vi "EC_Applied_XYZ_MM_BR_RES_2_NC_GR_pxi_Acc3_preset.vi"() -> ()   [LabVIEW 2009]
uses:
  <vilib>/Utility/file.llb/Read From Spreadsheet File (I64).vi
  <vilib>/Utility/file.llb/Read From Spreadsheet File (string).vi
  <vilib>/Instr/_visa.llb/VISA Configure Serial Port (Instr).vi
  <vilib>/Utility/file.llb/Write To Spreadsheet File (I64).vi
  <vilib>/Utility/file.llb/Write To Spreadsheet File (string).vi
panel:
  out "R Velocity MVdeg/sec":dbl format="%.3f"
  out "R Position MV deg":dbl
  out "Z Velocity MV mm/sec":dbl format="%.3f"
  out "Z Position MV mm":dbl
  out "Y Velocity MV mm/sec":dbl format="%.3f"
  out "Y Position MV mm":dbl
  out "X Velocity MV mm/sec":dbl format="%.3f"
  out "X Position MV mm":dbl
  out "Presets":i32[][](array[numeric])
  in  "stop":bool
  in  "Tab Control 3":enum32{"Status", "Reset"}(tab)
  out "Y in Range":bool
  out "Y Scan":bool
  out "Y in Motion":bool
  out "Y Backlash corr":bool
  out "X  in Range":bool
  out "X Scan":bool
  out "X  in Motion":bool
  out "X Backlash corr":bool
  out "Z in Range":bool
  out "Z Scan":bool
  out "Z in Motion":bool
  out "Z Backlash corr":bool
  out "R in Range":bool
  out "R Scan":bool
  out "R in Motion":bool
  out "R Backlash corr":bool
  out "X Ready":bool
  out "Y Ready":bool
  out "Z Ready":bool
  out "R Ready":bool
  in  "Reset Y Position mm":dbl
  out "Reset Y Motor Steps":i32
  in  "Reset X Position mm":dbl
  out "Reset X Motor Steps":i32
  in  "Reset Z Position mm":dbl
  out "Reset Z Motor Steps":i32
  in  "Reset R Position deg":dbl
  out "Reset R Motor Steps":i32
  in  "Reset":bool
  in  "Tab Control 2":enum32{"mm", "step"}(tab)
  in  "X Scan Length SP mm":dbl
  in  "X Scan Velocity SP mm/sec":dbl
  in  "X Scan set":bool
  in  "Y Scan Length SP mm":dbl
  in  "Y Scan Velocity SP mm/sec":dbl
  in  "Y Scan set":bool
  in  "Z Scan Length SP mm":dbl
  in  "Z Scan Velocity SP mm/sec":dbl
  in  "Z Scan set":bool
  in  "R Scan Length SP deg":dbl
  in  "R Scan Velocity SP deg/sec":dbl
  in  "R Scan set":bool
  in  "X Scan Velocity SP steps/sec":i32=1 min=1 max=102400 step=1
  in  "X Scan Length SP steps":i32 min=-2304000 max=2304000 step=100
  out "X Scan length MV mm":dbl
  out "X Scan velocity MV mm/sec":dbl format="%#_6f"
  in  "Y Scan Velocity SP steps/sec":i32=1 min=1 max=102400 step=1
  in  "Y Scan Length SP steps":i32 min=-2304000 max=2304000 step=100
  out "Y Scan length MV mm":dbl
  out "Y Scan velocity MV mm/sec":dbl format="%#_6f"
  in  "Z Scan Velocity SP steps/sec":i32=1 min=1 max=102400 step=1
  in  "Z Scan Length SP steps":i32 min=-5120000 max=97280000 step=100
  out "Z Scan length MV mm":dbl
  out "Z Scan velocity MV mm/sec":dbl format="%#_6f"
  in  "R Scan Velocity SP steps/sec":i32=1 min=1 max=102400 step=1
  in  "R Scan Length SP steps":i32 min=-6144000 max=0 step=100
  out "R Scan length MV deg":dbl
  out "R Scan velocity MV deg/sec":dbl format="%#_6f"
  out "atan Y/Z":dbl
  in  "Tab Control":enum32{"mm", "preset", "step"}(tab)
  in  "X Position SP mm":dbl
  in  "X Velocity SP mm/sec":dbl
  in  "X Move Set":bool
  in  "Y Move Set":bool
  in  "Y Position SP mm":dbl
  in  "Y Velocity SP mm/sec":dbl
  in  "Z Position SP mm":dbl
  in  "Z Velocity SP mm/sec":dbl
  in  "Z Move Set":bool
  in  "R Position SP deg":dbl
  in  "R Velocity SP deg/sec":dbl
  in  "R Move Set":bool
  in  "Add Button":bool
  in  "String":string
  in  "Delete Button":bool
  in  "Preset positions":i32(ring) items=["ZERO", "Default", "CDOSE", "QMS", "test", "test2", "test3"]
  in  "Set Button":bool
  in  "X Velocity SP step/sec":i32 min=1 max=10000
  in  "Y Velocity SP step/sec":i32 min=1 max=10000
  in  "Z Velocity SP step/sec":i32 min=1 max=10000
  in  "R Velocity SP step/sec":i32 min=1 max=10000
  in  "Y Step SP":i32=-20000 min=-2304000 max=2304000 step=500
  in  "X Step SP":i32=-20000 min=-1000000 max=1000000 step=500
  in  "Z Step SP":i32=-20000 min=0 max=102400000 step=500
  in  "R Step SP":i32=-20000 min=-6144000 max=0 step=500
  out "X Step PV":i32 max=2000
  out "Y Step PV":i32 max=2000
  out "Z Step PV":i32 max=2000
  out "R Step PV":i32 max=2000
  in  "Clear ZY":bool
  out "ZY Graph":cluster{"Y":dbl[], "Y":dbl[]}[](graph)
  out "ZR Graph":cluster{"Y":dbl[], "Y":dbl[]}[](graph)
  out "XY Graph":cluster{"Y":dbl[], "Y":dbl[]}[](graph)
  out "X Scan Duration":dbl
  out "Y Scan Duration":dbl
  out "Z Scan Duration":dbl
  out "R Scan Duration":dbl
  out "R Backlash steps/sec":i32
  out "R Backlash":i32
  out "R Holding Current %":i32
  out "R Run Current %":i32
  out "R offset deg":dbl
  out "R deg/rev":dbl
  out "R steps/rev":u32
  out "R velocity PV step/sec":i32
  out "R MINPOS":i32=-94296
  out "R MAXPOS":i32=-34296
  out "R COM PORT":refnum<visa-resource-name>="COM5"
  in  "R Scan OK":bool
  in  "R Go":bool
  out "R Position deg PV":dbl
  out "Z COM PORT":refnum<visa-resource-name>="COM5"
  out "Z Backlash steps/sec":i32
  out "Z Backlash":i32
  out "Z Holding Current %":i32
  out "Z Run Current %":i32
  out "Z offset mm":dbl
  out "Z mm/rev":dbl
  out "Z steps/rev":u32
  out "Z  velocity PV step/sec":i32
  out "Z MINPOS":i32=-94296
  out "Z MAXPOS":i32=-34296
  in  "Z Scan OK":bool
  in  "Z Go":bool
  out "Z Position mm PV":dbl
  out "X Position mm PV":dbl
  out "X velocity PV step/sec":i32
  in  "X Scan OK":bool
  in  "X Go":bool
  out "X Backlash steps/sec":i32
  out "X Backlash":i32
  out "X Holding Current %":i32
  out "X Run Current %":i32
  out "X offset mm":dbl
  out "X mm/rev":dbl
  out "X steps/rev":u32
  out "X MAXPOS":i32=-34296
  out "X MINPOS":i32=-94296
  out "X COM PORT":refnum<visa-resource-name>="COM5"
  out "Y Backlash steps/sec":i32
  out "Y Backlash":i32
  out "Y Holding Current %":i32
  out "Y Run Current %":i32
  in  "Scan Cancel":bool
  out "Y Position mm PV":dbl
  out "Y offset mm":dbl
  out "Y mm/rev":dbl
  out "Y steps/rev":u32
  out "Y velocity PV step/sec":i32
  in  "Y Scan OK":bool
  in  "Scan Go":bool
  in  "Stop":bool
  in  "Y Go":bool
  out "Y MINPOS":i32=-94296
  out "Y MAXPOS":i32=-34296
  out "Y COM PORT":refnum<visa-resource-name>="COM5"
  # "Current position"
  # "Goto position"
  # "RX"
  # "RY"
  # "RZ"
  # "RR"
  # "L"
  # "M"
  # "B"
  # "S"
  # "R"
  # "Preset position"
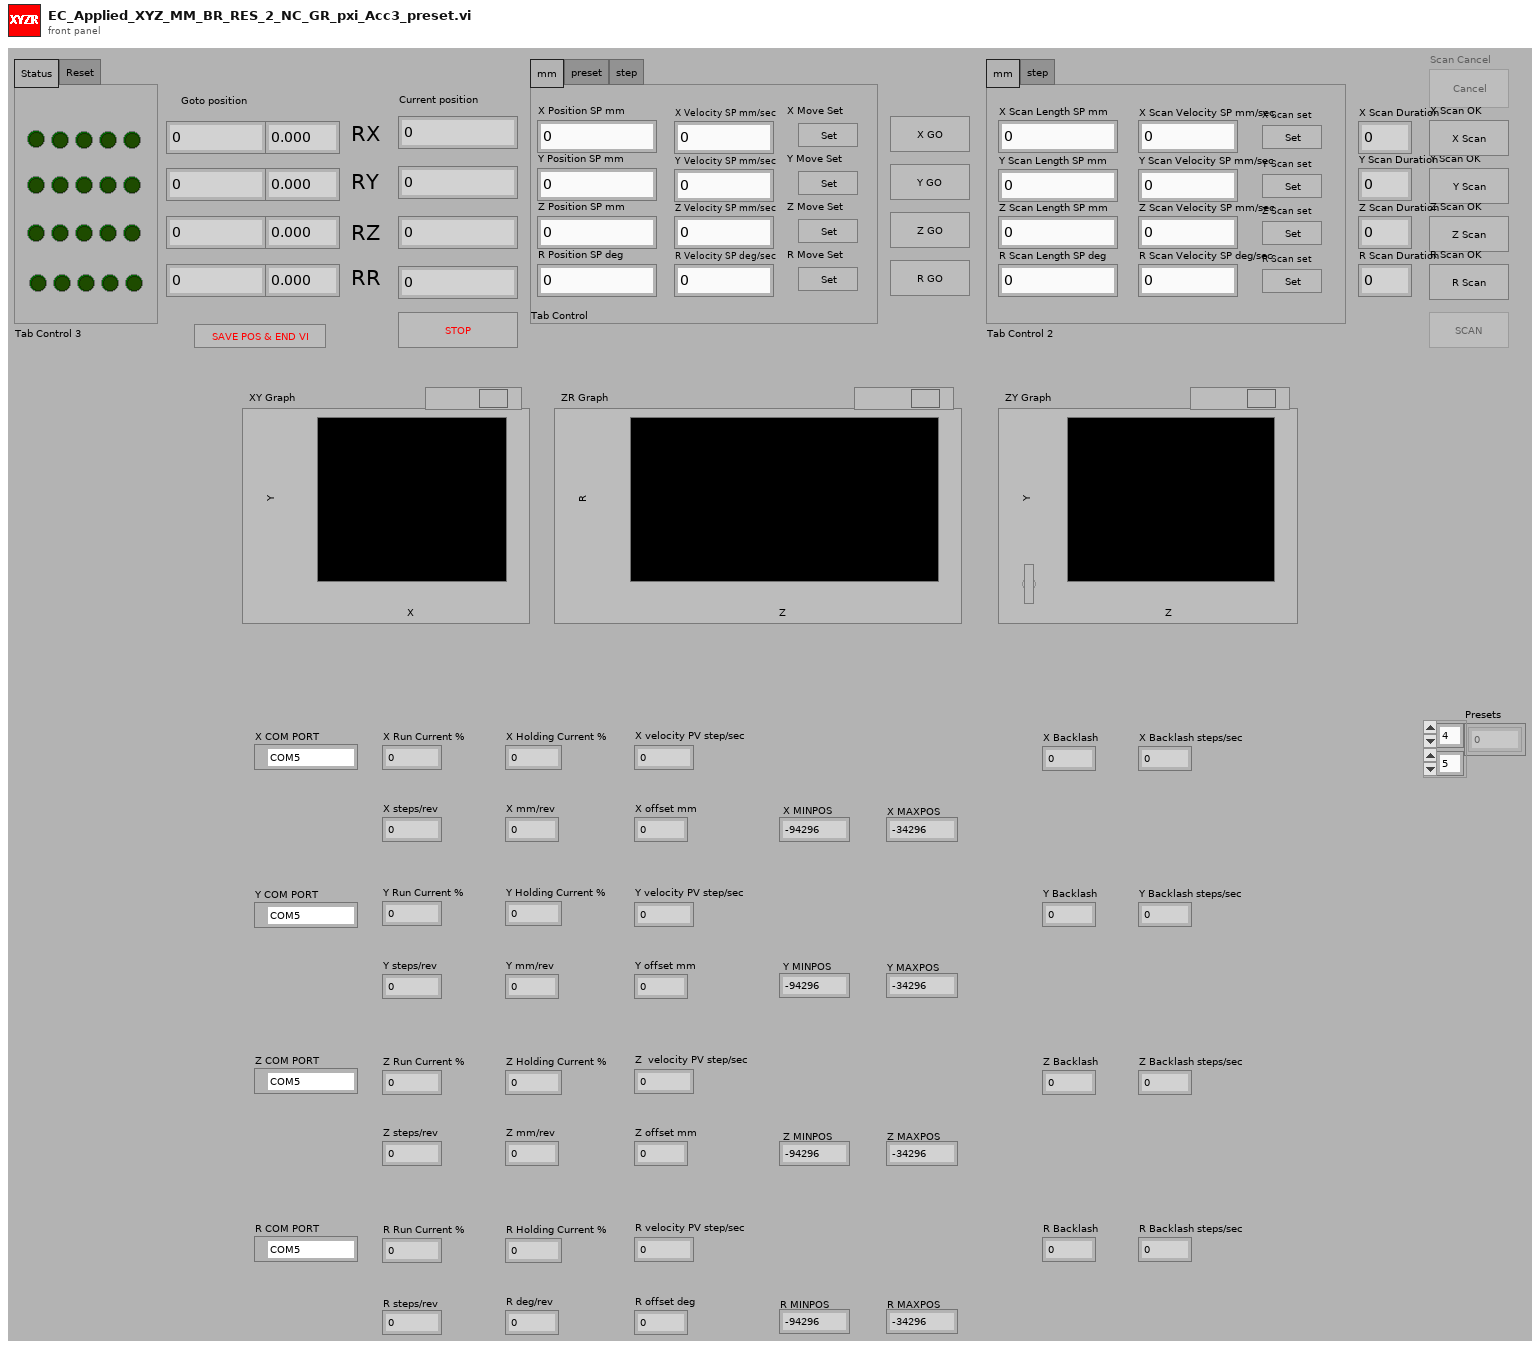
[diagram p1: front panel]
types:
  T1 = enum16{"Stop", "Reset", "Run Current", "Holding Current", "Accel Rate", "Decel Rate", "Move to Relative Position", "Move to Absolute Position", "Echo Mode", "Print Parameter", "Send String", "Microstep Resolution", "Set Current Position", "Max Velocity"}
  T2 = enum8{"Enabled", "Disabled", "Disabled and Grayed Out"}
  T3 = enum16{"Power-up Signature", "Accel Rate", "Accel Max", "Bit Rate", "Buffer Status", "Change Current", "Commence Jogging", "Change Jog Speed", "Continue", "Define Address", "Distance for FC,FM,FO,FY", "Decel Rate", "Distance or Position", "Define Limits", "Encoder Deadband", "Encoder Function", "Encoder Position", "Encoder Ratio", "Feed to Length with Speed Change", "Feed to Length", "Feed to Sensor with Mask Dist", "Feed to Length & Set Output", "Feed to Position", "Feed to Sensor", "Feed to Sensor w/safety", "Follow Handwheel", "Immediate Distance?", "Immediate Encoder?", "Immediate Low Output", "Immediate High Output", "Immediate Position?", "Input Status?", "Jog Accel/Decel", "Jog Disable", "Jog Enable", "Jog Speed", "Motor Disable", "Motor Enable", "Microstep Resolution", "Power up Current", "Power up Mode", "Pause", "Request Status", "Revision Level?", "Seek Home", "Stop Jogging", "Stop & Kill Buffer", "Set Output", "Set ABS Position", "Send String", "Stop", "Velocity for Speed Change", "Velocity Setting", "Wait for Input", "Wait Time"}
  T4 = cluster{"first row[0]":i64, "first row[1]":i64, "first row[2]":i64, "first row[3]":i64, "first row[4]":i64, "first row[5]":i64, "first row[6]":i64, "first row[7]":i64, "first row[8]":i64}
  T5 = cluster{"Value[0]":i32, "Value[1]":i32, "Value[2]":i32, "Value[3]":i32, "Value[4]":i32, "Value[5]":i32, "Value[6]":i32, "Value[7]":i32, "Value[8]":i32}
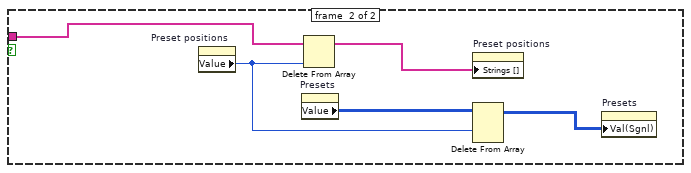
[diagram p2: hidden frame]
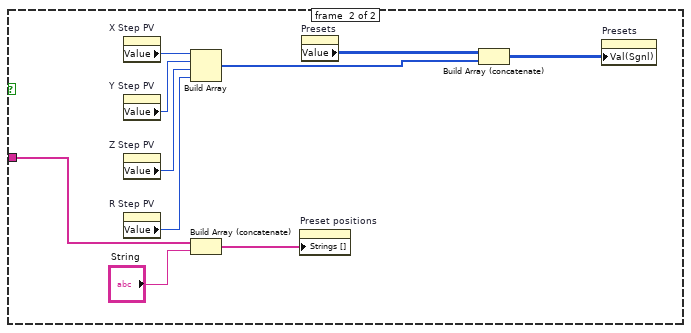
[diagram p3: hidden frame]
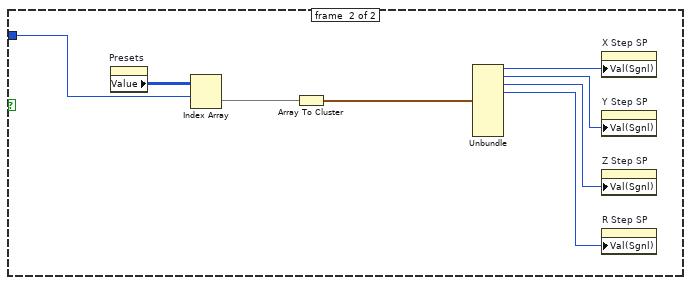
[diagram p4: hidden frame]
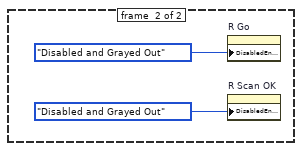
[diagram p5: hidden frame]
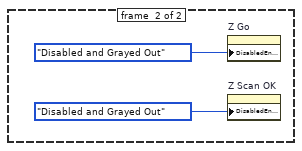
[diagram p8: hidden frame]
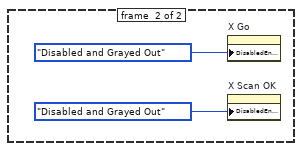
[diagram p11: hidden frame]
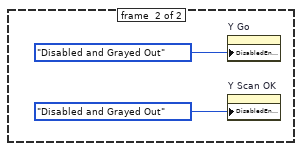
[diagram p14: hidden frame]
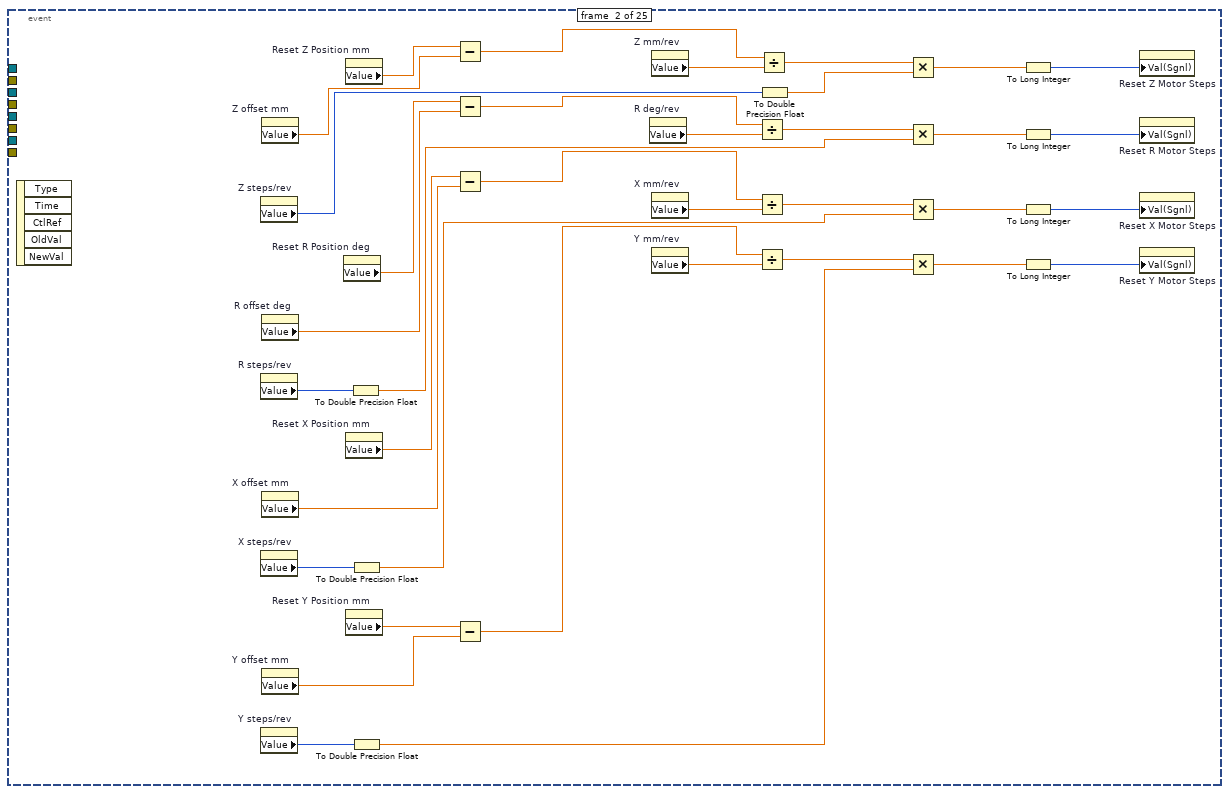
[diagram p17: hidden frame]
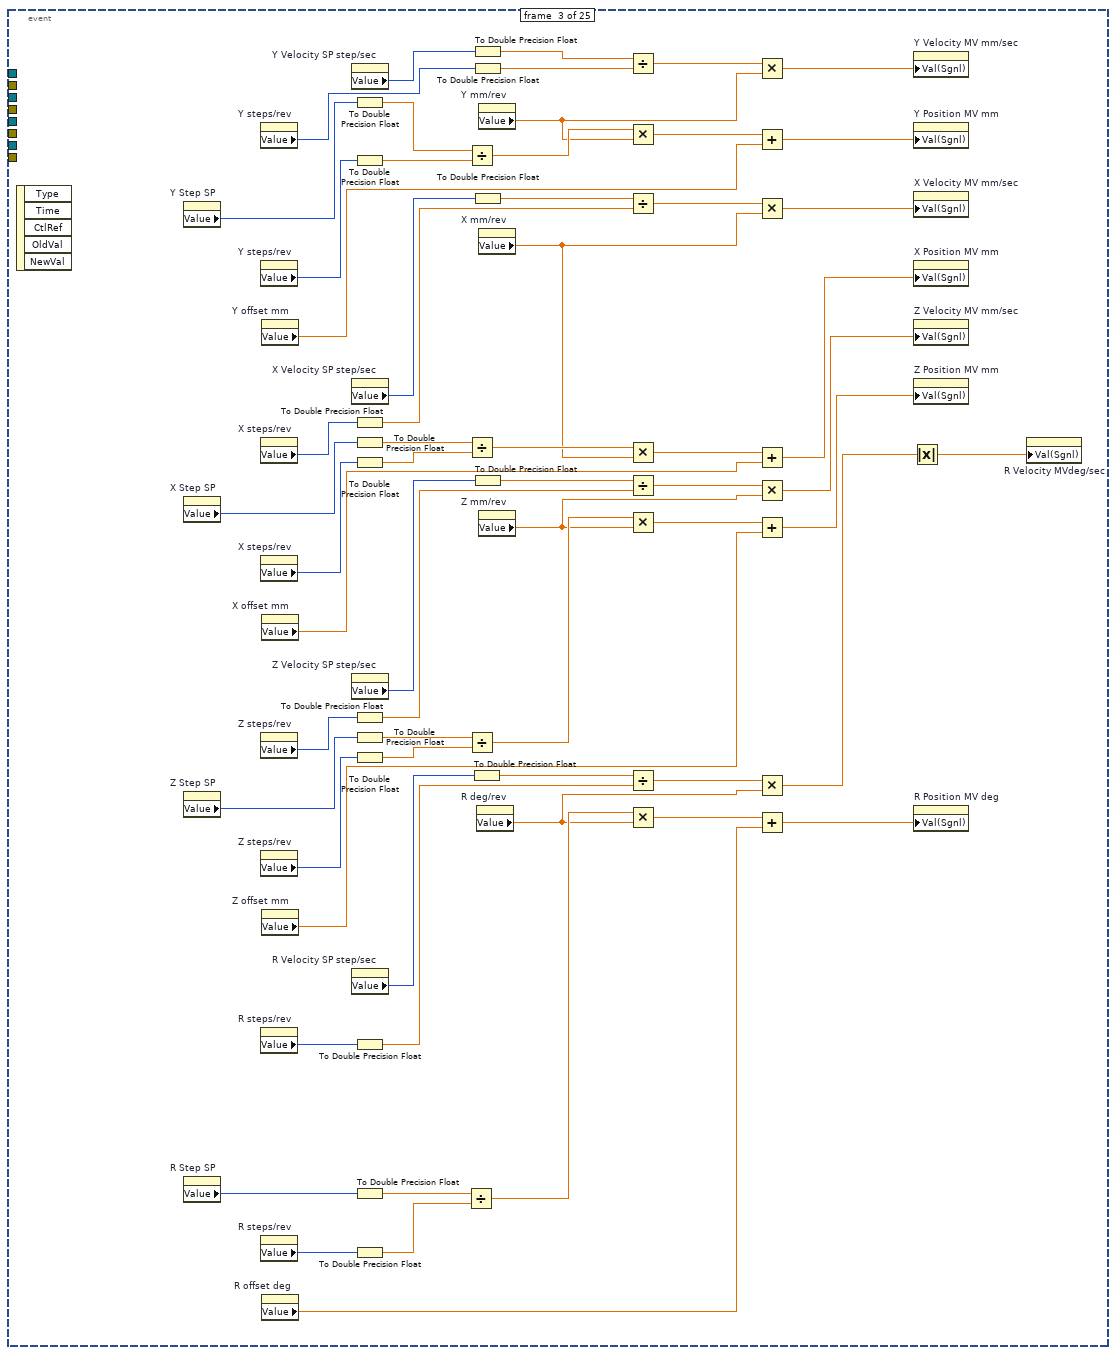
[diagram p18: hidden frame]
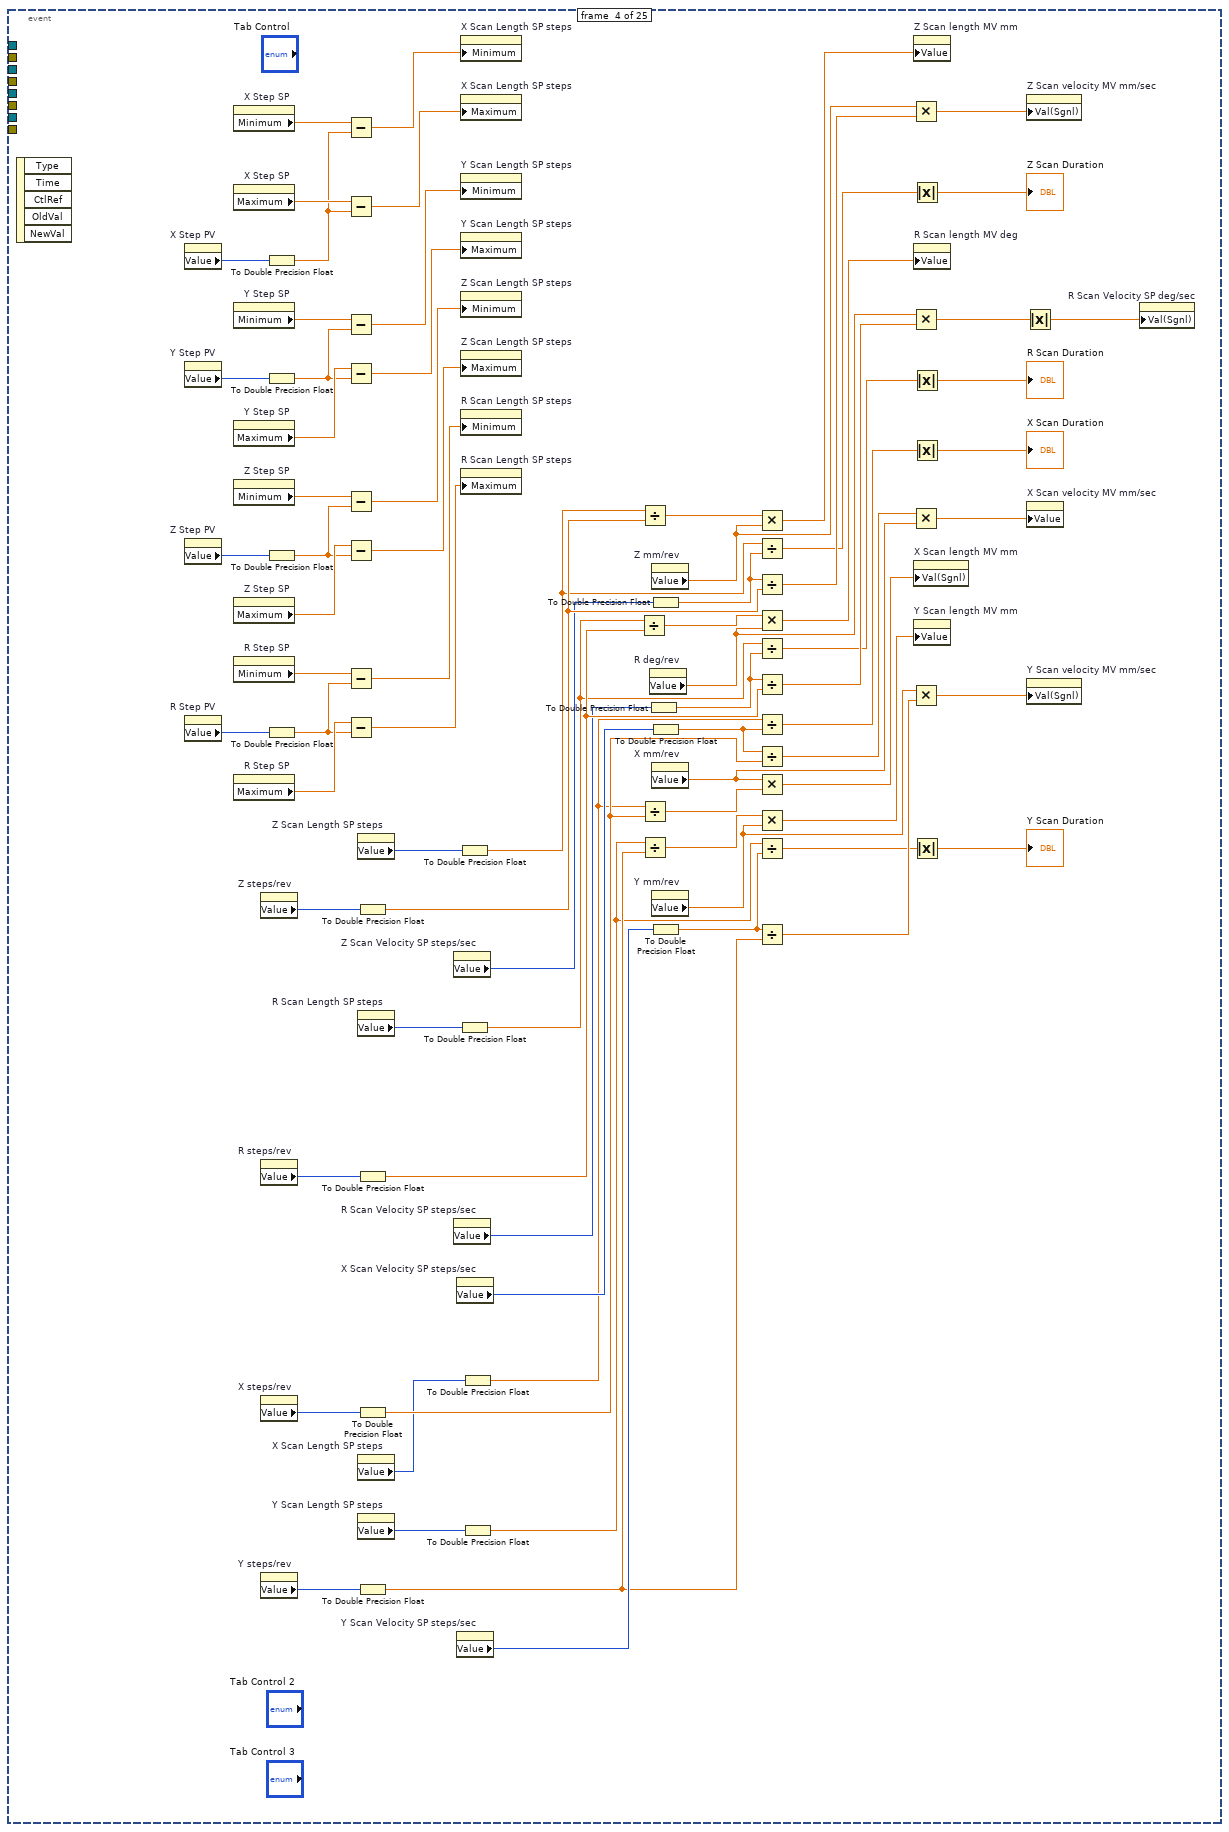
[diagram p19: hidden frame]
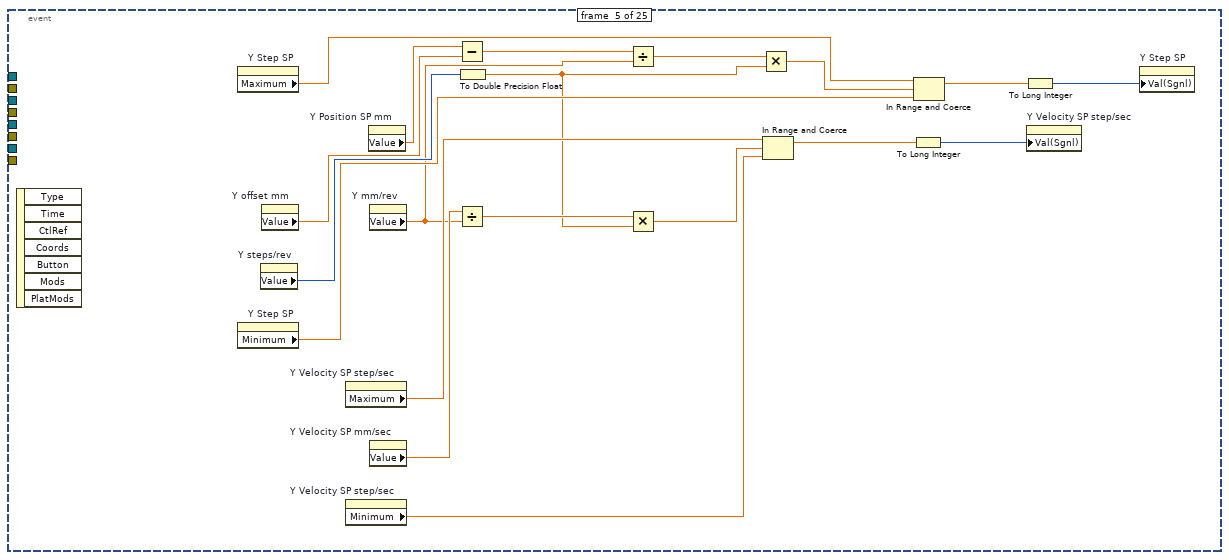
[diagram p20: hidden frame]
diagram:
  w6 = 0 ("dimension size")
  n1 = flat-sequence {
    tunnel: [w99] -> w40
    tunnel: [w98] -> w39
    tunnel: [w107] -> w56
    tunnel: [w109] -> w54
    tunnel: w40 -> [w108]
    tunnel: w39 -> [w110]
    tunnel: w56 -> [w114]
    tunnel: [w115] -> w55
    tunnel: w54 -> [w113]
    tunnel: [w116] -> w53
    tunnel: [w127] -> w69
    tunnel: [w129] -> w68
    tunnel: w55 -> [w128]
    tunnel: w53 -> [w123]
    tunnel: w69 -> [w136]
    tunnel: [w135] -> w67
    tunnel: w68 -> [w133]
    tunnel: [w134] -> w66
    tunnel: [w146] -> w65
    tunnel: [w147] -> w64
    tunnel: w67 -> [w145]
    tunnel: w66 -> [w144]
    tunnel: w65 -> [w157]
    tunnel: w64 -> [w156]
    tunnel: [w159] -> w63
    tunnel: [w158] -> w62
    tunnel: [w153] -> w61
    tunnel: [w166] -> w57
    tunnel: [w167] -> w58
    tunnel: w63 -> [w167]
    tunnel: w62 -> [w166]
    tunnel: w61 -> [w164]
    frame #0 {
      w106 = refnum<visa-resource-name> "COM11" ("COM PORT")
      w104 = u16 0 items=["None", "XON/XOFF", "RTS/CTS", "XON/XOFF & RTS/CTS", "DTR/DSR", "XON/XOFF & DTR/DSR"] ("flow control (0:none)")
      w103 = u16 10 items=["1.0"=10, "1.5"=15, "2.0"=20] ("stop bits (10: 1 bit)")
      # "Stop bits"
      n2 = call-poly "VISA Configure Serial Port"("VISA resource name"=w106, "timeout (10sec)"=u32 10000, "baud rate (9600)"=u32 9600, "data bits (8)"=u16 8, "parity (0:none)"=enum16{"None", "Odd", "Even", "Mark", "Space"}."None", "stop bits (10: 1 bit)"=w103, "flow control (0:none)"=w104) -> ("VISA resource name out"=w99:refnum<visa-resource-name>, "error out"=w98:errorcluster)  [unwired: 7 in]
      "R COM PORT" <- w106
    }
    frame #1 {
      n3 = call "mDrive Send Command.vi"("error in (no error)"=w110, "Extra"="EM=2", "Command"=T1."Send String", "VISA resource name"=w108) -> ("error out"=w109:errorcluster, "VISA resource name out"=w107:refnum<visa-resource-name>)  [unwired: 3 in, 1 out]
    }
    frame #2 {
      # "pr=1000000"
      n4 = Number To Decimal String(number=100000) -> (decimal integer string=w118:string)  [unwired: 1 in]
      n5 = call "mDrive Send Command.vi"("error in (no error)"=w113, "Extra"=w118, "Command"=T1."Accel Rate", "VISA resource name"=w114) -> ("error out"=w117:errorcluster, "VISA resource name out"=w122:refnum<visa-resource-name>)  [unwired: 3 in, 1 out]
      n6 = call "mDrive Send Command.vi"("error in (no error)"=w117, "Extra"=w118, "Command"=T1."Decel Rate", "VISA resource name"=w122) -> ("error out"=w116:errorcluster, "VISA resource name out"=w115:refnum<visa-resource-name>)  [unwired: 3 in, 1 out]
    }
    frame #3 {
      # "Run Current %"
      n7 = property on="R Run Current %" class="DigNum (strict)"() -> ("Value"=w125:i32)  [unwired: 2 in, 2 out]
      n8 = Number To Decimal String(number=w125) -> (decimal integer string=w126:string)  [unwired: 1 in]
      n9 = call "mDrive Send Command.vi"("error in (no error)"=w123, "Extra"=w126, "Command"=T1."Run Current", "VISA resource name"=w128) -> ("error out"=w129:errorcluster, "VISA resource name out"=w127:refnum<visa-resource-name>)  [unwired: 3 in, 1 out]
    }
    frame #4 {
      # "Holding Current %"
      n10 = property on="R Holding Current %" class="DigNum (strict)"() -> ("Value"=w131:i32)  [unwired: 2 in, 2 out]
      n11 = Number To Decimal String(number=w131) -> (decimal integer string=w132:string)  [unwired: 1 in]
      n12 = call "mDrive Send Command.vi"("error in (no error)"=w133, "Extra"=w132, "Command"=T1."Holding Current", "VISA resource name"=w136) -> ("error out"=w134:errorcluster, "VISA resource name out"=w135:refnum<visa-resource-name>)  [unwired: 3 in, 1 out]
    }
    frame #5 {
      # "Print Velocity Max"
      # "Velocity Max"
      n13 = property on="R Velocity SP step/sec" class="DigNum (strict)"() -> ("Value"=w143:i32)  [unwired: 2 in, 2 out]
      n14 = Number To Decimal String(number=w143) -> (decimal integer string=w142:string)  [unwired: 1 in]
      n15 = call "mDrive Send Command.vi"("error in (no error)"=w144, "Extra"=w142, "Command"=T1."Max Velocity", "VISA resource name"=w145) -> ("error out"=w140:errorcluster, "VISA resource name out"=w150:refnum<visa-resource-name>)  [unwired: 3 in, 1 out]
      n16 = call "mDrive Send Command.vi"("error in (no error)"=w140, "Extra"="VM", "Command"=T1."Print Parameter", "VISA resource name"=w150) -> ("error out"=w147:errorcluster, "read buffer"=w148:string, "VISA resource name out"=w146:refnum<visa-resource-name>)  [unwired: 3 in]
      n17 = Decimal String To Number(string=w148, offset=0) -> (number=w141:i32)  [unwired: 1 in, 1 out]
      n18 = property on="R velocity PV step/sec" class="DigNum (strict)"("Val(Sgnl)"=w141) -> ()  [unwired: 2 in, 2 out]
    }
    frame #6 {
      # "PRINT POSITION"
      n19 = call "mDrive Send Command.vi"("error in (no error)"=w156, "Extra"="P", "Command"=T1."Print Parameter", "VISA resource name"=w157) -> ("error out"=w158:errorcluster, "read buffer"=w155:string, "VISA resource name out"=w159:refnum<visa-resource-name>)  [unwired: 3 in]
      n20 = Decimal String To Number(string=w155, offset=0) -> (number=w153:i32)  [unwired: 1 in, 1 out]
    }
    frame #7 {
      n21 = property on="R Step SP" class="DigNum (strict)"("Val(Sgnl)"=w164) -> ()  [unwired: 2 in, 2 out]
      n22 = property on="R Step SP" class="DigNum (strict)"() -> ("Maximum"=w163:dbl)  [unwired: 2 in, 2 out]
      n23 = property on="R Step SP" class="DigNum (strict)"() -> ("Minimum"=w162:dbl)  [unwired: 2 in, 2 out]
      n24 = To Long Integer(number=w163) -> (32bit integer=w160:i32)
      "R MAXPOS" <- w160
      n25 = To Long Integer(number=w162) -> (32bit integer=w161:i32)
      "R MINPOS" <- w161
      n26 = In Range and Coerce(upper limit=w160, x=w164, lower limit=w161) -> (In Range?=w165:bool)  [unwired: 1 out]
      n27 = property on="R in Range" class="Bool (strict)"("Val(Sgnl)"=w165) -> ()  [unwired: 2 in, 2 out]
    }
  }
  n28 = flat-sequence {
    frame #0 {
      w173 = -3.0 ("R deg/rev")
      w171 = u32 20000 ("step/rev")
      w175 = 10000 ("Value (Signaling)")
      n29 = To Double Precision Float(number=w175) -> (double precision float=w177:dbl)
      n30 = To Double Precision Float(number=w171) -> (double precision float=w172:dbl)
      n31 = property on="R Velocity SP step/sec" class="DigNum (strict)"("Val(Sgnl)"=w175) -> ()  [unwired: 2 in, 2 out]
      n32 = property on="R Velocity SP step/sec" class="DigNum (strict)"("Minimum"=1.0 ("Data Entry Limits:Minimum")) -> ()  [unwired: 2 in, 2 out]
      n33 = Divide(x=w177, y=w172) -> (x/y=w176:dbl)
      n34 = property on="R Velocity SP step/sec" class="DigNum (strict)"("Maximum"=w177) -> ()  [unwired: 2 in, 2 out]
      n35 = Multiply(x=w176, y=w173) -> (x*y=w174:dbl)
      n36 = Absolute Value(x=w174) -> (abs(x)=w168:dbl)
      n37 = property on="R Velocity SP deg/sec" class="DigNum (strict)"("Val(Sgnl)"=w168) -> ()  [unwired: 2 in, 2 out]
      "R offset deg" <- 0.0 ("R offset deg")
      "R deg/rev" <- w173
      "R steps/rev" <- w171
    }
  }
  n38 = flat-sequence {
    frame #0 {
      w179 = 5.08 ("Z mm/rev")
      w178 = u32 20000 ("step/rev")
      w180 = 10000 ("Value (Signaling)")
      n39 = To Double Precision Float(number=w180) -> (double precision float=w184:dbl)
      n40 = To Double Precision Float(number=w178) -> (double precision float=w183:dbl)
      n41 = property on="Z Velocity SP step/sec" class="DigNum (strict)"("Val(Sgnl)"=w180) -> ()  [unwired: 2 in, 2 out]
      n42 = property on="Z Velocity SP step/sec" class="DigNum (strict)"("Minimum"=1.0 ("Data Entry Limits:Minimum")) -> ()  [unwired: 2 in, 2 out]
      n43 = Divide(x=w184, y=w183) -> (x/y=w181:dbl)
      n44 = property on="Z Velocity SP step/sec" class="DigNum (strict)"("Maximum"=w184) -> ()  [unwired: 2 in, 2 out]
      n45 = Multiply(x=w181, y=w179) -> (x*y=w182:dbl)
      n46 = property on="Z Velocity SP mm/sec" class="DigNum (strict)"("Val(Sgnl)"=w182) -> ()  [unwired: 2 in, 2 out]
      "Z offset mm" <- 0.0 ("Z offset mm")
      "Z mm/rev" <- w179
      "Z steps/rev" <- w178
    }
  }
  n47 = flat-sequence {
    frame #0 {
      n48 = property on="X Backlash corr" class="Bool (strict)"("Val(Sgnl)"=FALSE ("Value (Signaling)")) -> ()  [unwired: 2 in, 2 out]
      n49 = property on="Y Backlash corr" class="Bool (strict)"("Val(Sgnl)"=FALSE ("Value (Signaling)")) -> ()  [unwired: 2 in, 2 out]
      n50 = property on="R Backlash corr" class="Bool (strict)"("Val(Sgnl)"=FALSE ("Value (Signaling)")) -> ()  [unwired: 2 in, 2 out]
      n51 = property on="Z Backlash corr" class="Bool (strict)"("Val(Sgnl)"=FALSE ("Value (Signaling)")) -> ()  [unwired: 2 in, 2 out]
      "Z Backlash steps/sec" <- 1000 ("Z Backlash steps/sec")
      "Z Backlash" <- -12800 ("Z Backlash")
      "X Backlash steps/sec" <- 10000 ("Value (Signaling)")
      "X Backlash" <- 5000 ("Backlash2")
      "Y Backlash" <- 5120 ("Backlash2")
      "Y Backlash steps/sec" <- 1000 ("Value (Signaling)")
      "R Backlash steps/sec" <- 6400 ("R Backlash steps/sec")
      "R Backlash" <- -12800 ("R Backlash")
    }
  }
  n52 = flat-sequence {
    frame #0 {
      "Z Holding Current %" <- 50 ("Z Holding Current %")
      "Z Run Current %" <- 100 ("Z Run Current %")
      "X Run Current %" <- 100 ("Run Current %")
      "X Holding Current %" <- 50 ("Holding Current %")
      "Y Run Current %" <- 100 ("Run Current %")
      "Y Holding Current %" <- 50 ("Holding Current %")
      "R Holding Current %" <- 50 ("R Holding Current %")
      "R Run Current %" <- 100 ("R Run Current %")
    }
  }
  n53 = flat-sequence {
    frame #0 {
      n54 = property on="Y Scan" class="Bool (strict)"("Val(Sgnl)"=FALSE ("Value (Signaling)")) -> ()  [unwired: 2 in, 2 out]
      n55 = property on="X Scan Velocity SP mm/sec" class="DigNum (strict)"("Val(Sgnl)"=0.1 ("Value (Signaling)")) -> ()  [unwired: 2 in, 2 out]
      n56 = property on="Z Scan" class="Bool (strict)"("Val(Sgnl)"=FALSE ("Value (Signaling)")) -> ()  [unwired: 2 in, 2 out]
      n57 = property on="X Scan" class="Bool (strict)"("Val(Sgnl)"=FALSE ("Value (Signaling)")) -> ()  [unwired: 2 in, 2 out]
      n58 = property on="Z Scan Velocity SP mm/sec" class="DigNum (strict)"("Val(Sgnl)"=0.1 ("Value (Signaling)")) -> ()  [unwired: 2 in, 2 out]
      n59 = property on="R Velocity SP deg/sec" class="DigNum (strict)"("Val(Sgnl)"=0.1 ("Value (Signaling)")) -> ()  [unwired: 2 in, 2 out]
      n60 = property on="R Scan" class="Bool (strict)"("Val(Sgnl)"=FALSE ("Value (Signaling)")) -> ()  [unwired: 2 in, 2 out]
      n61 = property on="Y Scan Velocity SP mm/sec" class="DigNum (strict)"("Val(Sgnl)"=0.1 ("Value (Signaling)")) -> ()  [unwired: 2 in, 2 out]
      n62 = property on="Scan Go" class="Bool"("DisabledEnum"=T2."Disabled and Grayed Out" ("Disabled")) -> ()  [unwired: 2 in, 2 out]
      n63 = property on="Scan Cancel" class="Bool"("DisabledEnum"=T2."Disabled and Grayed Out" ("Disabled")) -> ()  [unwired: 2 in, 2 out]
    }
  }
  n64 = flat-sequence {
    frame #0 {
      w219 = 0.21167 ("MM/rev")
      w222 = u32 20000 ("step/rev")
      w217 = 10000 ("Value (Signaling)")
      # "a=1000000"
      n65 = property on="X Velocity SP step/sec" class="DigNum (strict)"("Minimum"=1.0 ("Data Entry Limits:Minimum")) -> ()  [unwired: 2 in, 2 out]
      n66 = To Double Precision Float(number=w217) -> (double precision float=w223:dbl)
      n67 = To Double Precision Float(number=w222) -> (double precision float=w221:dbl)
      n68 = property on="X Velocity SP step/sec" class="DigNum (strict)"("Val(Sgnl)"=w217) -> ()  [unwired: 2 in, 2 out]
      n69 = Divide(x=w223, y=w221) -> (x/y=w218:dbl)
      n70 = property on="X Velocity SP step/sec" class="DigNum (strict)"("Maximum"=w223) -> ()  [unwired: 2 in, 2 out]
      n71 = Multiply(x=w218, y=w219) -> (x*y=w220:dbl)
      n72 = property on="X Velocity SP mm/sec" class="DigNum (strict)"("Val(Sgnl)"=w220) -> ()  [unwired: 2 in, 2 out]
      "X offset mm" <- 0.0 ("offset")
      "X steps/rev" <- w222
      "X mm/rev" <- w219
    }
  }
  n73 = flat-sequence {
    frame #0 {
      w228 = 0.21167 ("MM/rev")
      w231 = u32 20000 ("step/rev")
      w226 = 10000 ("Value (Signaling)")
      n74 = To Double Precision Float(number=w226) -> (double precision float=w232:dbl)
      n75 = To Double Precision Float(number=w231) -> (double precision float=w230:dbl)
      n76 = property on="Y Velocity SP step/sec" class="DigNum (strict)"("Minimum"=1.0 ("Data Entry Limits:Minimum")) -> ()  [unwired: 2 in, 2 out]
      n77 = property on="Y Velocity SP step/sec" class="DigNum (strict)"("Val(Sgnl)"=w226) -> ()  [unwired: 2 in, 2 out]
      n78 = Divide(x=w232, y=w230) -> (x/y=w227:dbl)
      n79 = property on="Y Velocity SP step/sec" class="DigNum (strict)"("Maximum"=w232) -> ()  [unwired: 2 in, 2 out]
      n80 = Multiply(x=w227, y=w228) -> (x*y=w229:dbl)
      n81 = property on="Y Velocity SP mm/sec" class="DigNum (strict)"("Val(Sgnl)"=w229) -> ()  [unwired: 2 in, 2 out]
      "Y offset mm" <- 0.0 ("offset")
      "Y steps/rev" <- w231
      "Y mm/rev" <- w228
    }
  }
  n82 = flat-sequence {
    tunnel: [w235] -> w42
    tunnel: [w236] -> w41
    tunnel: [w246] -> w48
    tunnel: [w245] -> w46
    tunnel: w42 -> [w247]
    tunnel: w41 -> [w244]
    tunnel: w48 -> [w257]
    tunnel: [w252] -> w47
    tunnel: w46 -> [w256]
    tunnel: [w256] -> w45
    tunnel: [w261] -> w78
    tunnel: [w263] -> w77
    tunnel: w47 -> [w262]
    tunnel: w45 -> [w264]
    tunnel: w78 -> [w271]
    tunnel: [w270] -> w76
    tunnel: w77 -> [w268]
    tunnel: [w269] -> w75
    tunnel: [w281] -> w74
    tunnel: [w282] -> w73
    tunnel: w76 -> [w280]
    tunnel: w75 -> [w279]
    tunnel: w74 -> [w292]
    tunnel: w73 -> [w291]
    tunnel: [w294] -> w72
    tunnel: [w293] -> w71
    tunnel: [w288] -> w70
    tunnel: [w301] -> w59
    tunnel: [w302] -> w60
    tunnel: w72 -> [w302]
    tunnel: w71 -> [w301]
    tunnel: w70 -> [w299]
    frame #0 {
      w243 = refnum<visa-resource-name> "COM10" ("COM PORT")
      w241 = u16 0 items=["None", "XON/XOFF", "RTS/CTS", "XON/XOFF & RTS/CTS", "DTR/DSR", "XON/XOFF & DTR/DSR"] ("flow control (0:none)")
      w240 = u16 10 items=["1.0"=10, "1.5"=15, "2.0"=20] ("stop bits (10: 1 bit)")
      # "Stop bits"
      n83 = call-poly "VISA Configure Serial Port"("VISA resource name"=w243, "timeout (10sec)"=u32 10000, "baud rate (9600)"=u32 9600, "data bits (8)"=u16 8, "parity (0:none)"=enum16{"None", "Odd", "Even", "Mark", "Space"}."None", "stop bits (10: 1 bit)"=w240, "flow control (0:none)"=w241) -> ("VISA resource name out"=w235:refnum<visa-resource-name>, "error out"=w236:errorcluster)  [unwired: 7 in]
      "Z COM PORT" <- w243
    }
    frame #1 {
      n84 = call "mDrive Send Command.vi"("error in (no error)"=w244, "Extra"="EM=2", "Command"=T1."Send String", "VISA resource name"=w247) -> ("error out"=w245:errorcluster, "VISA resource name out"=w246:refnum<visa-resource-name>)  [unwired: 3 in, 1 out]
    }
    frame #2 {
      n85 = Number To Decimal String(number=1000000) -> (decimal integer string=w250:string)  [unwired: 1 in]
      n86 = call "mDrive Send Command.vi"("Extra"=w250, "Command"=T1."Accel Rate", "VISA resource name"=w257) -> ("VISA resource name out"=w255:refnum<visa-resource-name>)  [unwired: 4 in, 2 out]
      n87 = call "mDrive Send Command.vi"("Extra"=w250, "Command"=T1."Decel Rate", "VISA resource name"=w255) -> ("VISA resource name out"=w252:refnum<visa-resource-name>)  [unwired: 4 in, 2 out]
    }
    frame #3 {
      # "Run Current %"
      n88 = property on="Z Run Current %" class="DigNum (strict)"() -> ("Value"=w259:i32)  [unwired: 2 in, 2 out]
      n89 = Number To Decimal String(number=w259) -> (decimal integer string=w260:string)  [unwired: 1 in]
      n90 = call "mDrive Send Command.vi"("error in (no error)"=w264, "Extra"=w260, "Command"=T1."Run Current", "VISA resource name"=w262) -> ("error out"=w263:errorcluster, "VISA resource name out"=w261:refnum<visa-resource-name>)  [unwired: 3 in, 1 out]
    }
    frame #4 {
      # "Holding Current %"
      n91 = property on="Z Run Current %" class="DigNum (strict)"() -> ("Value"=w266:i32)  [unwired: 2 in, 2 out]
      n92 = Number To Decimal String(number=w266) -> (decimal integer string=w267:string)  [unwired: 1 in]
      n93 = call "mDrive Send Command.vi"("error in (no error)"=w268, "Extra"=w267, "Command"=T1."Holding Current", "VISA resource name"=w271) -> ("error out"=w269:errorcluster, "VISA resource name out"=w270:refnum<visa-resource-name>)  [unwired: 3 in, 1 out]
    }
    frame #5 {
      # "Velocity Max"
      n94 = property on="Z Velocity SP step/sec" class="DigNum (strict)"() -> ("Value"=w278:i32)  [unwired: 2 in, 2 out]
      n95 = Number To Decimal String(number=w278) -> (decimal integer string=w277:string)  [unwired: 1 in]
      n96 = call "mDrive Send Command.vi"("error in (no error)"=w279, "Extra"=w277, "Command"=T1."Max Velocity", "VISA resource name"=w280) -> ("error out"=w275:errorcluster, "VISA resource name out"=w285:refnum<visa-resource-name>)  [unwired: 3 in, 1 out]
      n97 = call "mDrive Send Command.vi"("error in (no error)"=w275, "Extra"="VM", "Command"=T1."Print Parameter", "VISA resource name"=w285) -> ("error out"=w282:errorcluster, "read buffer"=w283:string, "VISA resource name out"=w281:refnum<visa-resource-name>)  [unwired: 3 in]
      n98 = Decimal String To Number(string=w283, offset=0) -> (number=w276:i32)  [unwired: 1 in, 1 out]
      n99 = property on="Z  velocity PV step/sec" class="DigNum (strict)"("Val(Sgnl)"=w276) -> ()  [unwired: 2 in, 2 out]
    }
    frame #6 {
      # "PRINT POSITION"
      n100 = call "mDrive Send Command.vi"("error in (no error)"=w291, "Extra"="P", "Command"=T1."Print Parameter", "VISA resource name"=w292) -> ("error out"=w293:errorcluster, "read buffer"=w290:string, "VISA resource name out"=w294:refnum<visa-resource-name>)  [unwired: 3 in]
      n101 = Decimal String To Number(string=w290, offset=0) -> (number=w288:i32)  [unwired: 1 in, 1 out]
    }
    frame #7 {
      n102 = property on="Z Step SP" class="DigNum (strict)"("Val(Sgnl)"=w299) -> ()  [unwired: 2 in, 2 out]
      n103 = property on="Z Step SP" class="DigNum (strict)"() -> ("Maximum"=w296:dbl)  [unwired: 2 in, 2 out]
      n104 = property on="Z Step SP" class="DigNum (strict)"() -> ("Minimum"=w298:dbl)  [unwired: 2 in, 2 out]
      n105 = To Long Integer(number=w296) -> (32bit integer=w297:i32)
      "Z MAXPOS" <- w297
      n106 = To Long Integer(number=w298) -> (32bit integer=w295:i32)
      "Z MINPOS" <- w295
      n107 = In Range and Coerce(upper limit=w297, x=w299, lower limit=w295) -> (In Range?=w300:bool)  [unwired: 1 out]
      n108 = property on="Z in Range" class="Bool (strict)"("Val(Sgnl)"=w300) -> ()  [unwired: 2 in, 2 out]
    }
  }
  n109 = flat-sequence {
    tunnel: [w304] -> w38
    tunnel: [w303] -> w37
    tunnel: [w314] -> w52
    tunnel: [w312] -> w50
    tunnel: w38 -> [w315]
    tunnel: w37 -> [w313]
    tunnel: w52 -> [w321]
    tunnel: [w322] -> w51
    tunnel: w50 -> [w318]
    tunnel: [w320] -> w49
    tunnel: [w331] -> w93
    tunnel: [w333] -> w91
    tunnel: w51 -> [w332]
    tunnel: w49 -> [w334]
    tunnel: w93 -> [w341]
    tunnel: [w340] -> w92
    tunnel: w91 -> [w338]
    tunnel: [w339] -> w90
    tunnel: [w351] -> w95
    tunnel: [w352] -> w94
    tunnel: w92 -> [w350]
    tunnel: w90 -> [w349]
    tunnel: w95 -> [w362]
    tunnel: w94 -> [w361]
    tunnel: [w364] -> w84
    tunnel: [w363] -> w83
    tunnel: [w358] -> w82
    tunnel: [w369] -> w96
    tunnel: [w370] -> w97
    tunnel: w84 -> [w370]
    tunnel: w83 -> [w369]
    tunnel: w82 -> [w365]
    frame #0 {
      w311 = refnum<visa-resource-name> "COM9" ("COM PORT")
      w309 = u16 0 items=["None", "XON/XOFF", "RTS/CTS", "XON/XOFF & RTS/CTS", "DTR/DSR", "XON/XOFF & DTR/DSR"] ("flow control (0:none)")
      w308 = u16 10 items=["1.0"=10, "1.5"=15, "2.0"=20] ("stop bits (10: 1 bit)")
      # "Stop bits"
      n110 = call-poly "VISA Configure Serial Port"("VISA resource name"=w311, "timeout (10sec)"=u32 10000, "baud rate (9600)"=u32 9600, "data bits (8)"=u16 8, "parity (0:none)"=enum16{"None", "Odd", "Even", "Mark", "Space"}."None", "stop bits (10: 1 bit)"=w308, "flow control (0:none)"=w309) -> ("VISA resource name out"=w304:refnum<visa-resource-name>, "error out"=w303:errorcluster)  [unwired: 7 in]
      "Y COM PORT" <- w311
    }
    frame #1 {
      n111 = call "mDrive Send Command.vi"("error in (no error)"=w313, "Extra"="EM=2", "Command"=T1."Send String", "VISA resource name"=w315) -> ("error out"=w312:errorcluster, "VISA resource name out"=w314:refnum<visa-resource-name>)  [unwired: 3 in, 1 out]
    }
    frame #2 {
      n112 = Number To Decimal String(number=1000000) -> (decimal integer string=w323:string)  [unwired: 1 in]
      n113 = call "mDrive Send Command.vi"("error in (no error)"=w318, "Extra"=w323, "Command"=T1."Accel Rate", "VISA resource name"=w321) -> ("error out"=w319:errorcluster, "VISA resource name out"=w327:refnum<visa-resource-name>)  [unwired: 3 in, 1 out]
      n114 = call "mDrive Send Command.vi"("error in (no error)"=w319, "Extra"=w323, "Command"=T1."Decel Rate", "VISA resource name"=w327) -> ("error out"=w320:errorcluster, "VISA resource name out"=w322:refnum<visa-resource-name>)  [unwired: 3 in, 1 out]
    }
    frame #3 {
      # "Run Current %"
      n115 = property on="Y Run Current %" class="DigNum (strict)"() -> ("Value"=w329:i32)  [unwired: 2 in, 2 out]
      n116 = Number To Decimal String(number=w329) -> (decimal integer string=w330:string)  [unwired: 1 in]
      n117 = call "mDrive Send Command.vi"("error in (no error)"=w334, "Extra"=w330, "Command"=T1."Run Current", "VISA resource name"=w332) -> ("error out"=w333:errorcluster, "VISA resource name out"=w331:refnum<visa-resource-name>)  [unwired: 3 in, 1 out]
    }
    frame #4 {
      # "Holding Current %"
      n118 = property on="Y Holding Current %" class="DigNum (strict)"() -> ("Value"=w336:i32)  [unwired: 2 in, 2 out]
      n119 = Number To Decimal String(number=w336) -> (decimal integer string=w337:string)  [unwired: 1 in]
      n120 = call "mDrive Send Command.vi"("error in (no error)"=w338, "Extra"=w337, "Command"=T1."Holding Current", "VISA resource name"=w341) -> ("error out"=w339:errorcluster, "VISA resource name out"=w340:refnum<visa-resource-name>)  [unwired: 3 in, 1 out]
    }
    frame #5 {
      # "Velocity Max"
      n121 = property on="Y Velocity SP step/sec" class="DigNum (strict)"() -> ("Value"=w348:i32)  [unwired: 2 in, 2 out]
      n122 = Number To Decimal String(number=w348) -> (decimal integer string=w347:string)  [unwired: 1 in]
      n123 = call "mDrive Send Command.vi"("error in (no error)"=w349, "Extra"=w347, "Command"=T1."Max Velocity", "VISA resource name"=w350) -> ("error out"=w345:errorcluster, "VISA resource name out"=w355:refnum<visa-resource-name>)  [unwired: 3 in, 1 out]
      n124 = call "mDrive Send Command.vi"("error in (no error)"=w345, "Extra"="VM", "Command"=T1."Print Parameter", "VISA resource name"=w355) -> ("error out"=w352:errorcluster, "read buffer"=w353:string, "VISA resource name out"=w351:refnum<visa-resource-name>)  [unwired: 3 in]
      n125 = Decimal String To Number(string=w353, offset=0) -> (number=w346:i32)  [unwired: 1 in, 1 out]
      n126 = property on="Y scan velocity MV step/sec" class="DigNum (strict)"("Val(Sgnl)"=w346) -> ()  [unwired: 2 in, 2 out]
    }
    frame #6 {
      # "PRINT POSITION"
      n127 = call "mDrive Send Command.vi"("error in (no error)"=w361, "Extra"="P", "Command"=T1."Print Parameter", "VISA resource name"=w362) -> ("error out"=w363:errorcluster, "read buffer"=w360:string, "VISA resource name out"=w364:refnum<visa-resource-name>)  [unwired: 3 in]
      n128 = Decimal String To Number(string=w360, offset=0) -> (number=w358:i32)  [unwired: 1 in, 1 out]
    }
    frame #7 {
      w367 = -2304000 ("lower limit")
      w368 = 2304000 ("upper limit")
      n129 = property on="Y Step SP" class="DigNum (strict)"("Val(Sgnl)"=w365) -> ()  [unwired: 2 in, 2 out]
      n130 = property on="Y Step SP" class="DigNum (strict)"("Maximum"=w368) -> ()  [unwired: 2 in, 2 out]
      n131 = property on="Y Step SP" class="DigNum (strict)"("Minimum"=w367) -> ()  [unwired: 2 in, 2 out]
      n132 = In Range and Coerce(upper limit=w368, x=w365, lower limit=w367) -> (In Range?=w366:bool)  [unwired: 1 out]
      n133 = property on="Y in Range" class="Bool (strict)"("Val(Sgnl)"=w366) -> ()  [unwired: 2 in, 2 out]
      "Y MINPOS" <- w367
      "Y MAXPOS" <- w368
    }
  }
  n134 = property on="Z Step SP" class="DigNum (strict)"("Minimum"=0 ("lower limit")) -> ()  [unwired: 2 in, 2 out]
  n135 = property on="R Step SP" class="DigNum (strict)"("Maximum"=0 ("upper limit")) -> ()  [unwired: 2 in, 2 out]
  n136 = flat-sequence {
    tunnel: [w372] -> w5
    tunnel: [w371] -> w4
    tunnel: w5 -> [w387]
    tunnel: w4 -> [w386]
    tunnel: [w385] -> w3
    tunnel: [w384] -> w2
    tunnel: [w390] -> w89
    tunnel: w3 -> [w398]
    tunnel: w2 -> [w397]
    tunnel: [w391] -> w1
    tunnel: w89 -> [w412]
    tunnel: [w411] -> w81
    tunnel: [w409] -> w80
    tunnel: [w414] -> w79
    tunnel: w1 -> [w413]
    tunnel: [w423] -> w87
    tunnel: [w424] -> w88
    tunnel: w81 -> [w424]
    tunnel: w80 -> [w423]
    tunnel: w79 -> [w419]
    frame #0 {
      w379 = refnum<visa-resource-name> "COM8" ("COM PORT")
      w377 = u16 0 items=["None", "XON/XOFF", "RTS/CTS", "XON/XOFF & RTS/CTS", "DTR/DSR", "XON/XOFF & DTR/DSR"] ("flow control (0:none)")
      w376 = u16 10 items=["1.0"=10, "1.5"=15, "2.0"=20] ("stop bits (10: 1 bit)")
      # "Stop bits"
      n137 = call-poly "VISA Configure Serial Port"("VISA resource name"=w379, "timeout (10sec)"=u32 10000, "baud rate (9600)"=u32 9600, "data bits (8)"=u16 8, "parity (0:none)"=enum16{"None", "Odd", "Even", "Mark", "Space"}."None", "stop bits (10: 1 bit)"=w376, "flow control (0:none)"=w377) -> ("VISA resource name out"=w372:refnum<visa-resource-name>, "error out"=w371:errorcluster)  [unwired: 7 in]
      "X COM PORT" <- w379
    }
    frame #1 {
      n138 = property on="X Run Current" class="DigNum (strict)"() -> ("Value"=w380:i32)  [unwired: 2 in, 2 out]
      n139 = Divide(x=w380, y=3.5) -> (x/y=w382:dbl)
      n140 = Number To Fractional String(number=w382) -> (F-format string=w383:string)  [unwired: 3 in]
      n141 = call "Applied Send Command.vi"("error in (no error)"=w386, "Extra"=w383, "Command"=T3."Change Current", "VISA resource name"=w387) -> ("error out"=w385:errorcluster, "VISA resource name out"=w384:refnum<visa-resource-name>)  [unwired: 3 in, 1 out]
    }
    frame #2 {
      # "VELOCITY"
      n142 = property on="X Velocity SP step/sec" class="DigNum (strict)"() -> ("Value"=w394:i32)  [unwired: 2 in, 2 out]
      n143 = property on="X steps/rev" class="DigNum (strict)"() -> ("Value"=w393:u32)  [unwired: 2 in, 2 out]
      n144 = Divide(x=w394, y=w393) -> (x/y=w392:dbl)
      n145 = Number To Fractional String(number=w392) -> (F-format string=w399:string)  [unwired: 3 in]
      n146 = call "Applied Send Command.vi"("error in (no error)"=w398, "Extra"=w399, "Command"=T3."Velocity Setting", "VISA resource name"=w397) -> ("error out"=w400:errorcluster, "VISA resource name out"=w407:refnum<visa-resource-name>)  [unwired: 3 in, 1 out]
      n147 = call "Time Delay30"("error in (no error)"=w400, "Delay Time (s)"=0.5) -> ("error out"=w405:errorcluster)  [unwired: 9 in]
      n148 = call "Applied Send Command.vi"("error in (no error)"=w405, "Extra"="", "Command"=T3."Velocity Setting", "VISA resource name"=w407) -> ("error out"=w390:errorcluster, "read buffer"=w403:string, "VISA resource name out"=w391:refnum<visa-resource-name>)  [unwired: 3 in]
      n149 = Fract/Exp String To Number(string=w403, offset=3) -> (number=w396:dbl)  [unwired: 2 in, 1 out]
      n150 = Multiply(x=w396, y=w393) -> (x*y=w395:dbl)
      n151 = property on="X velocity PV step/sec" class="DigNum (strict)"("Val(Sgnl)"=w395) -> ()  [unwired: 2 in, 2 out]
    }
    frame #3 {
      # "GET CURRENT POSITION"
      n152 = call "Applied Send Command.vi"("error in (no error)"=w412, "Extra"="", "Command"=T3."Immediate Position?", "VISA resource name"=w413) -> ("error out"=w410:errorcluster, "read buffer"=w416:string, "VISA resource name out"=w411:refnum<visa-resource-name>)  [unwired: 3 in]
      n153 = call "Time Delay13"("error in (no error)"=w410, "Delay Time (s)"=0.2) -> ("error out"=w409:errorcluster)  [unwired: 9 in]
      n154 = Hexadecimal String To Number(string=w416, offset=3) -> (number=w414:u32)  [unwired: 1 in, 1 out]
    }
    frame #4 {
      w421 = -500000 ("lower limit")
      w422 = 500000 ("upper limit")
      n155 = property on="X Step SP" class="DigNum (strict)"("Val(Sgnl)"=w419) -> ()  [unwired: 2 in, 2 out]
      n156 = property on="X Step SP" class="DigNum (strict)"("Maximum"=w422) -> ()  [unwired: 2 in, 2 out]
      n157 = In Range and Coerce(upper limit=w422, x=w419, lower limit=w421) -> (In Range?=w420:bool)  [unwired: 1 out]
      n158 = property on="X Step SP" class="DigNum (strict)"("Minimum"=w421) -> ()  [unwired: 2 in, 2 out]
      n159 = property on="X  in Range" class="Bool (strict)"("Val(Sgnl)"=w420) -> ()  [unwired: 2 in, 2 out]
      "X MINPOS" <- w421
      "X MAXPOS" <- w422
    }
  }
  n160 = property on="R Step SP" class="DigNum (strict)"("Minimum"=-6144000 ("lower limit")) -> ()  [unwired: 2 in, 2 out]
  n161 = property on="Z Step SP" class="DigNum (strict)"("Maximum"=102400000 ("upper limit")) -> ()  [unwired: 2 in, 2 out]
  n162 = call-poly <vilib>:"Read From Spreadsheet File.vi"("file path (dialog if empty)"=path "S:/LV codes/SCL2/POS.TXT") -> ("first row"=w24:i64[])  [unwired: 6 in, 4 out]
  n163 = call-poly <vilib>:"Read From Spreadsheet File.vi"("file path (dialog if empty)"=path "S:/LV codes/SCL2/PRESET.TXT") -> ("all rows"=w12:string[][])  [unwired: 6 in, 4 out]
  n164 = Array To Cluster(array=w24) -> (cluster=w23:T4)
  n165 = Transpose 2D Array(2D array=w12) -> (transposed array=w13:string[][])
  n166 = Unbundle(w23) -> ("first row[0]"=w21:i64, "first row[1]"=w20:i64, "first row[2]"=w19:i64, "first row[3]"=w18:i64)  [unwired: 5 out]
  n167 = Delete From Array(array=w13, index (row)=0) -> (deleted portion=w14:string[], array with subset deleted=w16:string[][])  [unwired: 2 in]
  n168 = property on="Reset X Motor Steps" class="DigNum (strict)"("Val(Sgnl)"=w21) -> ()  [unwired: 2 in, 2 out]
  n169 = property on="Reset Y Motor Steps" class="DigNum (strict)"("Val(Sgnl)"=w20) -> ()  [unwired: 2 in, 2 out]
  n170 = property on="Reset Z Motor Steps" class="DigNum (strict)"("Val(Sgnl)"=w19) -> ()  [unwired: 2 in, 2 out]
  n171 = property on="Reset R Motor Steps" class="DigNum (strict)"("Val(Sgnl)"=w18) -> ()  [unwired: 2 in, 2 out]
  n172 = Transpose 2D Array(2D array=w16) -> (transposed array=w17:string[][])
  n173 = property on="Preset positions" class="Ring (strict)"("Strings []"=w14) -> ()  [unwired: 2 in, 2 out]
  n174 = Decimal String To Number(string=w17) -> (number=w15:i32[][])  [unwired: 2 in, 1 out]
  n175 = Initialize Array(w6, w6, 4 ("dimension size")) -> (w9:i32[][])
  n176 = Build Array (concatenate)(w9, w15) -> (→"Presets":i32[][])
  n177 = while {
    tunnel: w97 -> [w443]
    tunnel: w96 -> [w446]
    tunnel: [w447] -> w31
    tunnel: [w445] -> w32
    tunnel: w88 -> [w442]
    tunnel: w87 -> [w441]
    tunnel: [w440] -> w86
    tunnel: [w439] -> w85
    tunnel: w60 -> [w438]
    tunnel: w59 -> [w437]
    tunnel: [w436] -> w34
    tunnel: [w435] -> w33
    tunnel: w58 -> [w434]
    tunnel: w57 -> [w433]
    tunnel: [w432] -> w30
    tunnel: [w431] -> w29
    stop <- "stop" stop-if-true
    n178 = property on="Preset positions" class="Ring (strict)"() -> ("Strings []"=w427:string[])  [unwired: 2 in, 2 out]
    n179 = event shown="[0] Timeout" {
      selector: _ -> [_ _ _ _ _ _ _ _ _ _ _ _ _ _ _ _ _ _ _ _ _ _ _ _ _]
      dyn-events: _ -> [_ _ _ _ _ _ _ _ _ _ _ _ _ _ _ _ _ _ _ _ _ _ _ _ _]
      timeout: 200 -> [_ _ _ _ _ _ _ _ _ _ _ _ _ _ _ _ _ _ _ _ _ _ _ _ _]
      tunnel: w446 -> [w548 _ _ _ _ _ _ _ _ _ _ _ w1360 _ _ _ _ w1622 _ _ w1717 w1733 w1777 w1854 w2096]
      tunnel: [w547 _ _ _ _ _ _ _ _ _ _ _ w1366 _ _ _ _ w1620 _ _ w1717 w1731 w1779 w1843 w2094] -> w447
      tunnel: w443 -> [w486 _ _ _ _ _ _ _ _ _ _ _ w1361 _ _ _ _ w1621 _ _ w1718 w1734 w1778 w1856 w2097]
      tunnel: [w546 _ _ _ _ _ _ _ _ _ _ _ w1367 _ _ _ _ w1617 _ _ w1718 w1732 w1780 w1844 w2095] -> w445
      tunnel: w442 -> [w485 _ _ _ _ _ _ _ _ _ _ _ _ _ _ w1524 w1584 _ _ _ _ w1728 w1770 w1860 w2093]
      tunnel: w441 -> [w523 _ _ _ _ _ _ _ _ _ _ _ _ _ _ w1523 w1583 _ _ _ _ w1727 w1769 w1858 w2092]
      tunnel: [w522 _ _ _ _ _ _ _ _ _ _ _ _ _ _ w1522 w1582 _ _ _ _ w1730 w1768 w1836 w2091] -> w440
      tunnel: [w521 _ _ _ _ _ _ _ _ _ _ _ _ _ _ w1521 w1581 _ _ _ _ w1729 w1767 w1834 w2090] -> w439
      tunnel: w438 -> [w495 _ _ _ _ _ _ _ _ _ _ _ _ w1412 _ _ _ _ w1652 _ _ w1726 w1764 w1852 w2089]
      tunnel: w437 -> [w498 _ _ _ _ _ _ _ _ _ _ _ _ w1411 _ _ _ _ w1651 _ _ w1725 w1763 w1850 w2088]
      tunnel: [w497 _ _ _ _ _ _ _ _ _ _ _ _ w1409 _ _ _ _ w1649 _ _ w1724 w1762 w1842 w2085] -> w436
      tunnel: [w496 _ _ _ _ _ _ _ _ _ _ _ _ w1410 _ _ _ _ w1650 _ _ w1723 w1761 w1841 w2084] -> w435
      tunnel: w434 -> [w494 _ _ _ _ _ _ _ _ _ _ _ _ _ w1465 _ _ _ _ w1686 _ w1722 w1758 w1847 w2087]
      tunnel: w433 -> [w493 _ _ _ _ _ _ _ _ _ _ _ _ _ w1464 _ _ _ _ w1685 _ w1721 w1757 w1845 w2086]
      tunnel: [w492 _ _ _ _ _ _ _ _ _ _ _ _ _ w1462 _ _ _ _ w1684 _ w1720 w1756 w1839 w2083] -> w432
      tunnel: [w491 _ _ _ _ _ _ _ _ _ _ _ _ _ w1463 _ _ _ _ w1683 _ w1719 w1755 w1838 w2082] -> w431
      event #0 {
        n180 = event-data() -> ()  [unwired: 1 in, 2 out]
        n181 = flat-sequence {
          tunnel: [w815] -> w534
          tunnel: [w826] -> w533
          tunnel: [w837] -> w532
          tunnel: [w811] -> w531
          tunnel: w485 -> [w822]
          tunnel: w523 -> [w810]
          tunnel: w534 -> [w848]
          tunnel: [w848] -> w530
          tunnel: w533 -> [w847]
          tunnel: [w847] -> w529
          tunnel: w532 -> [w846]
          tunnel: [w846] -> w528
          tunnel: w531 -> [w843]
          tunnel: [w843] -> w527
          tunnel: w530 -> [w857]
          tunnel: [w854] -> w526
          tunnel: w529 -> [w856]
          tunnel: [w855] -> w525
          tunnel: w528 -> [w853]
          tunnel: [w858] -> w524
          tunnel: w527 -> [w858]
          tunnel: w526 -> [w869]
          tunnel: w525 -> [w870]
          tunnel: w524 -> [w871]
          tunnel: [w868] -> w521
          tunnel: [w867] -> w522
          frame #0 {
            w825 = 0.2 ("Delay Time (s)")
            n182 = property on="X Step SP" class="DigNum (strict)"() -> ("Maximum"=w839:dbl)  [unwired: 2 in, 2 out]
            n183 = property on="X Step SP" class="DigNum (strict)"() -> ("Minimum"=w841:dbl)  [unwired: 2 in, 2 out]
            n184 = property on="X steps/rev" class="DigNum (strict)"() -> ("Value"=w835:u32)  [unwired: 2 in, 2 out]
            n185 = property on="X offset mm" class="DigNum (strict)"() -> ("Value"=w831:dbl)  [unwired: 2 in, 2 out]
            n186 = To Long Integer(number=w839) -> (32bit integer=w838:i32)
            n187 = To Long Integer(number=w841) -> (32bit integer=w840:i32)
            n188 = To Double Precision Float(number=w835) -> (double precision float=w836:dbl)
            n189 = call "Applied Send Command.vi"("error in (no error)"=w810, "Command"=T3."Immediate Position?", "VISA resource name"=w822) -> ("error out"=w820:errorcluster, "read buffer"=w821:string, "VISA resource name out"=w816:refnum<visa-resource-name>)  [unwired: 4 in]
            n190 = call "Time Delay12"("error in (no error)"=w820, "Delay Time (s)"=w825) -> ("error out"=w813:errorcluster)  [unwired: 9 in]
            n191 = Hexadecimal String To Number(string=w821, offset=3) -> (number=w827:u32)  [unwired: 1 in, 1 out]
            n192 = To Long Integer(number=w827) -> (32bit integer=w829:i32)
            n193 = call "Applied Send Command.vi"("error in (no error)"=w813, "Command"=T3."Request Status", "VISA resource name"=w816) -> ("error out"=w814:errorcluster, "read buffer"=w818:string, "VISA resource name out"=w815:refnum<visa-resource-name>)  [unwired: 4 in]
            n194 = property on="X Step PV" class="DigNum (strict)"("Val(Sgnl)"=w829) -> ()  [unwired: 2 in, 2 out]
            n195 = String Subset(string=w818, offset (0)=0, length (rest)=1 ("length (rest)")) -> (substring=w807:string)
            n196 = call "Time Delay11"("error in (no error)"=w814, "Delay Time (s)"=w825) -> ("error out"=w826:errorcluster)  [unwired: 9 in]
            n197 = In Range and Coerce(upper limit=w838, x=w829, lower limit=w840) -> (In Range?=w837:bool)  [unwired: 1 out]
            n198 = To Double Precision Float(number=w829) -> (double precision float=w830:dbl)
            n199 = Not Equal?(x=w807, y="R") -> (x != y?=w811:bool)
            n200 = Equal?(x=w807, y="R") -> (x = y?=w824:bool)
            n201 = property on="X  in Range" class="Bool (strict)"("Val(Sgnl)"=w837) -> ()  [unwired: 2 in, 2 out]
            n202 = property on="X Ready" class="Bool (strict)"("Val(Sgnl)"=w824) -> ()  [unwired: 2 in, 2 out]
            n203 = Divide(x=w830, y=w836) -> (x/y=w834:dbl)
            n204 = property on="X mm/rev" class="DigNum (strict)"() -> ("Value"=w833:dbl)  [unwired: 2 in, 2 out]
            n205 = Multiply(x=w834, y=w833) -> (x*y=w832:dbl)
            n206 = property on="X  in Motion" class="Bool (strict)"("Val(Sgnl)"=w811) -> ()  [unwired: 2 in, 2 out]
            n207 = Add(x=w832, y=w831) -> (x+y=w828:dbl)
            n208 = property on="X Position mm PV" class="DigNum (strict)"("Val(Sgnl)"=w828) -> ()  [unwired: 2 in, 2 out]
          }
          frame #1 {
            n209 = property on="X Scan" class="Bool (strict)"() -> ("Value"=w844:bool)  [unwired: 2 in, 2 out]
            n210 = Or(x=w843, y=w844) -> (x .or. y?=w845:bool)
            n211 = case shown="True" w845 {
              frame #0 {
                n212 = property on="X Go" class="Bool"("DisabledEnum"=T2."Enabled" ("Disabled")) -> ()  [unwired: 2 in, 2 out]
                n213 = property on="X Scan OK" class="Bool"("DisabledEnum"=T2."Enabled" ("Disabled")) -> ()  [unwired: 2 in, 2 out]
              }
              frame #1 {
                n214 = property on="X Go" class="Bool"("DisabledEnum"=T2."Disabled and Grayed Out" ("Disabled")) -> ()  [unwired: 2 in, 2 out]
                n215 = property on="X Scan OK" class="Bool"("DisabledEnum"=T2."Disabled and Grayed Out" ("Disabled")) -> ()  [unwired: 2 in, 2 out]
              }
            }
          }
          frame #2 {
            n216 = case shown="False" w853 {
              tunnel: w857 -> [w860 w865]
              tunnel: [w862 w865] -> w854
              tunnel: [w863 w864] -> w855
              tunnel: w856 -> [w859 w864]
              frame #0 {
                n217 = call "Applied Send Command.vi"("error in (no error)"=w859, "Command"=T3."Stop & Kill Buffer", "VISA resource name"=w860) -> ("error out"=w863:errorcluster, "VISA resource name out"=w862:refnum<visa-resource-name>)  [unwired: 4 in, 1 out]
              }
              frame #1 {
              }
            }
          }
          frame #3 {
            n218 = property on="X Backlash corr" class="Bool (strict)"() -> ("Value"=w872:bool)  [unwired: 2 in, 2 out]
            n219 = Implies(1:w871, 2:w872) -> (0:w866:bool)
            n220 = case shown="False" w866 {
              tunnel: w870 -> [w886 w905]
              tunnel: w869 -> [w887 w906]
              tunnel: [w889 w905] -> w868
              tunnel: [w888 w906] -> w867
              frame #0 {
                w877 = 0.1 ("Delay Time (s)")
                # "Backlash"
                n221 = property on="X steps/rev" class="DigNum (strict)"() -> ("Value"=w875:u32)  [unwired: 2 in, 2 out]
                n222 = property on="X Backlash steps/sec" class="DigNum (strict)"() -> ("Value"=w876:i32)  [unwired: 2 in, 2 out]
                n223 = Divide(x=w876, y=w875) -> (x/y=w874:dbl)
                n224 = Number To Fractional String(number=w874) -> (F-format string=w873:string)  [unwired: 3 in]
                n225 = property on="X Backlash" class="DigNum (strict)"() -> ("Value"=w892:i32)  [unwired: 2 in, 2 out]
                n226 = call "Applied Send Command.vi"("error in (no error)"=w886, "Extra"=w873, "Command"=T3."Velocity Setting", "VISA resource name"=w887) -> ("error out"=w879:errorcluster, "VISA resource name out"=w890:refnum<visa-resource-name>)  [unwired: 3 in, 1 out]
                n227 = call "Time Delay35"("error in (no error)"=w879, "Delay Time (s)"=w877) -> ("error out"=w878:errorcluster)  [unwired: 9 in]
                n228 = Number To Decimal String(number=w892) -> (decimal integer string=w896:string)  [unwired: 1 in]
                n229 = To Long Integer(number=w892) -> (32bit integer=w901:i32)
                n230 = Negate(x=w901) -> (-x=w902:i32)
                n231 = call "Applied Send Command.vi"("error in (no error)"=w878, "Extra"=w896, "Command"=T3."Distance or Position", "VISA resource name"=w890) -> ("error out"=w885:errorcluster, "VISA resource name out"=w897:refnum<visa-resource-name>)  [unwired: 3 in, 1 out]
                n232 = Number To Decimal String(number=w902) -> (decimal integer string=w895:string)  [unwired: 1 in]
                n233 = call "Time Delay32"("error in (no error)"=w885, "Delay Time (s)"=w877) -> ("error out"=w884:errorcluster)  [unwired: 9 in]
                n234 = call "Applied Send Command.vi"("error in (no error)"=w884, "Command"=T3."Feed to Length", "VISA resource name"=w897) -> ("error out"=w883:errorcluster, "VISA resource name out"=w894:refnum<visa-resource-name>)  [unwired: 4 in, 1 out]
                n235 = call "Time Delay33"("error in (no error)"=w883, "Delay Time (s)"=w877) -> ("error out"=w882:errorcluster)  [unwired: 9 in]
                n236 = call "Applied Send Command.vi"("error in (no error)"=w882, "Extra"=w895, "Command"=T3."Distance or Position", "VISA resource name"=w894) -> ("error out"=w881:errorcluster, "VISA resource name out"=w893:refnum<visa-resource-name>)  [unwired: 3 in, 1 out]
                n237 = call "Time Delay34"("error in (no error)"=w881, "Delay Time (s)"=w877) -> ("error out"=w880:errorcluster)  [unwired: 9 in]
                n238 = call "Applied Send Command.vi"("error in (no error)"=w880, "Command"=T3."Feed to Length", "VISA resource name"=w893) -> ("error out"=w889:errorcluster, "VISA resource name out"=w888:refnum<visa-resource-name>)  [unwired: 4 in, 1 out]
                n239 = property on="X Backlash corr" class="Bool (strict)"("Val(Sgnl)"=FALSE ("Value (Signaling)")) -> ()  [unwired: 2 in, 2 out]
              }
              frame #1 {
              }
            }
          }
        }
        n240 = flat-sequence {
          tunnel: w548 -> [w939]
          tunnel: w486 -> [w938]
          tunnel: [w944] -> w545
          tunnel: [w919] -> w543
          tunnel: [w931] -> w541
          tunnel: [w910] -> w539
          tunnel: w545 -> [w950]
          tunnel: [w950] -> w544
          tunnel: w543 -> [w949]
          tunnel: [w949] -> w542
          tunnel: w541 -> [w948]
          tunnel: [w948] -> w540
          tunnel: w539 -> [w945]
          tunnel: [w945] -> w535
          tunnel: w544 -> [w957]
          tunnel: [w958] -> w538
          tunnel: w542 -> [w960]
          tunnel: [w959] -> w537
          tunnel: w540 -> [w956]
          tunnel: [w955] -> w536
          tunnel: w535 -> [w955]
          tunnel: w538 -> [w970]
          tunnel: w537 -> [w971]
          tunnel: w536 -> [w973]
          tunnel: [w969] -> w547
          tunnel: [w968] -> w546
          frame #0 {
            w914 = 0.05 ("Delay Time (s)")
            n241 = property on="Y Step SP" class="DigNum (strict)"() -> ("Maximum"=w933:dbl)  [unwired: 2 in, 2 out]
            n242 = property on="Y Step SP" class="DigNum (strict)"() -> ("Minimum"=w935:dbl)  [unwired: 2 in, 2 out]
            n243 = property on="Y steps/rev" class="DigNum (strict)"() -> ("Value"=w929:u32)  [unwired: 2 in, 2 out]
            n244 = property on="Y offset mm" class="DigNum (strict)"() -> ("Value"=w925:dbl)  [unwired: 2 in, 2 out]
            n245 = To Long Integer(number=w933) -> (32bit integer=w932:i32)
            n246 = To Long Integer(number=w935) -> (32bit integer=w934:i32)
            n247 = To Double Precision Float(number=w929) -> (double precision float=w930:dbl)
            n248 = call "mDrive Send Command.vi"("error in (no error)"=w939, "Extra"="P", "Command"=T1."Print Parameter", "VISA resource name"=w938) -> ("error out"=w937:errorcluster, "read buffer"=w943:string, "VISA resource name out"=w941:refnum<visa-resource-name>)  [unwired: 3 in]
            n249 = call "Time Delay4"("error in (no error)"=w937, "Delay Time (s)"=w914) -> ("error out"=w936:errorcluster)  [unwired: 9 in]
            n250 = Decimal String To Number(string=w943, offset=0) -> (number=w921:i32)  [unwired: 1 in, 1 out]
            n251 = To Long Integer(number=w921) -> (32bit integer=w923:i32)
            n252 = property on="Y Step PV" class="DigNum (strict)"("Val(Sgnl)"=w923) -> ()  [unwired: 2 in, 2 out]
            n253 = call "mDrive Send Command.vi"("error in (no error)"=w936, "Extra"="MV", "Command"=T1."Print Parameter", "VISA resource name"=w941) -> ("error out"=w940:errorcluster, "read buffer"=w907:string, "VISA resource name out"=w944:refnum<visa-resource-name>)  [unwired: 3 in]
            n254 = call "Time Delay3"("error in (no error)"=w940, "Delay Time (s)"=w914) -> ("error out"=w919:errorcluster)  [unwired: 9 in]
            n255 = In Range and Coerce(upper limit=w932, x=w923, lower limit=w934) -> (In Range?=w931:bool)  [unwired: 1 out]
            n256 = To Double Precision Float(number=w923) -> (double precision float=w924:dbl)
            n257 = Decimal String To Number(string=w907, offset=0 ("offset (0)")) -> (number=w913:i32)  [unwired: 1 in, 1 out]
            n258 = Not Equal?(x=w907, y="") -> (x != y?=w908:bool)
            n259 = property on="Y in Range" class="Bool (strict)"("Val(Sgnl)"=w931) -> ()  [unwired: 2 in, 2 out]
            n260 = property on="Y Ready" class="Bool (strict)"("Val(Sgnl)"=w908) -> ()  [unwired: 2 in, 2 out]
            n261 = Divide(x=w924, y=w930) -> (x/y=w928:dbl)
            n262 = Number To Boolean Array(number=w913) -> (Boolean array=w912:bool[])
            n263 = property on="Y mm/rev" class="DigNum (strict)"() -> ("Value"=w927:dbl)  [unwired: 2 in, 2 out]
            n264 = Index Array(array=w912, index=0) -> (element=w910:bool)
            n265 = Multiply(x=w928, y=w927) -> (x*y=w926:dbl)
            n266 = property on="Y in Motion" class="Bool (strict)"("Val(Sgnl)"=w910) -> ()  [unwired: 2 in, 2 out]
            n267 = Add(x=w926, y=w925) -> (x+y=w922:dbl)
            n268 = property on="Y Position mm PV" class="DigNum (strict)"("Val(Sgnl)"=w922) -> ()  [unwired: 2 in, 2 out]
          }
          frame #1 {
            n269 = property on="Y Scan" class="Bool (strict)"() -> ("Value"=w946:bool)  [unwired: 2 in, 2 out]
            n270 = Or(x=w945, y=w946) -> (x .or. y?=w947:bool)
            n271 = case shown="True" w947 {
              frame #0 {
                n272 = property on="Y Go" class="Bool"("DisabledEnum"=T2."Enabled" ("Disabled")) -> ()  [unwired: 2 in, 2 out]
                n273 = property on="Y Scan OK" class="Bool"("DisabledEnum"=T2."Enabled" ("Disabled")) -> ()  [unwired: 2 in, 2 out]
              }
              frame #1 {
                n274 = property on="Y Go" class="Bool"("DisabledEnum"=T2."Disabled and Grayed Out" ("Disabled")) -> ()  [unwired: 2 in, 2 out]
                n275 = property on="Y Scan OK" class="Bool"("DisabledEnum"=T2."Disabled and Grayed Out" ("Disabled")) -> ()  [unwired: 2 in, 2 out]
              }
            }
          }
          frame #2 {
            n276 = case shown="False" w956 {
              tunnel: w957 -> [w963 w967]
              tunnel: [w964 w967] -> w958
              tunnel: [w965 w966] -> w959
              tunnel: w960 -> [w962 w966]
              frame #0 {
                n277 = call "mDrive Send Command.vi"("error in (no error)"=w962, "Command"=T1."Stop", "VISA resource name"=w963) -> ("error out"=w965:errorcluster, "VISA resource name out"=w964:refnum<visa-resource-name>)  [unwired: 4 in, 1 out]
              }
              frame #1 {
              }
            }
          }
          frame #3 {
            n278 = property on="Y Backlash corr" class="Bool (strict)"() -> ("Value"=w974:bool)  [unwired: 2 in, 2 out]
            n279 = Implies(1:w973, 2:w974) -> (0:w972:bool)
            n280 = case shown="False" w972 {
              tunnel: w971 -> [w981 w1034]
              tunnel: w970 -> [w980 w1035]
              tunnel: [w979 w1034] -> w969
              tunnel: [w978 w1035] -> w968
              frame #0 {
                # "Backlash"
                n281 = flat-sequence {
                  tunnel: [w996] -> w993
                  tunnel: [w998] -> w992
                  tunnel: [w997] -> w991
                  tunnel: w981 -> [w995]
                  tunnel: w980 -> [w994]
                  tunnel: w993 -> [w1006]
                  tunnel: [w1006] -> w990
                  tunnel: w992 -> [w1005]
                  tunnel: w991 -> [w1004]
                  tunnel: [w1003] -> w989
                  tunnel: [w1002] -> w988
                  tunnel: [w1001] -> w977
                  tunnel: w990 -> [w1016]
                  tunnel: w989 -> [w1015]
                  tunnel: w988 -> [w1013]
                  tunnel: [w1014] -> w987
                  tunnel: [w1013] -> w986
                  tunnel: [w1012] -> w983
                  tunnel: [w1011] -> w982
                  tunnel: w977 -> [w1011]
                  tunnel: w987 -> [w1027]
                  tunnel: w986 -> [w1020]
                  tunnel: [w1027] -> w985
                  tunnel: [w1026] -> w984
                  tunnel: w983 -> [w1026]
                  tunnel: w982 -> [w1022]
                  tunnel: [w1021] -> w975
                  tunnel: w985 -> [w1031]
                  tunnel: w984 -> [w1030]
                  tunnel: [w1029] -> w979
                  tunnel: [w1028] -> w976
                  tunnel: w975 -> [w1028]
                  tunnel: [w1033] -> w978
                  tunnel: w976 -> [w1033]
                  frame #0 {
                    n282 = property on="Y Backlash steps/sec" class="DigNum (strict)"() -> ("Value"=w996:i32)  [unwired: 2 in, 2 out]
                    n283 = Number To Decimal String(number=w996) -> (decimal integer string=w999:string)  [unwired: 1 in]
                    n284 = call "mDrive Send Command.vi"("error in (no error)"=w995, "Extra"=w999, "Command"=T1."Max Velocity", "VISA resource name"=w994) -> ("error out"=w997:errorcluster, "VISA resource name out"=w998:refnum<visa-resource-name>)  [unwired: 3 in, 1 out]
                  }
                  frame #1 {
                    n285 = property on="Y Backlash" class="DigNum (strict)"() -> ("Value"=w1001:i32)  [unwired: 2 in, 2 out]
                    n286 = Number To Decimal String(number=w1001) -> (decimal integer string=w1007:string)  [unwired: 1 in]
                    n287 = call "mDrive Send Command.vi"("error in (no error)"=w1004, "Extra"=w1007, "Command"=T1."Move to Relative Position", "VISA resource name"=w1005) -> ("error out"=w1003:errorcluster, "VISA resource name out"=w1002:refnum<visa-resource-name>)  [unwired: 3 in, 1 out]
                  }
                  frame #2 {
                    n288 = To Double Precision Float(number=w1011) -> (double precision float=w1009:dbl)
                    n289 = To Double Precision Float(number=w1016) -> (double precision float=w1018:dbl)
                    n290 = Absolute Value(x=w1009) -> (abs(x)=w1010:dbl)
                    n291 = Divide(x=w1010, y=w1018) -> (x/y=w1019:dbl)
                    n292 = Add(x=w1019, y=0.3) -> (x+y=w1012:dbl)
                    n293 = call "Time Delay8"("error in (no error)"=w1015, "Delay Time (s)"=w1012) -> ("error out"=w1014:errorcluster)  [unwired: 9 in]
                  }
                  frame #3 {
                    n294 = Negate(x=w1022) -> (-x=w1023:i32)
                    n295 = Number To Decimal String(number=w1023) -> (decimal integer string=w1024:string)  [unwired: 1 in]
                    n296 = call "mDrive Send Command.vi"("Extra"=w1024, "Command"=T1."Move to Relative Position", "VISA resource name"=w1020) -> ("VISA resource name out"=w1021:refnum<visa-resource-name>)  [unwired: 4 in, 2 out]
                  }
                  frame #4 {
                    n297 = call "Time Delay2"("error in (no error)"=w1031, "Delay Time (s)"=w1030) -> ("error out"=w1029:errorcluster)  [unwired: 9 in]
                  }
                  frame #5 {
                    n298 = property on="Y Backlash corr" class="Bool (strict)"("Val(Sgnl)"=FALSE ("Value (Signaling)")) -> ()  [unwired: 2 in, 2 out]
                  }
                }
              }
              frame #1 {
              }
            }
          }
        }
        n299 = flat-sequence {
          tunnel: [w715] -> w520
          tunnel: [w692] -> w519
          tunnel: [w704] -> w518
          tunnel: [w683] -> w517
          tunnel: w495 -> [w682]
          tunnel: w498 -> [w681]
          tunnel: w520 -> [w721]
          tunnel: [w721] -> w516
          tunnel: w519 -> [w720]
          tunnel: [w720] -> w515
          tunnel: w518 -> [w719]
          tunnel: [w719] -> w514
          tunnel: w517 -> [w716]
          tunnel: [w716] -> w513
          tunnel: w516 -> [w728]
          tunnel: [w729] -> w512
          tunnel: w515 -> [w731]
          tunnel: [w730] -> w511
          tunnel: w514 -> [w727]
          tunnel: [w726] -> w510
          tunnel: w513 -> [w726]
          tunnel: w512 -> [w741]
          tunnel: w511 -> [w742]
          tunnel: w510 -> [w744]
          tunnel: [w740] -> w496
          tunnel: [w739] -> w497
          frame #0 {
            w687 = 0.05 ("Delay Time (s)")
            n300 = property on="Z Step SP" class="DigNum (strict)"() -> ("Maximum"=w706:dbl)  [unwired: 2 in, 2 out]
            n301 = property on="Z Step SP" class="DigNum (strict)"() -> ("Minimum"=w708:dbl)  [unwired: 2 in, 2 out]
            n302 = property on="Z steps/rev" class="DigNum (strict)"() -> ("Value"=w702:u32)  [unwired: 2 in, 2 out]
            n303 = property on="Z offset mm" class="DigNum (strict)"() -> ("Value"=w698:dbl)  [unwired: 2 in, 2 out]
            n304 = To Long Integer(number=w706) -> (32bit integer=w705:i32)
            n305 = To Long Integer(number=w708) -> (32bit integer=w707:i32)
            n306 = To Double Precision Float(number=w702) -> (double precision float=w703:dbl)
            n307 = call "mDrive Send Command.vi"("error in (no error)"=w681, "Extra"="P", "Command"=T1."Print Parameter", "VISA resource name"=w682) -> ("error out"=w710:errorcluster, "read buffer"=w714:string, "VISA resource name out"=w712:refnum<visa-resource-name>)  [unwired: 3 in]
            n308 = call "Time Delay17"("error in (no error)"=w710, "Delay Time (s)"=w687) -> ("error out"=w709:errorcluster)  [unwired: 9 in]
            n309 = Decimal String To Number(string=w714, offset=0) -> (number=w694:i32)  [unwired: 1 in, 1 out]
            n310 = To Long Integer(number=w694) -> (32bit integer=w696:i32)
            n311 = property on="Z Step PV" class="DigNum (strict)"("Val(Sgnl)"=w696) -> ()  [unwired: 2 in, 2 out]
            n312 = call "mDrive Send Command.vi"("error in (no error)"=w709, "Extra"="MV", "Command"=T1."Print Parameter", "VISA resource name"=w712) -> ("error out"=w711:errorcluster, "read buffer"=w678:string, "VISA resource name out"=w715:refnum<visa-resource-name>)  [unwired: 3 in]
            n313 = call "Time Delay16"("error in (no error)"=w711, "Delay Time (s)"=w687) -> ("error out"=w692:errorcluster)  [unwired: 9 in]
            n314 = In Range and Coerce(upper limit=w705, x=w696, lower limit=w707) -> (In Range?=w704:bool)  [unwired: 1 out]
            n315 = To Double Precision Float(number=w696) -> (double precision float=w697:dbl)
            n316 = Decimal String To Number(string=w678, offset=0 ("offset (0)")) -> (number=w686:i32)  [unwired: 1 in, 1 out]
            n317 = Not Equal?(x=w678, y="") -> (x != y?=w679:bool)
            n318 = property on="Z in Range" class="Bool (strict)"("Val(Sgnl)"=w704) -> ()  [unwired: 2 in, 2 out]
            n319 = property on="Z Ready" class="Bool (strict)"("Val(Sgnl)"=w679) -> ()  [unwired: 2 in, 2 out]
            n320 = Divide(x=w697, y=w703) -> (x/y=w701:dbl)
            n321 = Number To Boolean Array(number=w686) -> (Boolean array=w685:bool[])
            n322 = property on="Z mm/rev" class="DigNum (strict)"() -> ("Value"=w700:dbl)  [unwired: 2 in, 2 out]
            n323 = Index Array(array=w685, index=0) -> (element=w683:bool)
            n324 = Multiply(x=w701, y=w700) -> (x*y=w699:dbl)
            n325 = property on="Z in Motion" class="Bool (strict)"("Val(Sgnl)"=w683) -> ()  [unwired: 2 in, 2 out]
            n326 = Add(x=w699, y=w698) -> (x+y=w695:dbl)
            n327 = property on="Z Position mm PV" class="DigNum (strict)"("Val(Sgnl)"=w695) -> ()  [unwired: 2 in, 2 out]
          }
          frame #1 {
            n328 = property on="Z Scan" class="Bool (strict)"() -> ("Value"=w717:bool)  [unwired: 2 in, 2 out]
            n329 = Or(x=w716, y=w717) -> (x .or. y?=w718:bool)
            n330 = case shown="True" w718 {
              frame #0 {
                n331 = property on="Z Go" class="Bool"("DisabledEnum"=T2."Enabled" ("Disabled")) -> ()  [unwired: 2 in, 2 out]
                n332 = property on="Z Scan OK" class="Bool"("DisabledEnum"=T2."Enabled" ("Disabled")) -> ()  [unwired: 2 in, 2 out]
              }
              frame #1 {
                n333 = property on="Z Go" class="Bool"("DisabledEnum"=T2."Disabled and Grayed Out" ("Disabled")) -> ()  [unwired: 2 in, 2 out]
                n334 = property on="Z Scan OK" class="Bool"("DisabledEnum"=T2."Disabled and Grayed Out" ("Disabled")) -> ()  [unwired: 2 in, 2 out]
              }
            }
          }
          frame #2 {
            n335 = case shown="False" w727 {
              tunnel: w728 -> [w734 w738]
              tunnel: [w735 w738] -> w729
              tunnel: [w736 w737] -> w730
              tunnel: w731 -> [w733 w737]
              frame #0 {
                n336 = call "mDrive Send Command.vi"("error in (no error)"=w733, "Command"=T1."Stop", "VISA resource name"=w734) -> ("error out"=w736:errorcluster, "VISA resource name out"=w735:refnum<visa-resource-name>)  [unwired: 4 in, 1 out]
              }
              frame #1 {
              }
            }
          }
          frame #3 {
            n337 = property on="Z Backlash corr" class="Bool (strict)"() -> ("Value"=w745:bool)  [unwired: 2 in, 2 out]
            n338 = Implies(1:w744, 2:w745) -> (0:w743:bool)
            n339 = case shown="False" w743 {
              tunnel: w742 -> [w752 w805]
              tunnel: w741 -> [w751 w806]
              tunnel: [w750 w805] -> w740
              tunnel: [w749 w806] -> w739
              frame #0 {
                # "Backlash"
                n340 = flat-sequence {
                  tunnel: [w767] -> w764
                  tunnel: [w769] -> w763
                  tunnel: [w768] -> w762
                  tunnel: w752 -> [w766]
                  tunnel: w751 -> [w765]
                  tunnel: w764 -> [w777]
                  tunnel: [w777] -> w761
                  tunnel: w763 -> [w776]
                  tunnel: w762 -> [w775]
                  tunnel: [w774] -> w760
                  tunnel: [w773] -> w759
                  tunnel: [w772] -> w748
                  tunnel: w761 -> [w787]
                  tunnel: w760 -> [w786]
                  tunnel: w759 -> [w784]
                  tunnel: [w785] -> w758
                  tunnel: [w784] -> w757
                  tunnel: [w783] -> w754
                  tunnel: [w782] -> w753
                  tunnel: w748 -> [w782]
                  tunnel: w758 -> [w798]
                  tunnel: w757 -> [w791]
                  tunnel: [w798] -> w756
                  tunnel: [w797] -> w755
                  tunnel: w754 -> [w797]
                  tunnel: w753 -> [w793]
                  tunnel: [w792] -> w746
                  tunnel: w756 -> [w802]
                  tunnel: w755 -> [w801]
                  tunnel: [w800] -> w750
                  tunnel: [w799] -> w747
                  tunnel: w746 -> [w799]
                  tunnel: [w804] -> w749
                  tunnel: w747 -> [w804]
                  frame #0 {
                    n341 = property on="Z Backlash steps/sec" class="DigNum (strict)"() -> ("Value"=w767:i32)  [unwired: 2 in, 2 out]
                    n342 = Number To Decimal String(number=w767) -> (decimal integer string=w770:string)  [unwired: 1 in]
                    n343 = call "mDrive Send Command.vi"("error in (no error)"=w766, "Extra"=w770, "Command"=T1."Max Velocity", "VISA resource name"=w765) -> ("error out"=w768:errorcluster, "VISA resource name out"=w769:refnum<visa-resource-name>)  [unwired: 3 in, 1 out]
                  }
                  frame #1 {
                    n344 = property on="Z Backlash" class="DigNum (strict)"() -> ("Value"=w772:i32)  [unwired: 2 in, 2 out]
                    n345 = Number To Decimal String(number=w772) -> (decimal integer string=w778:string)  [unwired: 1 in]
                    n346 = call "mDrive Send Command.vi"("error in (no error)"=w775, "Extra"=w778, "Command"=T1."Move to Relative Position", "VISA resource name"=w776) -> ("error out"=w774:errorcluster, "VISA resource name out"=w773:refnum<visa-resource-name>)  [unwired: 3 in, 1 out]
                  }
                  frame #2 {
                    n347 = To Double Precision Float(number=w782) -> (double precision float=w780:dbl)
                    n348 = To Double Precision Float(number=w787) -> (double precision float=w789:dbl)
                    n349 = Absolute Value(x=w780) -> (abs(x)=w781:dbl)
                    n350 = Divide(x=w781, y=w789) -> (x/y=w790:dbl)
                    n351 = Add(x=w790, y=0.5) -> (x+y=w783:dbl)
                    n352 = call "Time Delay18"("error in (no error)"=w786, "Delay Time (s)"=w783) -> ("error out"=w785:errorcluster)  [unwired: 9 in]
                  }
                  frame #3 {
                    n353 = Negate(x=w793) -> (-x=w794:i32)
                    n354 = Number To Decimal String(number=w794) -> (decimal integer string=w795:string)  [unwired: 1 in]
                    n355 = call "mDrive Send Command.vi"("Extra"=w795, "Command"=T1."Move to Relative Position", "VISA resource name"=w791) -> ("VISA resource name out"=w792:refnum<visa-resource-name>)  [unwired: 4 in, 2 out]
                  }
                  frame #4 {
                    n356 = call "Time Delay19"("error in (no error)"=w802, "Delay Time (s)"=w801) -> ("error out"=w800:errorcluster)  [unwired: 9 in]
                  }
                  frame #5 {
                    n357 = property on="Z Backlash corr" class="Bool (strict)"("Val(Sgnl)"=FALSE ("Value (Signaling)")) -> ()  [unwired: 2 in, 2 out]
                  }
                }
              }
              frame #1 {
              }
            }
          }
        }
        n358 = flat-sequence {
          tunnel: [w586] -> w509
          tunnel: [w563] -> w508
          tunnel: [w575] -> w507
          tunnel: [w554] -> w506
          tunnel: w494 -> [w553]
          tunnel: w493 -> [w552]
          tunnel: w509 -> [w592]
          tunnel: [w592] -> w505
          tunnel: w508 -> [w591]
          tunnel: [w591] -> w504
          tunnel: w507 -> [w590]
          tunnel: [w590] -> w503
          tunnel: w506 -> [w587]
          tunnel: [w587] -> w502
          tunnel: w505 -> [w599]
          tunnel: [w600] -> w501
          tunnel: w504 -> [w602]
          tunnel: [w601] -> w500
          tunnel: w503 -> [w598]
          tunnel: [w597] -> w499
          tunnel: w502 -> [w597]
          tunnel: w501 -> [w612]
          tunnel: w500 -> [w613]
          tunnel: w499 -> [w615]
          tunnel: [w611] -> w491
          tunnel: [w610] -> w492
          frame #0 {
            w558 = 0.05 ("Delay Time (s)")
            n359 = property on="R Step SP" class="DigNum (strict)"() -> ("Maximum"=w577:dbl)  [unwired: 2 in, 2 out]
            n360 = property on="R Step SP" class="DigNum (strict)"() -> ("Minimum"=w579:dbl)  [unwired: 2 in, 2 out]
            n361 = property on="R steps/rev" class="DigNum (strict)"() -> ("Value"=w573:u32)  [unwired: 2 in, 2 out]
            n362 = property on="R offset deg" class="DigNum (strict)"() -> ("Value"=w569:dbl)  [unwired: 2 in, 2 out]
            n363 = To Long Integer(number=w577) -> (32bit integer=w576:i32)
            n364 = To Long Integer(number=w579) -> (32bit integer=w578:i32)
            n365 = To Double Precision Float(number=w573) -> (double precision float=w574:dbl)
            n366 = call "mDrive Send Command.vi"("error in (no error)"=w552, "Extra"="P", "Command"=T1."Print Parameter", "VISA resource name"=w553) -> ("error out"=w581:errorcluster, "read buffer"=w585:string, "VISA resource name out"=w583:refnum<visa-resource-name>)  [unwired: 3 in]
            n367 = call "Time Delay21"("error in (no error)"=w581, "Delay Time (s)"=w558) -> ("error out"=w580:errorcluster)  [unwired: 9 in]
            n368 = Decimal String To Number(string=w585, offset=0) -> (number=w565:i32)  [unwired: 1 in, 1 out]
            n369 = To Long Integer(number=w565) -> (32bit integer=w567:i32)
            n370 = property on="R Step PV" class="DigNum (strict)"("Val(Sgnl)"=w567) -> ()  [unwired: 2 in, 2 out]
            n371 = call "mDrive Send Command.vi"("error in (no error)"=w580, "Extra"="MV", "Command"=T1."Print Parameter", "VISA resource name"=w583) -> ("error out"=w582:errorcluster, "read buffer"=w549:string, "VISA resource name out"=w586:refnum<visa-resource-name>)  [unwired: 3 in]
            n372 = call "Time Delay20"("error in (no error)"=w582, "Delay Time (s)"=w558) -> ("error out"=w563:errorcluster)  [unwired: 9 in]
            n373 = In Range and Coerce(upper limit=w576, x=w567, lower limit=w578) -> (In Range?=w575:bool)  [unwired: 1 out]
            n374 = To Double Precision Float(number=w567) -> (double precision float=w568:dbl)
            n375 = Decimal String To Number(string=w549, offset=0 ("offset (0)")) -> (number=w557:i32)  [unwired: 1 in, 1 out]
            n376 = Not Equal?(x=w549, y="") -> (x != y?=w550:bool)
            n377 = property on="R in Range" class="Bool (strict)"("Val(Sgnl)"=w575) -> ()  [unwired: 2 in, 2 out]
            n378 = property on="R Ready" class="Bool (strict)"("Val(Sgnl)"=w550) -> ()  [unwired: 2 in, 2 out]
            n379 = Divide(x=w568, y=w574) -> (x/y=w572:dbl)
            n380 = Number To Boolean Array(number=w557) -> (Boolean array=w556:bool[])
            n381 = property on="R deg/rev" class="DigNum (strict)"() -> ("Value"=w571:dbl)  [unwired: 2 in, 2 out]
            n382 = Index Array(array=w556, index=0) -> (element=w554:bool)
            n383 = Multiply(x=w572, y=w571) -> (x*y=w570:dbl)
            n384 = property on="R in Motion" class="Bool (strict)"("Val(Sgnl)"=w554) -> ()  [unwired: 2 in, 2 out]
            n385 = Add(x=w570, y=w569) -> (x+y=w566:dbl)
            n386 = property on="R Position deg PV" class="DigNum (strict)"("Val(Sgnl)"=w566) -> ()  [unwired: 2 in, 2 out]
          }
          frame #1 {
            n387 = property on="R Scan" class="Bool (strict)"() -> ("Value"=w588:bool)  [unwired: 2 in, 2 out]
            n388 = Or(x=w587, y=w588) -> (x .or. y?=w589:bool)
            n389 = case shown="True" w589 {
              frame #0 {
                n390 = property on="R Go" class="Bool"("DisabledEnum"=T2."Enabled" ("Disabled")) -> ()  [unwired: 2 in, 2 out]
                n391 = property on="R Scan OK" class="Bool"("DisabledEnum"=T2."Enabled" ("Disabled")) -> ()  [unwired: 2 in, 2 out]
              }
              frame #1 {
                n392 = property on="R Go" class="Bool"("DisabledEnum"=T2."Disabled and Grayed Out" ("Disabled")) -> ()  [unwired: 2 in, 2 out]
                n393 = property on="R Scan OK" class="Bool"("DisabledEnum"=T2."Disabled and Grayed Out" ("Disabled")) -> ()  [unwired: 2 in, 2 out]
              }
            }
          }
          frame #2 {
            n394 = case shown="False" w598 {
              tunnel: w599 -> [w605 w609]
              tunnel: [w606 w609] -> w600
              tunnel: [w607 w608] -> w601
              tunnel: w602 -> [w604 w608]
              frame #0 {
                n395 = call "mDrive Send Command.vi"("error in (no error)"=w604, "Command"=T1."Stop", "VISA resource name"=w605) -> ("error out"=w607:errorcluster, "VISA resource name out"=w606:refnum<visa-resource-name>)  [unwired: 4 in, 1 out]
              }
              frame #1 {
              }
            }
          }
          frame #3 {
            n396 = property on="R Backlash corr" class="Bool (strict)"() -> ("Value"=w616:bool)  [unwired: 2 in, 2 out]
            n397 = Implies(1:w615, 2:w616) -> (0:w614:bool)
            n398 = case shown="False" w614 {
              tunnel: w613 -> [w623 w676]
              tunnel: w612 -> [w622 w677]
              tunnel: [w621 w676] -> w611
              tunnel: [w620 w677] -> w610
              frame #0 {
                # "Backlash"
                n399 = flat-sequence {
                  tunnel: [w638] -> w635
                  tunnel: [w640] -> w634
                  tunnel: [w639] -> w633
                  tunnel: w623 -> [w637]
                  tunnel: w622 -> [w636]
                  tunnel: w635 -> [w648]
                  tunnel: [w648] -> w632
                  tunnel: w634 -> [w647]
                  tunnel: w633 -> [w646]
                  tunnel: [w645] -> w631
                  tunnel: [w644] -> w630
                  tunnel: [w643] -> w619
                  tunnel: w632 -> [w658]
                  tunnel: w631 -> [w657]
                  tunnel: w630 -> [w655]
                  tunnel: [w656] -> w629
                  tunnel: [w655] -> w628
                  tunnel: [w654] -> w625
                  tunnel: [w653] -> w624
                  tunnel: w619 -> [w653]
                  tunnel: w629 -> [w669]
                  tunnel: w628 -> [w662]
                  tunnel: [w669] -> w627
                  tunnel: [w668] -> w626
                  tunnel: w625 -> [w668]
                  tunnel: w624 -> [w664]
                  tunnel: [w663] -> w617
                  tunnel: w627 -> [w673]
                  tunnel: w626 -> [w672]
                  tunnel: [w671] -> w621
                  tunnel: [w670] -> w618
                  tunnel: w617 -> [w670]
                  tunnel: [w675] -> w620
                  tunnel: w618 -> [w675]
                  frame #0 {
                    n400 = property on="R Backlash steps/sec" class="DigNum (strict)"() -> ("Value"=w638:i32)  [unwired: 2 in, 2 out]
                    n401 = Number To Decimal String(number=w638) -> (decimal integer string=w641:string)  [unwired: 1 in]
                    n402 = call "mDrive Send Command.vi"("error in (no error)"=w637, "Extra"=w641, "Command"=T1."Max Velocity", "VISA resource name"=w636) -> ("error out"=w639:errorcluster, "VISA resource name out"=w640:refnum<visa-resource-name>)  [unwired: 3 in, 1 out]
                  }
                  frame #1 {
                    n403 = property on="R Backlash" class="DigNum (strict)"() -> ("Value"=w643:i32)  [unwired: 2 in, 2 out]
                    n404 = Number To Decimal String(number=w643) -> (decimal integer string=w649:string)  [unwired: 1 in]
                    n405 = call "mDrive Send Command.vi"("error in (no error)"=w646, "Extra"=w649, "Command"=T1."Move to Relative Position", "VISA resource name"=w647) -> ("error out"=w645:errorcluster, "VISA resource name out"=w644:refnum<visa-resource-name>)  [unwired: 3 in, 1 out]
                  }
                  frame #2 {
                    n406 = To Double Precision Float(number=w653) -> (double precision float=w651:dbl)
                    n407 = To Double Precision Float(number=w658) -> (double precision float=w660:dbl)
                    n408 = Absolute Value(x=w651) -> (abs(x)=w652:dbl)
                    n409 = Divide(x=w652, y=w660) -> (x/y=w661:dbl)
                    n410 = Add(x=w661, y=0.3) -> (x+y=w654:dbl)
                    n411 = call "Time Delay22"("error in (no error)"=w657, "Delay Time (s)"=w654) -> ("error out"=w656:errorcluster)  [unwired: 9 in]
                  }
                  frame #3 {
                    n412 = Negate(x=w664) -> (-x=w665:i32)
                    n413 = Number To Decimal String(number=w665) -> (decimal integer string=w666:string)  [unwired: 1 in]
                    n414 = call "mDrive Send Command.vi"("Extra"=w666, "Command"=T1."Move to Relative Position", "VISA resource name"=w662) -> ("VISA resource name out"=w663:refnum<visa-resource-name>)  [unwired: 4 in, 2 out]
                  }
                  frame #4 {
                    n415 = call "Time Delay23"("error in (no error)"=w673, "Delay Time (s)"=w672) -> ("error out"=w671:errorcluster)  [unwired: 9 in]
                  }
                  frame #5 {
                    n416 = property on="R Backlash corr" class="Bool (strict)"("Val(Sgnl)"=FALSE ("Value (Signaling)")) -> ()  [unwired: 2 in, 2 out]
                  }
                }
              }
              frame #1 {
              }
            }
          }
        }
        n417 = property on="X Position mm PV" class="DigNum (strict)"() -> ("Value"=w487:dbl)  [unwired: 2 in, 2 out]
        n418 = property on="Y Position mm PV" class="DigNum (strict)"() -> ("Value"=w480:dbl)  [unwired: 2 in, 2 out]
        n419 = property on="Z Position mm PV" class="DigNum (strict)"() -> ("Value"=w481:dbl)  [unwired: 2 in, 2 out]
        n420 = property on="R Position deg PV" class="DigNum (strict)"() -> ("Value"=w488:dbl)  [unwired: 2 in, 2 out]
        n421 = property on="Y Scan Length SP steps" class="DigNum (strict)"() -> ("Value"=w472:i32)  [unwired: 2 in, 2 out]
        n422 = property on="Z Scan Length SP steps" class="DigNum (strict)"() -> ("Value"=w473:i32)  [unwired: 2 in, 2 out]
        n423 = Divide(x=w472, y=w473) -> (x/y=w474:dbl)
        n424 = call "Build XY Graph"("Reset"=TRUE, "Y Input"=w480, "X Input"=w487) -> ("XY Graph"=→"XY Graph":cluster{"Y":dbl[], "Y":dbl[]}[])  [unwired: 7 in, 1 out]
        n425 = call "Build XY Graph2"("Reset"=TRUE, "Y Input"=w488, "X Input"=w481) -> ("XY Graph"=→"ZR Graph":cluster{"Y":dbl[], "Y":dbl[]}[])  [unwired: 7 in, 1 out]
        n426 = property on="Clear ZY" class="Bool (strict)"() -> ("Value"=w471:bool)  [unwired: 2 in, 2 out]
        n427 = call "Build XY Graph3"("Reset"=w471, "Y Input"=w480, "X Input"=w481) -> ("XY Graph"=→"ZY Graph":cluster{"Y":dbl[], "Y":dbl[]}[])  [unwired: 7 in, 1 out]
        n428 = Inverse Tangent(1:w474) -> (0:w475:dbl)
        n429 = Divide(x=w475, y=6.283185307179586) -> (x/y=w476:dbl)
        n430 = Multiply(x=360.0, y=w476) -> (x*y=w479:dbl)
        n431 = property on="atan Y/Z" class="DigNum (strict)"("Val(Sgnl)"=w479) -> ()  [unwired: 2 in, 2 out]
      }
      event #1 {
        n432 = event-data() -> ()  [unwired: 1 in, 5 out]
        n433 = property on="Z steps/rev" class="DigNum (strict)"() -> ("Value"=w1047:u32)  [unwired: 2 in, 2 out]
        n434 = property on="R steps/rev" class="DigNum (strict)"() -> ("Value"=w1038:u32)  [unwired: 2 in, 2 out]
        n435 = property on="X steps/rev" class="DigNum (strict)"() -> ("Value"=w1056:u32)  [unwired: 2 in, 2 out]
        n436 = property on="Y steps/rev" class="DigNum (strict)"() -> ("Value"=w1065:u32)  [unwired: 2 in, 2 out]
        n437 = property on="Z offset mm" class="DigNum (strict)"() -> ("Value"=w1045:dbl)  [unwired: 2 in, 2 out]
        n438 = property on="R offset deg" class="DigNum (strict)"() -> ("Value"=w1036:dbl)  [unwired: 2 in, 2 out]
        n439 = property on="X offset mm" class="DigNum (strict)"() -> ("Value"=w1054:dbl)  [unwired: 2 in, 2 out]
        n440 = property on="Y offset mm" class="DigNum (strict)"() -> ("Value"=w1063:dbl)  [unwired: 2 in, 2 out]
        n441 = property on="Reset R Position deg" class="DigNum (strict)"() -> ("Value"=w1044:dbl)  [unwired: 2 in, 2 out]
        n442 = property on="Reset Z Position mm" class="DigNum (strict)"() -> ("Value"=w1053:dbl)  [unwired: 2 in, 2 out]
        n443 = property on="Reset X Position mm" class="DigNum (strict)"() -> ("Value"=w1062:dbl)  [unwired: 2 in, 2 out]
        n444 = property on="Reset Y Position mm" class="DigNum (strict)"() -> ("Value"=w1071:dbl)  [unwired: 2 in, 2 out]
        n445 = To Double Precision Float(number=w1038) -> (double precision float=w1041:dbl)
        n446 = To Double Precision Float(number=w1056) -> (double precision float=w1059:dbl)
        n447 = To Double Precision Float(number=w1065) -> (double precision float=w1068:dbl)
        n448 = Subtract(x=w1053, y=w1045) -> (x-y=w1052:dbl)
        n449 = Subtract(x=w1044, y=w1036) -> (x-y=w1043:dbl)
        n450 = Subtract(x=w1062, y=w1054) -> (x-y=w1061:dbl)
        n451 = Subtract(x=w1071, y=w1063) -> (x-y=w1070:dbl)
        n452 = property on="R deg/rev" class="DigNum (strict)"() -> ("Value"=w1037:dbl)  [unwired: 2 in, 2 out]
        n453 = property on="Z mm/rev" class="DigNum (strict)"() -> ("Value"=w1046:dbl)  [unwired: 2 in, 2 out]
        n454 = property on="X mm/rev" class="DigNum (strict)"() -> ("Value"=w1055:dbl)  [unwired: 2 in, 2 out]
        n455 = property on="Y mm/rev" class="DigNum (strict)"() -> ("Value"=w1064:dbl)  [unwired: 2 in, 2 out]
        n456 = Divide(x=w1043, y=w1037) -> (x/y=w1042:dbl)
        n457 = Divide(x=w1061, y=w1055) -> (x/y=w1060:dbl)
        n458 = Divide(x=w1070, y=w1064) -> (x/y=w1069:dbl)
        n459 = Divide(x=w1052, y=w1046) -> (x/y=w1051:dbl)
        n460 = To Double Precision Float(number=w1047) -> (double precision float=w1050:dbl)
        n461 = Multiply(x=w1051, y=w1050) -> (x*y=w1049:dbl)
        n462 = Multiply(x=w1042, y=w1041) -> (x*y=w1040:dbl)
        n463 = Multiply(x=w1060, y=w1059) -> (x*y=w1058:dbl)
        n464 = Multiply(x=w1069, y=w1068) -> (x*y=w1067:dbl)
        n465 = To Long Integer(number=w1049) -> (32bit integer=w1048:i32)
        n466 = To Long Integer(number=w1040) -> (32bit integer=w1039:i32)
        n467 = To Long Integer(number=w1058) -> (32bit integer=w1057:i32)
        n468 = To Long Integer(number=w1067) -> (32bit integer=w1066:i32)
        n469 = property on="Reset Z Motor Steps" class="DigNum (strict)"("Val(Sgnl)"=w1048) -> ()  [unwired: 2 in, 2 out]
        n470 = property on="Reset R Motor Steps" class="DigNum (strict)"("Val(Sgnl)"=w1039) -> ()  [unwired: 2 in, 2 out]
        n471 = property on="Reset X Motor Steps" class="DigNum (strict)"("Val(Sgnl)"=w1057) -> ()  [unwired: 2 in, 2 out]
        n472 = property on="Reset Y Motor Steps" class="DigNum (strict)"("Val(Sgnl)"=w1066) -> ()  [unwired: 2 in, 2 out]
      }
      event #2 {
        n473 = event-data() -> ()  [unwired: 1 in, 5 out]
        n474 = property on="Y Step SP" class="DigNum (strict)"() -> ("Value"=w1104:i32)  [unwired: 2 in, 2 out]
        n475 = property on="X Step SP" class="DigNum (strict)"() -> ("Value"=w1096:i32)  [unwired: 2 in, 2 out]
        n476 = property on="Z Step SP" class="DigNum (strict)"() -> ("Value"=w1088:i32)  [unwired: 2 in, 2 out]
        n477 = property on="R Step SP" class="DigNum (strict)"() -> ("Value"=w1080:i32)  [unwired: 2 in, 2 out]
        n478 = property on="Y steps/rev" class="DigNum (strict)"() -> ("Value"=w1127:u32)  [unwired: 2 in, 2 out]
        n479 = property on="Y steps/rev" class="DigNum (strict)"() -> ("Value"=w1102:u32)  [unwired: 2 in, 2 out]
        n480 = property on="X steps/rev" class="DigNum (strict)"() -> ("Value"=w1121:u32)  [unwired: 2 in, 2 out]
        n481 = property on="X steps/rev" class="DigNum (strict)"() -> ("Value"=w1094:u32)  [unwired: 2 in, 2 out]
        n482 = property on="Z steps/rev" class="DigNum (strict)"() -> ("Value"=w1115:u32)  [unwired: 2 in, 2 out]
        n483 = property on="Z steps/rev" class="DigNum (strict)"() -> ("Value"=w1086:u32)  [unwired: 2 in, 2 out]
        n484 = property on="R steps/rev" class="DigNum (strict)"() -> ("Value"=w1109:u32)  [unwired: 2 in, 2 out]
        n485 = property on="R steps/rev" class="DigNum (strict)"() -> ("Value"=w1078:u32)  [unwired: 2 in, 2 out]
        n486 = property on="Y offset mm" class="DigNum (strict)"() -> ("Value"=w1101:dbl)  [unwired: 2 in, 2 out]
        n487 = property on="X offset mm" class="DigNum (strict)"() -> ("Value"=w1093:dbl)  [unwired: 2 in, 2 out]
        n488 = property on="Z offset mm" class="DigNum (strict)"() -> ("Value"=w1085:dbl)  [unwired: 2 in, 2 out]
        n489 = property on="R offset deg" class="DigNum (strict)"() -> ("Value"=w1077:dbl)  [unwired: 2 in, 2 out]
        n490 = property on="Y Velocity SP step/sec" class="DigNum (strict)"() -> ("Value"=w1129:i32)  [unwired: 2 in, 2 out]
        n491 = property on="X Velocity SP step/sec" class="DigNum (strict)"() -> ("Value"=w1123:i32)  [unwired: 2 in, 2 out]
        n492 = property on="Z Velocity SP step/sec" class="DigNum (strict)"() -> ("Value"=w1117:i32)  [unwired: 2 in, 2 out]
        n493 = property on="R Velocity SP step/sec" class="DigNum (strict)"() -> ("Value"=w1111:i32)  [unwired: 2 in, 2 out]
        n494 = To Double Precision Float(number=w1104) -> (double precision float=w1105:dbl)
        n495 = To Double Precision Float(number=w1102) -> (double precision float=w1108:dbl)
        n496 = To Double Precision Float(number=w1121) -> (double precision float=w1126:dbl)
        n497 = To Double Precision Float(number=w1096) -> (double precision float=w1097:dbl)
        n498 = To Double Precision Float(number=w1094) -> (double precision float=w1100:dbl)
        n499 = To Double Precision Float(number=w1115) -> (double precision float=w1120:dbl)
        n500 = To Double Precision Float(number=w1088) -> (double precision float=w1089:dbl)
        n501 = To Double Precision Float(number=w1086) -> (double precision float=w1092:dbl)
        n502 = To Double Precision Float(number=w1109) -> (double precision float=w1114:dbl)
        n503 = To Double Precision Float(number=w1080) -> (double precision float=w1081:dbl)
        n504 = To Double Precision Float(number=w1078) -> (double precision float=w1084:dbl)
        n505 = Divide(x=w1081, y=w1084) -> (x/y=w1083:dbl)
        n506 = Divide(x=w1105, y=w1108) -> (x/y=w1107:dbl)
        n507 = Divide(x=w1097, y=w1100) -> (x/y=w1099:dbl)
        n508 = Divide(x=w1089, y=w1092) -> (x/y=w1091:dbl)
        n509 = To Double Precision Float(number=w1111) -> (double precision float=w1112:dbl)
        n510 = To Double Precision Float(number=w1129) -> (double precision float=w1130:dbl)
        n511 = To Double Precision Float(number=w1127) -> (double precision float=w1132:dbl)
        n512 = To Double Precision Float(number=w1123) -> (double precision float=w1124:dbl)
        n513 = To Double Precision Float(number=w1117) -> (double precision float=w1118:dbl)
        n514 = property on="R deg/rev" class="DigNum (strict)"() -> ("Value"=w1076:dbl)  [unwired: 2 in, 2 out]
        n515 = property on="Y mm/rev" class="DigNum (strict)"() -> ("Value"=w1073:dbl)  [unwired: 2 in, 2 out]
        n516 = property on="X mm/rev" class="DigNum (strict)"() -> ("Value"=w1074:dbl)  [unwired: 2 in, 2 out]
        n517 = property on="Z mm/rev" class="DigNum (strict)"() -> ("Value"=w1075:dbl)  [unwired: 2 in, 2 out]
        n518 = Divide(x=w1130, y=w1132) -> (x/y=w1131:dbl)
        n519 = Multiply(x=w1107, y=w1073) -> (x*y=w1106:dbl)
        n520 = Divide(x=w1124, y=w1126) -> (x/y=w1125:dbl)
        n521 = Multiply(x=w1099, y=w1074) -> (x*y=w1098:dbl)
        n522 = Divide(x=w1118, y=w1120) -> (x/y=w1119:dbl)
        n523 = Multiply(x=w1091, y=w1075) -> (x*y=w1090:dbl)
        n524 = Divide(x=w1112, y=w1114) -> (x/y=w1113:dbl)
        n525 = Multiply(x=w1083, y=w1076) -> (x*y=w1082:dbl)
        n526 = Multiply(x=w1131, y=w1073) -> (x*y=w1128:dbl)
        n527 = Add(x=w1106, y=w1101) -> (x+y=w1103:dbl)
        n528 = Multiply(x=w1125, y=w1074) -> (x*y=w1122:dbl)
        n529 = Add(x=w1098, y=w1093) -> (x+y=w1095:dbl)
        n530 = Multiply(x=w1119, y=w1075) -> (x*y=w1116:dbl)
        n531 = Add(x=w1090, y=w1085) -> (x+y=w1087:dbl)
        n532 = Multiply(x=w1113, y=w1076) -> (x*y=w1110:dbl)
        n533 = Add(x=w1082, y=w1077) -> (x+y=w1079:dbl)
        n534 = Absolute Value(x=w1110) -> (abs(x)=w1072:dbl)
        n535 = property on="Y Velocity MV mm/sec" class="DigNum (strict)"("Val(Sgnl)"=w1128) -> ()  [unwired: 2 in, 2 out]
        n536 = property on="Y Position MV mm" class="DigNum (strict)"("Val(Sgnl)"=w1103) -> ()  [unwired: 2 in, 2 out]
        n537 = property on="X Velocity MV mm/sec" class="DigNum (strict)"("Val(Sgnl)"=w1122) -> ()  [unwired: 2 in, 2 out]
        n538 = property on="X Position MV mm" class="DigNum (strict)"("Val(Sgnl)"=w1095) -> ()  [unwired: 2 in, 2 out]
        n539 = property on="Z Velocity MV mm/sec" class="DigNum (strict)"("Val(Sgnl)"=w1116) -> ()  [unwired: 2 in, 2 out]
        n540 = property on="Z Position MV mm" class="DigNum (strict)"("Val(Sgnl)"=w1087) -> ()  [unwired: 2 in, 2 out]
        n541 = property on="R Position MV deg" class="DigNum (strict)"("Val(Sgnl)"=w1079) -> ()  [unwired: 2 in, 2 out]
        n542 = property on="R Velocity MVdeg/sec" class="DigNum (strict)"("Val(Sgnl)"=w1072) -> ()  [unwired: 2 in, 2 out]
      }
      event #3 {
        n543 = event-data() -> ()  [unwired: 1 in, 5 out]
        n544 = property on="X Step PV" class="DigNum (strict)"() -> ("Value"=w1201:i32)  [unwired: 2 in, 2 out]
        n545 = property on="Y Step PV" class="DigNum (strict)"() -> ("Value"=w1187:i32)  [unwired: 2 in, 2 out]
        n546 = property on="Z Step PV" class="DigNum (strict)"() -> ("Value"=w1174:i32)  [unwired: 2 in, 2 out]
        n547 = property on="R Step PV" class="DigNum (strict)"() -> ("Value"=w1160:i32)  [unwired: 2 in, 2 out]
        n548 = property on="X Step SP" class="DigNum (strict)"() -> ("Minimum"=w1208:dbl)  [unwired: 2 in, 2 out]
        n549 = property on="X Step SP" class="DigNum (strict)"() -> ("Maximum"=w1207:dbl)  [unwired: 2 in, 2 out]
        n550 = property on="Y Step SP" class="DigNum (strict)"() -> ("Minimum"=w1194:dbl)  [unwired: 2 in, 2 out]
        n551 = property on="Y Step SP" class="DigNum (strict)"() -> ("Maximum"=w1193:dbl)  [unwired: 2 in, 2 out]
        n552 = property on="Z Step SP" class="DigNum (strict)"() -> ("Minimum"=w1181:dbl)  [unwired: 2 in, 2 out]
        n553 = property on="Z Step SP" class="DigNum (strict)"() -> ("Maximum"=w1180:dbl)  [unwired: 2 in, 2 out]
        n554 = property on="R Step SP" class="DigNum (strict)"() -> ("Minimum"=w1165:dbl)  [unwired: 2 in, 2 out]
        n555 = property on="R Step SP" class="DigNum (strict)"() -> ("Maximum"=w1168:dbl)  [unwired: 2 in, 2 out]
        n556 = property on="Z steps/rev" class="DigNum (strict)"() -> ("Value"=w1176:u32)  [unwired: 2 in, 2 out]
        n557 = property on="R steps/rev" class="DigNum (strict)"() -> ("Value"=w1162:u32)  [unwired: 2 in, 2 out]
        n558 = property on="X steps/rev" class="DigNum (strict)"() -> ("Value"=w1203:u32)  [unwired: 2 in, 2 out]
        n559 = property on="Y steps/rev" class="DigNum (strict)"() -> ("Value"=w1189:u32)  [unwired: 2 in, 2 out]
        n560 = To Double Precision Float(number=w1201) -> (double precision float=w1154:dbl)
        n561 = To Double Precision Float(number=w1187) -> (double precision float=w1153:dbl)
        n562 = To Double Precision Float(number=w1174) -> (double precision float=w1152:dbl)
        n563 = To Double Precision Float(number=w1160) -> (double precision float=w1151:dbl)
        n564 = Subtract(x=w1208, y=w1154) -> (x-y=w1209:dbl)
        n565 = Subtract(x=w1207, y=w1154) -> (x-y=w1206:dbl)
        n566 = Subtract(x=w1194, y=w1153) -> (x-y=w1195:dbl)
        n567 = Subtract(x=w1193, y=w1153) -> (x-y=w1192:dbl)
        n568 = Subtract(x=w1181, y=w1152) -> (x-y=w1182:dbl)
        n569 = Subtract(x=w1180, y=w1152) -> (x-y=w1179:dbl)
        n570 = Subtract(x=w1165, y=w1151) -> (x-y=w1166:dbl)
        n571 = Subtract(x=w1168, y=w1151) -> (x-y=w1167:dbl)
        n572 = property on="Z Scan Length SP steps" class="DigNum (strict)"() -> ("Value"=w1177:i32)  [unwired: 2 in, 2 out]
        n573 = To Double Precision Float(number=w1176) -> (double precision float=w1173:dbl)
        n574 = property on="R Scan Length SP steps" class="DigNum (strict)"() -> ("Value"=w1163:i32)  [unwired: 2 in, 2 out]
        n575 = To Double Precision Float(number=w1162) -> (double precision float=w1159:dbl)
        n576 = To Double Precision Float(number=w1203) -> (double precision float=w1200:dbl)
        n577 = property on="X Scan Length SP steps" class="DigNum (strict)"() -> ("Value"=w1199:i32)  [unwired: 2 in, 2 out]
        n578 = property on="Y Scan Length SP steps" class="DigNum (strict)"() -> ("Value"=w1190:i32)  [unwired: 2 in, 2 out]
        n579 = To Double Precision Float(number=w1189) -> (double precision float=w1144:dbl)
        n580 = property on="Z Scan Velocity SP steps/sec" class="DigNum (strict)"() -> ("Value"=w1172:i32)  [unwired: 2 in, 2 out]
        n581 = property on="R Scan Velocity SP steps/sec" class="DigNum (strict)"() -> ("Value"=w1158:i32)  [unwired: 2 in, 2 out]
        n582 = property on="X Scan Velocity SP steps/sec" class="DigNum (strict)"() -> ("Value"=w1204:i32)  [unwired: 2 in, 2 out]
        n583 = property on="Y Scan Velocity SP steps/sec" class="DigNum (strict)"() -> ("Value"=w1186:i32)  [unwired: 2 in, 2 out]
        n584 = To Double Precision Float(number=w1177) -> (double precision float=w1150:dbl)
        n585 = To Double Precision Float(number=w1163) -> (double precision float=w1148:dbl)
        n586 = property on="X Scan Length SP steps" class="DigNum (strict)"("Minimum"=w1209) -> ()  [unwired: 2 in, 2 out]
        n587 = property on="X Scan Length SP steps" class="DigNum (strict)"("Maximum"=w1206) -> ()  [unwired: 2 in, 2 out]
        n588 = property on="Y Scan Length SP steps" class="DigNum (strict)"("Minimum"=w1195) -> ()  [unwired: 2 in, 2 out]
        n589 = property on="Y Scan Length SP steps" class="DigNum (strict)"("Maximum"=w1192) -> ()  [unwired: 2 in, 2 out]
        n590 = property on="Z Scan Length SP steps" class="DigNum (strict)"("Minimum"=w1182) -> ()  [unwired: 2 in, 2 out]
        n591 = property on="Z Scan Length SP steps" class="DigNum (strict)"("Maximum"=w1179) -> ()  [unwired: 2 in, 2 out]
        n592 = property on="R Scan Length SP steps" class="DigNum (strict)"("Minimum"=w1166) -> ()  [unwired: 2 in, 2 out]
        n593 = property on="R Scan Length SP steps" class="DigNum (strict)"("Maximum"=w1167) -> ()  [unwired: 2 in, 2 out]
        n594 = To Double Precision Float(number=w1199) -> (double precision float=w1139:dbl)
        n595 = To Double Precision Float(number=w1190) -> (double precision float=w1143:dbl)
        n596 = Divide(x=w1148, y=w1159) -> (x/y=w1164:dbl)
        n597 = Divide(x=w1150, y=w1173) -> (x/y=w1178:dbl)
        n598 = Divide(x=w1139, y=w1200) -> (x/y=w1198:dbl)
        n599 = Divide(x=w1143, y=w1144) -> (x/y=w1191:dbl)
        n600 = To Double Precision Float(number=w1158) -> (double precision float=w1147:dbl)
        n601 = property on="R deg/rev" class="DigNum (strict)"() -> ("Value"=w1161:dbl)  [unwired: 2 in, 2 out]
        n602 = To Double Precision Float(number=w1172) -> (double precision float=w1149:dbl)
        n603 = To Double Precision Float(number=w1204) -> (double precision float=w1138:dbl)
        n604 = To Double Precision Float(number=w1186) -> (double precision float=w1142:dbl)
        n605 = property on="Z mm/rev" class="DigNum (strict)"() -> ("Value"=w1175:dbl)  [unwired: 2 in, 2 out]
        n606 = property on="X mm/rev" class="DigNum (strict)"() -> ("Value"=w1202:dbl)  [unwired: 2 in, 2 out]
        n607 = property on="Y mm/rev" class="DigNum (strict)"() -> ("Value"=w1188:dbl)  [unwired: 2 in, 2 out]
        n608 = Multiply(x=w1178, y=w1175) -> (x*y=w1170:dbl)
        n609 = Divide(x=w1150, y=w1149) -> (x/y=w1145:dbl)
        n610 = Divide(x=w1149, y=w1173) -> (x/y=w1171:dbl)
        n611 = Multiply(x=w1164, y=w1161) -> (x*y=w1156:dbl)
        n612 = Divide(x=w1148, y=w1147) -> (x/y=w1146:dbl)
        n613 = Divide(x=w1147, y=w1159) -> (x/y=w1157:dbl)
        n614 = Divide(x=w1139, y=w1138) -> (x/y=w1140:dbl)
        n615 = Divide(x=w1138, y=w1200) -> (x/y=w1205:dbl)
        n616 = Multiply(x=w1202, y=w1198) -> (x*y=w1196:dbl)
        n617 = Multiply(x=w1191, y=w1188) -> (x*y=w1184:dbl)
        n618 = Divide(x=w1143, y=w1142) -> (x/y=w1141:dbl)
        n619 = Divide(x=w1142, y=w1144) -> (x/y=w1185:dbl)
        n620 = Multiply(x=w1175, y=w1171) -> (x*y=w1169:dbl)
        n621 = Multiply(x=w1161, y=w1157) -> (x*y=w1155:dbl)
        n622 = Multiply(x=w1205, y=w1202) -> (x*y=w1197:dbl)
        n623 = Multiply(x=w1188, y=w1185) -> (x*y=w1183:dbl)
        n624 = Absolute Value(x=w1145) -> (abs(x)=→"Z Scan Duration":dbl)
        n625 = Absolute Value(x=w1146) -> (abs(x)=→"R Scan Duration":dbl)
        n626 = Absolute Value(x=w1140) -> (abs(x)=→"X Scan Duration":dbl)
        n627 = Absolute Value(x=w1141) -> (abs(x)=→"Y Scan Duration":dbl)
        n628 = property on="Z Scan length MV mm" class="DigNum (strict)"("Value"=w1170) -> ()  [unwired: 2 in, 2 out]
        n629 = property on="R Scan length MV deg" class="DigNum (strict)"("Value"=w1156) -> ()  [unwired: 2 in, 2 out]
        n630 = property on="X Scan length MV mm" class="DigNum (strict)"("Val(Sgnl)"=w1196) -> ()  [unwired: 2 in, 2 out]
        n631 = property on="Y Scan length MV mm" class="DigNum (strict)"("Value"=w1184) -> ()  [unwired: 2 in, 2 out]
        n632 = Absolute Value(x=w1155) -> (abs(x)=w1137:dbl)
        n633 = property on="Z Scan velocity MV mm/sec" class="DigNum (strict)"("Val(Sgnl)"=w1169) -> ()  [unwired: 2 in, 2 out]
        n634 = property on="X Scan velocity MV mm/sec" class="DigNum (strict)"("Value"=w1197) -> ()  [unwired: 2 in, 2 out]
        n635 = property on="Y Scan velocity MV mm/sec" class="DigNum (strict)"("Val(Sgnl)"=w1183) -> ()  [unwired: 2 in, 2 out]
        n636 = property on="R Scan Velocity SP deg/sec" class="DigNum (strict)"("Val(Sgnl)"=w1137) -> ()  [unwired: 2 in, 2 out]
      }
      event #4 {
        n637 = event-data() -> ()  [unwired: 1 in, 7 out]
        n638 = property on="Y Step SP" class="DigNum (strict)"() -> ("Maximum"=w1220:dbl)  [unwired: 2 in, 2 out]
        n639 = property on="Y Step SP" class="DigNum (strict)"() -> ("Minimum"=w1219:dbl)  [unwired: 2 in, 2 out]
        n640 = property on="Y steps/rev" class="DigNum (strict)"() -> ("Value"=w1226:u32)  [unwired: 2 in, 2 out]
        n641 = property on="Y offset mm" class="DigNum (strict)"() -> ("Value"=w1224:dbl)  [unwired: 2 in, 2 out]
        n642 = property on="Y Velocity SP step/sec" class="DigNum (strict)"() -> ("Maximum"=w1213:dbl)  [unwired: 2 in, 2 out]
        n643 = property on="Y Velocity SP step/sec" class="DigNum (strict)"() -> ("Minimum"=w1212:dbl)  [unwired: 2 in, 2 out]
        n644 = property on="Y Position SP mm" class="DigNum (strict)"() -> ("Value"=w1223:dbl)  [unwired: 2 in, 2 out]
        n645 = property on="Y mm/rev" class="DigNum (strict)"() -> ("Value"=w1210:dbl)  [unwired: 2 in, 2 out]
        n646 = property on="Y Velocity SP mm/sec" class="DigNum (strict)"() -> ("Value"=w1217:dbl)  [unwired: 2 in, 2 out]
        n647 = Subtract(x=w1223, y=w1224) -> (x-y=w1227:dbl)
        n648 = Divide(x=w1217, y=w1210) -> (x/y=w1218:dbl)
        n649 = To Double Precision Float(number=w1226) -> (double precision float=w1211:dbl)
        n650 = Divide(x=w1227, y=w1210) -> (x/y=w1228:dbl)
        n651 = Multiply(x=w1218, y=w1211) -> (x*y=w1215:dbl)
        n652 = Multiply(x=w1228, y=w1211) -> (x*y=w1222:dbl)
        n653 = In Range and Coerce(upper limit=w1213, x=w1215, lower limit=w1212) -> (coerced(x)=w1214:dbl)  [unwired: 1 out]
        n654 = To Long Integer(number=w1214) -> (32bit integer=w1216:i32)
        n655 = In Range and Coerce(upper limit=w1220, x=w1222, lower limit=w1219) -> (coerced(x)=w1221:dbl)  [unwired: 1 out]
        n656 = To Long Integer(number=w1221) -> (32bit integer=w1225:i32)
        n657 = property on="Y Velocity SP step/sec" class="DigNum (strict)"("Val(Sgnl)"=w1216) -> ()  [unwired: 2 in, 2 out]
        n658 = property on="Y Step SP" class="DigNum (strict)"("Val(Sgnl)"=w1225) -> ()  [unwired: 2 in, 2 out]
      }
      event #5 {
        n659 = event-data() -> ()  [unwired: 1 in, 7 out]
        n660 = property on="X Step SP" class="DigNum (strict)"() -> ("Maximum"=w1239:dbl)  [unwired: 2 in, 2 out]
        n661 = property on="X Step SP" class="DigNum (strict)"() -> ("Minimum"=w1238:dbl)  [unwired: 2 in, 2 out]
        n662 = property on="X steps/rev" class="DigNum (strict)"() -> ("Value"=w1245:u32)  [unwired: 2 in, 2 out]
        n663 = property on="X offset mm" class="DigNum (strict)"() -> ("Value"=w1243:dbl)  [unwired: 2 in, 2 out]
        n664 = property on="X Velocity SP step/sec" class="DigNum (strict)"() -> ("Maximum"=w1232:dbl)  [unwired: 2 in, 2 out]
        n665 = property on="X Velocity SP step/sec" class="DigNum (strict)"() -> ("Minimum"=w1231:dbl)  [unwired: 2 in, 2 out]
        n666 = property on="X Position SP mm" class="DigNum (strict)"() -> ("Value"=w1242:dbl)  [unwired: 2 in, 2 out]
        n667 = property on="X mm/rev" class="DigNum (strict)"() -> ("Value"=w1229:dbl)  [unwired: 2 in, 2 out]
        n668 = property on="X Velocity SP mm/sec" class="DigNum (strict)"() -> ("Value"=w1236:dbl)  [unwired: 2 in, 2 out]
        n669 = Subtract(x=w1242, y=w1243) -> (x-y=w1246:dbl)
        n670 = Divide(x=w1236, y=w1229) -> (x/y=w1237:dbl)
        n671 = To Double Precision Float(number=w1245) -> (double precision float=w1230:dbl)
        n672 = Divide(x=w1246, y=w1229) -> (x/y=w1247:dbl)
        n673 = Multiply(x=w1237, y=w1230) -> (x*y=w1234:dbl)
        n674 = Multiply(x=w1247, y=w1230) -> (x*y=w1241:dbl)
        n675 = In Range and Coerce(upper limit=w1232, x=w1234, lower limit=w1231) -> (coerced(x)=w1233:dbl)  [unwired: 1 out]
        n676 = To Long Integer(number=w1233) -> (32bit integer=w1235:i32)
        n677 = In Range and Coerce(upper limit=w1239, x=w1241, lower limit=w1238) -> (coerced(x)=w1240:dbl)  [unwired: 1 out]
        n678 = To Long Integer(number=w1240) -> (32bit integer=w1244:i32)
        n679 = property on="X Velocity SP step/sec" class="DigNum (strict)"("Val(Sgnl)"=w1235) -> ()  [unwired: 2 in, 2 out]
        n680 = property on="X Step SP" class="DigNum (strict)"("Val(Sgnl)"=w1244) -> ()  [unwired: 2 in, 2 out]
      }
      event #6 {
        n681 = event-data() -> ()  [unwired: 1 in, 7 out]
        n682 = property on="Z Step SP" class="DigNum (strict)"() -> ("Maximum"=w1256:dbl)  [unwired: 2 in, 2 out]
        n683 = property on="Z Step SP" class="DigNum (strict)"() -> ("Minimum"=w1255:dbl)  [unwired: 2 in, 2 out]
        n684 = property on="Z steps/rev" class="DigNum (strict)"() -> ("Value"=w1262:u32)  [unwired: 2 in, 2 out]
        n685 = property on="Z offset mm" class="DigNum (strict)"() -> ("Value"=w1260:dbl)  [unwired: 2 in, 2 out]
        n686 = property on="Z Velocity SP step/sec" class="DigNum (strict)"() -> ("Maximum"=w1249:dbl)  [unwired: 2 in, 2 out]
        n687 = property on="Z Velocity SP step/sec" class="DigNum (strict)"() -> ("Minimum"=w1248:dbl)  [unwired: 2 in, 2 out]
        n688 = property on="Z Position SP mm" class="DigNum (strict)"() -> ("Value"=w1259:dbl)  [unwired: 2 in, 2 out]
        n689 = property on="Z mm/rev" class="DigNum (strict)"() -> ("Value"=w1265:dbl)  [unwired: 2 in, 2 out]
        n690 = property on="Z Velocity SP mm/sec" class="DigNum (strict)"() -> ("Value"=w1253:dbl)  [unwired: 2 in, 2 out]
        n691 = Subtract(x=w1259, y=w1260) -> (x-y=w1263:dbl)
        n692 = Divide(x=w1253, y=w1265) -> (x/y=w1254:dbl)
        n693 = To Double Precision Float(number=w1262) -> (double precision float=w1266:dbl)
        n694 = Divide(x=w1263, y=w1265) -> (x/y=w1264:dbl)
        n695 = Multiply(x=w1254, y=w1266) -> (x*y=w1251:dbl)
        n696 = Multiply(x=w1264, y=w1266) -> (x*y=w1258:dbl)
        n697 = In Range and Coerce(upper limit=w1249, x=w1251, lower limit=w1248) -> (coerced(x)=w1250:dbl)  [unwired: 1 out]
        n698 = To Long Integer(number=w1250) -> (32bit integer=w1252:i32)
        n699 = In Range and Coerce(upper limit=w1256, x=w1258, lower limit=w1255) -> (coerced(x)=w1257:dbl)  [unwired: 1 out]
        n700 = To Long Integer(number=w1257) -> (32bit integer=w1261:i32)
        n701 = property on="Z Velocity SP step/sec" class="DigNum (strict)"("Val(Sgnl)"=w1252) -> ()  [unwired: 2 in, 2 out]
        n702 = property on="Z Step SP" class="DigNum (strict)"("Val(Sgnl)"=w1261) -> ()  [unwired: 2 in, 2 out]
      }
      event #7 {
        n703 = event-data() -> ()  [unwired: 1 in, 7 out]
        n704 = property on="R Step SP" class="DigNum (strict)"() -> ("Maximum"=w1278:dbl)  [unwired: 2 in, 2 out]
        n705 = property on="R Step SP" class="DigNum (strict)"() -> ("Minimum"=w1277:dbl)  [unwired: 2 in, 2 out]
        n706 = property on="R steps/rev" class="DigNum (strict)"() -> ("Value"=w1284:u32)  [unwired: 2 in, 2 out]
        n707 = property on="R offset deg" class="DigNum (strict)"() -> ("Value"=w1282:dbl)  [unwired: 2 in, 2 out]
        n708 = property on="R Velocity SP step/sec" class="DigNum (strict)"() -> ("Maximum"=w1271:dbl)  [unwired: 2 in, 2 out]
        n709 = property on="R Velocity SP step/sec" class="DigNum (strict)"() -> ("Minimum"=w1270:dbl)  [unwired: 2 in, 2 out]
        n710 = To Double Precision Float(number=w1284) -> (double precision float=w1269:dbl)
        n711 = property on="R Position SP deg" class="DigNum (strict)"() -> ("Value"=w1281:dbl)  [unwired: 2 in, 2 out]
        n712 = property on="R deg/rev" class="DigNum (strict)"() -> ("Value"=w1268:dbl)  [unwired: 2 in, 2 out]
        n713 = property on="R Velocity SP deg/sec" class="DigNum (strict)"() -> ("Value"=w1275:dbl)  [unwired: 2 in, 2 out]
        n714 = Subtract(x=w1281, y=w1282) -> (x-y=w1285:dbl)
        n715 = Divide(x=w1275, y=w1268) -> (x/y=w1276:dbl)
        n716 = Divide(x=w1285, y=w1268) -> (x/y=w1286:dbl)
        n717 = Multiply(x=w1276, y=w1269) -> (x*y=w1273:dbl)
        n718 = Multiply(x=w1286, y=w1269) -> (x*y=w1280:dbl)
        n719 = Absolute Value(x=w1273) -> (abs(x)=w1267:dbl)
        n720 = In Range and Coerce(upper limit=w1278, x=w1280, lower limit=w1277) -> (coerced(x)=w1279:dbl)  [unwired: 1 out]
        n721 = In Range and Coerce(upper limit=w1271, x=w1267, lower limit=w1270) -> (coerced(x)=w1272:dbl)  [unwired: 1 out]
        n722 = To Long Integer(number=w1279) -> (32bit integer=w1283:i32)
        n723 = To Long Integer(number=w1272) -> (32bit integer=w1274:i32)
        n724 = property on="R Step SP" class="DigNum (strict)"("Val(Sgnl)"=w1283) -> ()  [unwired: 2 in, 2 out]
        n725 = property on="R Velocity SP step/sec" class="DigNum (strict)"("Val(Sgnl)"=w1274) -> ()  [unwired: 2 in, 2 out]
      }
      event #8 {
        n726 = event-data() -> ()  [unwired: 1 in, 7 out]
        n727 = property on="Y Step SP" class="DigNum (strict)"() -> ("Maximum"=w1296:dbl)  [unwired: 2 in, 2 out]
        n728 = property on="Y Step SP" class="DigNum (strict)"() -> ("Minimum"=w1297:dbl)  [unwired: 2 in, 2 out]
        n729 = property on="Y steps/rev" class="DigNum (strict)"() -> ("Value"=w1302:u32)  [unwired: 2 in, 2 out]
        n730 = To Double Precision Float(number=w1302) -> (double precision float=w1288:dbl)
        n731 = property on="Y Scan Length SP mm" class="DigNum (strict)"() -> ("Value"=w1300:dbl)  [unwired: 2 in, 2 out]
        n732 = property on="Y mm/rev" class="DigNum (strict)"() -> ("Value"=w1287:dbl)  [unwired: 2 in, 2 out]
        n733 = property on="Y Scan Velocity SP steps/sec" class="DigNum (strict)"() -> ("Maximum"=w1290:dbl)  [unwired: 2 in, 2 out]
        n734 = property on="Y Scan Velocity SP steps/sec" class="DigNum (strict)"() -> ("Minimum"=w1289:dbl)  [unwired: 2 in, 2 out]
        n735 = property on="Y Scan Velocity SP mm/sec" class="DigNum (strict)"() -> ("Value"=w1294:dbl)  [unwired: 2 in, 2 out]
        n736 = Divide(x=w1300, y=w1287) -> (x/y=w1303:dbl)
        n737 = Multiply(x=w1303, y=w1288) -> (x*y=w1299:dbl)
        n738 = Divide(x=w1294, y=w1287) -> (x/y=w1295:dbl)
        n739 = Multiply(x=w1295, y=w1288) -> (x*y=w1292:dbl)
        n740 = In Range and Coerce(upper limit=w1296, x=w1299, lower limit=w1297) -> (coerced(x)=w1298:dbl)  [unwired: 1 out]
        n741 = To Long Integer(number=w1298) -> (32bit integer=w1301:i32)
        n742 = In Range and Coerce(upper limit=w1290, x=w1292, lower limit=w1289) -> (coerced(x)=w1291:dbl)  [unwired: 1 out]
        n743 = To Long Integer(number=w1291) -> (32bit integer=w1293:i32)
        n744 = property on="Y Scan Length SP steps" class="DigNum (strict)"("Val(Sgnl)"=w1301) -> ()  [unwired: 2 in, 2 out]
        n745 = property on="Y Scan Velocity SP steps/sec" class="DigNum (strict)"("Val(Sgnl)"=w1293) -> ()  [unwired: 2 in, 2 out]
      }
      event #9 {
        n746 = event-data() -> ()  [unwired: 1 in, 7 out]
        n747 = property on="X Step SP" class="DigNum (strict)"() -> ("Maximum"=w1313:dbl)  [unwired: 2 in, 2 out]
        n748 = property on="X Step SP" class="DigNum (strict)"() -> ("Minimum"=w1314:dbl)  [unwired: 2 in, 2 out]
        n749 = property on="X steps/rev" class="DigNum (strict)"() -> ("Value"=w1319:u32)  [unwired: 2 in, 2 out]
        n750 = To Double Precision Float(number=w1319) -> (double precision float=w1305:dbl)
        n751 = property on="X Scan Length SP mm" class="DigNum (strict)"() -> ("Value"=w1317:dbl)  [unwired: 2 in, 2 out]
        n752 = property on="X mm/rev" class="DigNum (strict)"() -> ("Value"=w1304:dbl)  [unwired: 2 in, 2 out]
        n753 = property on="X Scan Velocity SP steps/sec" class="DigNum (strict)"() -> ("Maximum"=w1307:dbl)  [unwired: 2 in, 2 out]
        n754 = property on="X Scan Velocity SP steps/sec" class="DigNum (strict)"() -> ("Minimum"=w1306:dbl)  [unwired: 2 in, 2 out]
        n755 = property on="X Scan Velocity SP mm/sec" class="DigNum (strict)"() -> ("Value"=w1311:dbl)  [unwired: 2 in, 2 out]
        n756 = Divide(x=w1317, y=w1304) -> (x/y=w1320:dbl)
        n757 = Multiply(x=w1320, y=w1305) -> (x*y=w1316:dbl)
        n758 = Divide(x=w1311, y=w1304) -> (x/y=w1312:dbl)
        n759 = Multiply(x=w1312, y=w1305) -> (x*y=w1309:dbl)
        n760 = In Range and Coerce(upper limit=w1313, x=w1316, lower limit=w1314) -> (coerced(x)=w1315:dbl)  [unwired: 1 out]
        n761 = To Long Integer(number=w1315) -> (32bit integer=w1318:i32)
        n762 = In Range and Coerce(upper limit=w1307, x=w1309, lower limit=w1306) -> (coerced(x)=w1308:dbl)  [unwired: 1 out]
        n763 = To Long Integer(number=w1308) -> (32bit integer=w1310:i32)
        n764 = property on="X Scan Length SP steps" class="DigNum (strict)"("Val(Sgnl)"=w1318) -> ()  [unwired: 2 in, 2 out]
        n765 = property on="X Scan Velocity SP steps/sec" class="DigNum (strict)"("Val(Sgnl)"=w1310) -> ()  [unwired: 2 in, 2 out]
      }
      event #10 {
        n766 = event-data() -> ()  [unwired: 1 in, 7 out]
        n767 = property on="Z Step SP" class="DigNum (strict)"() -> ("Maximum"=w1330:dbl)  [unwired: 2 in, 2 out]
        n768 = property on="Z Step SP" class="DigNum (strict)"() -> ("Minimum"=w1331:dbl)  [unwired: 2 in, 2 out]
        n769 = property on="Z steps/rev" class="DigNum (strict)"() -> ("Value"=w1336:u32)  [unwired: 2 in, 2 out]
        n770 = To Double Precision Float(number=w1336) -> (double precision float=w1322:dbl)
        n771 = property on="Z Scan Length SP mm" class="DigNum (strict)"() -> ("Value"=w1334:dbl)  [unwired: 2 in, 2 out]
        n772 = property on="Z mm/rev" class="DigNum (strict)"() -> ("Value"=w1321:dbl)  [unwired: 2 in, 2 out]
        n773 = property on="Z Scan Velocity SP steps/sec" class="DigNum (strict)"() -> ("Maximum"=w1324:dbl)  [unwired: 2 in, 2 out]
        n774 = property on="Z Scan Velocity SP steps/sec" class="DigNum (strict)"() -> ("Minimum"=w1323:dbl)  [unwired: 2 in, 2 out]
        n775 = property on="Z Scan Velocity SP mm/sec" class="DigNum (strict)"() -> ("Value"=w1328:dbl)  [unwired: 2 in, 2 out]
        n776 = Divide(x=w1334, y=w1321) -> (x/y=w1337:dbl)
        n777 = Multiply(x=w1337, y=w1322) -> (x*y=w1333:dbl)
        n778 = Divide(x=w1328, y=w1321) -> (x/y=w1329:dbl)
        n779 = Multiply(x=w1329, y=w1322) -> (x*y=w1326:dbl)
        n780 = In Range and Coerce(upper limit=w1330, x=w1333, lower limit=w1331) -> (coerced(x)=w1332:dbl)  [unwired: 1 out]
        n781 = To Long Integer(number=w1332) -> (32bit integer=w1335:i32)
        n782 = In Range and Coerce(upper limit=w1324, x=w1326, lower limit=w1323) -> (coerced(x)=w1325:dbl)  [unwired: 1 out]
        n783 = To Long Integer(number=w1325) -> (32bit integer=w1327:i32)
        n784 = property on="Z Scan Length SP steps" class="DigNum (strict)"("Val(Sgnl)"=w1335) -> ()  [unwired: 2 in, 2 out]
        n785 = property on="Z Scan Velocity SP steps/sec" class="DigNum (strict)"("Val(Sgnl)"=w1327) -> ()  [unwired: 2 in, 2 out]
      }
      event #11 {
        n786 = event-data() -> ()  [unwired: 1 in, 7 out]
        n787 = property on="R Step SP" class="DigNum (strict)"() -> ("Maximum"=w1348:dbl)  [unwired: 2 in, 2 out]
        n788 = property on="R Step SP" class="DigNum (strict)"() -> ("Minimum"=w1349:dbl)  [unwired: 2 in, 2 out]
        n789 = property on="R steps/rev" class="DigNum (strict)"() -> ("Value"=w1354:u32)  [unwired: 2 in, 2 out]
        n790 = property on="R Velocity SP step/sec" class="DigNum (strict)"() -> ("Maximum"=w1342:dbl)  [unwired: 2 in, 2 out]
        n791 = To Double Precision Float(number=w1354) -> (double precision float=w1340:dbl)
        n792 = property on="R Scan Length SP deg" class="DigNum (strict)"() -> ("Value"=w1352:dbl)  [unwired: 2 in, 2 out]
        n793 = property on="R deg/rev" class="DigNum (strict)"() -> ("Value"=w1339:dbl)  [unwired: 2 in, 2 out]
        n794 = property on="R Scan Velocity SP steps/sec" class="DigNum (strict)"() -> ("Minimum"=w1341:dbl)  [unwired: 2 in, 2 out]
        n795 = property on="R Scan Velocity SP deg/sec" class="DigNum (strict)"() -> ("Value"=w1346:dbl)  [unwired: 2 in, 2 out]
        n796 = Divide(x=w1352, y=w1339) -> (x/y=w1355:dbl)
        n797 = Multiply(x=w1355, y=w1340) -> (x*y=w1351:dbl)
        n798 = Divide(x=w1346, y=w1339) -> (x/y=w1347:dbl)
        n799 = Multiply(x=w1347, y=w1340) -> (x*y=w1344:dbl)
        n800 = In Range and Coerce(upper limit=w1348, x=w1351, lower limit=w1349) -> (coerced(x)=w1350:dbl)  [unwired: 1 out]
        n801 = To Long Integer(number=w1350) -> (32bit integer=w1353:i32)
        n802 = Absolute Value(x=w1344) -> (abs(x)=w1338:dbl)
        n803 = property on="R Scan Length SP steps" class="DigNum (strict)"("Val(Sgnl)"=w1353) -> ()  [unwired: 2 in, 2 out]
        n804 = In Range and Coerce(upper limit=w1342, x=w1338, lower limit=w1341) -> (coerced(x)=w1343:dbl)  [unwired: 1 out]
        n805 = To Long Integer(number=w1343) -> (32bit integer=w1345:i32)
        n806 = property on="R Scan Velocity SP steps/sec" class="DigNum (strict)"("Val(Sgnl)"=w1345) -> ()  [unwired: 2 in, 2 out]
      }
      event #12 {
        n807 = event-data() -> ()  [unwired: 1 in, 7 out]
        n808 = flat-sequence {
          tunnel: w1360 -> [w1370]
          tunnel: w1361 -> [w1371]
          tunnel: [w1371] -> w1357
          tunnel: [w1370] -> w1356
          tunnel: [w1374] -> w1359
          tunnel: [w1373] -> w1358
          tunnel: w1357 -> [w1376]
          tunnel: w1356 -> [w1375]
          tunnel: [w1394] -> w1363
          tunnel: [w1393] -> w1362
          tunnel: w1359 -> [w1392]
          tunnel: w1358 -> [w1391]
          tunnel: [w1401] -> w1365
          tunnel: [w1400] -> w1364
          tunnel: w1363 -> [w1399]
          tunnel: w1362 -> [w1398]
          tunnel: [w1407] -> w1366
          tunnel: [w1408] -> w1367
          tunnel: w1365 -> [w1408]
          tunnel: w1364 -> [w1406]
          frame #0 {
            n809 = property on="Scan Go" class="Bool"("DisabledEnum"=T2."Disabled and Grayed Out" ("Disabled")) -> ()  [unwired: 2 in, 2 out]
            n810 = property on="Y Go" class="Bool"("DisabledEnum"=T2."Disabled and Grayed Out" ("Disabled")) -> ()  [unwired: 2 in, 2 out]
          }
          frame #1 {
            n811 = property on="Y Step SP" class="DigNum (strict)"() -> ("Value"=w1384:i32)  [unwired: 2 in, 2 out]
            n812 = property on="Y Step PV" class="DigNum (strict)"() -> ("Value"=w1383:i32)  [unwired: 2 in, 2 out]
            n813 = property on="Y Backlash" class="DigNum (strict)"() -> ("Value"=w1372:i32)  [unwired: 2 in, 2 out]
            n814 = Subtract(x=w1384, y=w1383) -> (x-y=w1382:i32)
            n815 = Sign(1:w1372) -> (0:w1380:i32)
            n816 = Sign(1:w1382) -> (0:w1381:i32)
            n817 = Multiply(x=w1381, y=w1380) -> (x*y=w1379:i32)
            n818 = Equal?(x=w1379, y=1) -> (x = y?=w1377:bool)
            n819 = case shown="False" w1377 {
              tunnel: w1376 -> [w1387 w1389]
              tunnel: w1375 -> [w1386 w1388]
              tunnel: [w1386 w1388] -> w1374
              tunnel: [w1387 w1389] -> w1373
              frame #0 {
                n820 = property on="Y Backlash corr" class="Bool (strict)"("Val(Sgnl)"=FALSE ("Value (Signaling)")) -> ()  [unwired: 2 in, 2 out]
              }
              frame #1 {
                n821 = property on="Y Backlash corr" class="Bool (strict)"("Val(Sgnl)"=TRUE ("Value (Signaling)")) -> ()  [unwired: 2 in, 2 out]
              }
            }
          }
          frame #2 {
            # "Velocity Setting"
            n822 = property on="Y Velocity SP step/sec" class="DigNum (strict)"() -> ("Value"=w1395:i32)  [unwired: 2 in, 2 out]
            n823 = Number To Decimal String(number=w1395) -> (decimal integer string=w1396:string)  [unwired: 1 in]
            n824 = call "mDrive Send Command.vi"("error in (no error)"=w1392, "Extra"=w1396, "Command"=T1."Max Velocity", "VISA resource name"=w1391) -> ("error out"=w1393:errorcluster, "VISA resource name out"=w1394:refnum<visa-resource-name>)  [unwired: 3 in, 1 out]
          }
          frame #3 {
            # "Move to Abs Position"
            n825 = property on="Y Step SP" class="DigNum (strict)"() -> ("Value"=w1404:i32)  [unwired: 2 in, 2 out]
            n826 = Number To Decimal String(number=w1404) -> (decimal integer string=w1403:string)  [unwired: 1 in]
            n827 = call "mDrive Send Command.vi"("error in (no error)"=w1398, "Extra"=w1403, "Command"=T1."Move to Absolute Position", "VISA resource name"=w1399) -> ("error out"=w1400:errorcluster, "VISA resource name out"=w1401:refnum<visa-resource-name>)  [unwired: 3 in, 1 out]
          }
          frame #4 {
            n828 = call "Time Delay"("error in (no error)"=w1406, "Delay Time (s)"=0.1) -> ("error out"=w1407:errorcluster)  [unwired: 9 in]
          }
        }
      }
      event #13 {
        n829 = event-data() -> ()  [unwired: 1 in, 7 out]
        n830 = flat-sequence {
          tunnel: w1411 -> [w1423]
          tunnel: w1412 -> [w1424]
          tunnel: [w1424] -> w1414
          tunnel: [w1423] -> w1413
          tunnel: [w1427] -> w1416
          tunnel: [w1426] -> w1415
          tunnel: w1414 -> [w1429]
          tunnel: w1413 -> [w1428]
          tunnel: [w1447] -> w1418
          tunnel: [w1446] -> w1417
          tunnel: w1416 -> [w1445]
          tunnel: w1415 -> [w1444]
          tunnel: [w1454] -> w1420
          tunnel: [w1453] -> w1419
          tunnel: w1418 -> [w1452]
          tunnel: w1417 -> [w1451]
          tunnel: [w1460] -> w1410
          tunnel: [w1461] -> w1409
          tunnel: w1420 -> [w1461]
          tunnel: w1419 -> [w1459]
          frame #0 {
            n831 = property on="Scan Go" class="Bool"("DisabledEnum"=T2."Disabled and Grayed Out" ("Disabled")) -> ()  [unwired: 2 in, 2 out]
            n832 = property on="Z Go" class="Bool"("DisabledEnum"=T2."Disabled and Grayed Out" ("Disabled")) -> ()  [unwired: 2 in, 2 out]
          }
          frame #1 {
            n833 = property on="Z Step SP" class="DigNum (strict)"() -> ("Value"=w1437:i32)  [unwired: 2 in, 2 out]
            n834 = property on="Z Step PV" class="DigNum (strict)"() -> ("Value"=w1436:i32)  [unwired: 2 in, 2 out]
            n835 = property on="Z Backlash" class="DigNum (strict)"() -> ("Value"=w1425:i32)  [unwired: 2 in, 2 out]
            n836 = Subtract(x=w1437, y=w1436) -> (x-y=w1435:i32)
            n837 = Sign(1:w1425) -> (0:w1433:i32)
            n838 = Sign(1:w1435) -> (0:w1434:i32)
            n839 = Multiply(x=w1434, y=w1433) -> (x*y=w1432:i32)
            n840 = Equal?(x=w1432, y=1) -> (x = y?=w1430:bool)
            n841 = case shown="True" w1430 {
              tunnel: w1429 -> [w1440 w1442]
              tunnel: w1428 -> [w1439 w1441]
              tunnel: [w1439 w1441] -> w1427
              tunnel: [w1440 w1442] -> w1426
              frame #0 {
                n842 = property on="Z Backlash corr" class="Bool (strict)"("Val(Sgnl)"=FALSE ("Value (Signaling)")) -> ()  [unwired: 2 in, 2 out]
              }
              frame #1 {
                n843 = property on="Z Backlash corr" class="Bool (strict)"("Val(Sgnl)"=TRUE ("Value (Signaling)")) -> ()  [unwired: 2 in, 2 out]
              }
            }
          }
          frame #2 {
            # "Velocity Setting"
            n844 = property on="Z Velocity SP step/sec" class="DigNum (strict)"() -> ("Value"=w1448:i32)  [unwired: 2 in, 2 out]
            n845 = Number To Decimal String(number=w1448) -> (decimal integer string=w1449:string)  [unwired: 1 in]
            n846 = call "mDrive Send Command.vi"("error in (no error)"=w1445, "Extra"=w1449, "Command"=T1."Max Velocity", "VISA resource name"=w1444) -> ("error out"=w1446:errorcluster, "VISA resource name out"=w1447:refnum<visa-resource-name>)  [unwired: 3 in, 1 out]
          }
          frame #3 {
            # "Move to Abs Position"
            n847 = property on="Z Step SP" class="DigNum (strict)"() -> ("Value"=w1457:i32)  [unwired: 2 in, 2 out]
            n848 = Number To Decimal String(number=w1457) -> (decimal integer string=w1456:string)  [unwired: 1 in]
            n849 = call "mDrive Send Command.vi"("error in (no error)"=w1451, "Extra"=w1456, "Command"=T1."Move to Absolute Position", "VISA resource name"=w1452) -> ("error out"=w1453:errorcluster, "VISA resource name out"=w1454:refnum<visa-resource-name>)  [unwired: 3 in, 1 out]
          }
          frame #4 {
            n850 = call "Time Delay28"("error in (no error)"=w1459, "Delay Time (s)"=0.1) -> ("error out"=w1460:errorcluster)  [unwired: 9 in]
          }
        }
      }
      event #14 {
        n851 = event-data() -> ()  [unwired: 1 in, 7 out]
        n852 = flat-sequence {
          tunnel: w1464 -> [w1476]
          tunnel: w1465 -> [w1477]
          tunnel: [w1477] -> w1467
          tunnel: [w1476] -> w1466
          tunnel: [w1480] -> w1469
          tunnel: [w1479] -> w1468
          tunnel: w1467 -> [w1482]
          tunnel: w1466 -> [w1481]
          tunnel: [w1500] -> w1471
          tunnel: [w1499] -> w1470
          tunnel: w1469 -> [w1498]
          tunnel: w1468 -> [w1497]
          tunnel: [w1507] -> w1473
          tunnel: [w1506] -> w1472
          tunnel: w1471 -> [w1505]
          tunnel: w1470 -> [w1504]
          tunnel: [w1513] -> w1463
          tunnel: [w1514] -> w1462
          tunnel: w1473 -> [w1514]
          tunnel: w1472 -> [w1512]
          frame #0 {
            n853 = property on="Scan Go" class="Bool"("DisabledEnum"=T2."Disabled and Grayed Out" ("Disabled")) -> ()  [unwired: 2 in, 2 out]
            n854 = property on="R Go" class="Bool"("DisabledEnum"=T2."Disabled and Grayed Out" ("Disabled")) -> ()  [unwired: 2 in, 2 out]
          }
          frame #1 {
            n855 = property on="R Step SP" class="DigNum (strict)"() -> ("Value"=w1490:i32)  [unwired: 2 in, 2 out]
            n856 = property on="R Step PV" class="DigNum (strict)"() -> ("Value"=w1489:i32)  [unwired: 2 in, 2 out]
            n857 = property on="R Backlash" class="DigNum (strict)"() -> ("Value"=w1478:i32)  [unwired: 2 in, 2 out]
            n858 = Subtract(x=w1490, y=w1489) -> (x-y=w1488:i32)
            n859 = Sign(1:w1478) -> (0:w1486:i32)
            n860 = Sign(1:w1488) -> (0:w1487:i32)
            n861 = Multiply(x=w1487, y=w1486) -> (x*y=w1485:i32)
            n862 = Equal?(x=w1485, y=1) -> (x = y?=w1483:bool)
            n863 = case shown="True" w1483 {
              tunnel: w1482 -> [w1493 w1495]
              tunnel: w1481 -> [w1492 w1494]
              tunnel: [w1492 w1494] -> w1480
              tunnel: [w1493 w1495] -> w1479
              frame #0 {
                n864 = property on="R Backlash corr" class="Bool (strict)"("Val(Sgnl)"=FALSE ("Value (Signaling)")) -> ()  [unwired: 2 in, 2 out]
              }
              frame #1 {
                n865 = property on="R Backlash corr" class="Bool (strict)"("Val(Sgnl)"=TRUE ("Value (Signaling)")) -> ()  [unwired: 2 in, 2 out]
              }
            }
          }
          frame #2 {
            # "Velocity Setting"
            n866 = property on="R Velocity SP step/sec" class="DigNum (strict)"() -> ("Value"=w1501:i32)  [unwired: 2 in, 2 out]
            n867 = Number To Decimal String(number=w1501) -> (decimal integer string=w1502:string)  [unwired: 1 in]
            n868 = call "mDrive Send Command.vi"("error in (no error)"=w1498, "Extra"=w1502, "Command"=T1."Max Velocity", "VISA resource name"=w1497) -> ("error out"=w1499:errorcluster, "VISA resource name out"=w1500:refnum<visa-resource-name>)  [unwired: 3 in, 1 out]
          }
          frame #3 {
            # "Move to Abs Position"
            n869 = property on="R Step SP" class="DigNum (strict)"() -> ("Value"=w1510:i32)  [unwired: 2 in, 2 out]
            n870 = Number To Decimal String(number=w1510) -> (decimal integer string=w1509:string)  [unwired: 1 in]
            n871 = call "mDrive Send Command.vi"("error in (no error)"=w1504, "Extra"=w1509, "Command"=T1."Move to Absolute Position", "VISA resource name"=w1505) -> ("error out"=w1506:errorcluster, "VISA resource name out"=w1507:refnum<visa-resource-name>)  [unwired: 3 in, 1 out]
          }
          frame #4 {
            n872 = call "Time Delay29"("error in (no error)"=w1512, "Delay Time (s)"=0.1) -> ("error out"=w1513:errorcluster)  [unwired: 9 in]
          }
        }
      }
      event #15 {
        n873 = event-data() -> ()  [unwired: 1 in, 7 out]
        n874 = flat-sequence {
          tunnel: [w1530] -> w1526
          tunnel: [w1529] -> w1525
          tunnel: w1524 -> [w1530]
          tunnel: w1523 -> [w1529]
          tunnel: [w1535] -> w1528
          tunnel: [w1534] -> w1527
          tunnel: w1526 -> [w1537]
          tunnel: w1525 -> [w1536]
          tunnel: [w1556] -> w1520
          tunnel: [w1553] -> w1518
          tunnel: w1528 -> [w1557]
          tunnel: w1527 -> [w1558]
          tunnel: [w1552] -> w1516
          tunnel: w1520 -> [w1565]
          tunnel: [w1564] -> w1519
          tunnel: w1518 -> [w1566]
          tunnel: [w1567] -> w1517
          tunnel: w1516 -> [w1563]
          tunnel: [w1563] -> w1515
          tunnel: w1519 -> [w1577]
          tunnel: w1517 -> [w1576]
          tunnel: [w1575] -> w1522
          tunnel: [w1574] -> w1521
          tunnel: w1515 -> [w1572]
          frame #0 {
            n875 = property on="Scan Go" class="Bool"("DisabledEnum"=T2."Disabled and Grayed Out" ("Disabled")) -> ()  [unwired: 2 in, 2 out]
            n876 = property on="X Go" class="Bool"("DisabledEnum"=T2."Disabled and Grayed Out" ("Disabled")) -> ()  [unwired: 2 in, 2 out]
          }
          frame #1 {
            n877 = property on="X Step SP" class="DigNum (strict)"() -> ("Value"=w1545:i32)  [unwired: 2 in, 2 out]
            n878 = property on="X Step PV" class="DigNum (strict)"() -> ("Value"=w1544:i32)  [unwired: 2 in, 2 out]
            n879 = Subtract(x=w1545, y=w1544) -> (x-y=w1543:i32)
            n880 = property on="X Backlash" class="DigNum (strict)"() -> ("Value"=w1533:i32)  [unwired: 2 in, 2 out]
            n881 = Sign(1:w1543) -> (0:w1542:i32)
            n882 = Sign(1:w1533) -> (0:w1541:i32)
            n883 = Multiply(x=w1542, y=w1541) -> (x*y=w1540:i32)
            n884 = Equal?(x=w1540, y=1) -> (x = y?=w1538:bool)
            n885 = case shown="True" w1538 {
              tunnel: w1537 -> [w1548 w1550]
              tunnel: w1536 -> [w1547 w1549]
              tunnel: [w1547 w1549] -> w1535
              tunnel: [w1548 w1550] -> w1534
              frame #0 {
                n886 = property on="X Backlash corr" class="Bool (strict)"("Val(Sgnl)"=FALSE ("Value (Signaling)")) -> ()  [unwired: 2 in, 2 out]
              }
              frame #1 {
                n887 = property on="X Backlash corr" class="Bool (strict)"("Val(Sgnl)"=TRUE ("Value (Signaling)")) -> ()  [unwired: 2 in, 2 out]
              }
            }
          }
          frame #2 {
            w1552 = 0.1 ("Delay Time (s)")
            n888 = property on="X Velocity SP step/sec" class="DigNum (strict)"() -> ("Value"=w1555:i32)  [unwired: 2 in, 2 out]
            n889 = property on="X steps/rev" class="DigNum (strict)"() -> ("Value"=w1559:u32)  [unwired: 2 in, 2 out]
            n890 = Divide(x=w1555, y=w1559) -> (x/y=w1560:dbl)
            n891 = Number To Fractional String(number=w1560) -> (F-format string=w1561:string)  [unwired: 3 in]
            n892 = call "Applied Send Command.vi"("error in (no error)"=w1557, "Extra"=w1561, "Command"=T3."Velocity Setting", "VISA resource name"=w1558) -> ("error out"=w1554:errorcluster, "VISA resource name out"=w1556:refnum<visa-resource-name>)  [unwired: 3 in, 1 out]
            n893 = call "Time Delay14"("error in (no error)"=w1554, "Delay Time (s)"=w1552) -> ("error out"=w1553:errorcluster)  [unwired: 9 in]
          }
          frame #3 {
            # "Distance/Position"
            n894 = property on="X Step SP" class="DigNum (strict)"() -> ("Value"=w1568:i32)  [unwired: 2 in, 2 out]
            n895 = Number To Decimal String(number=w1568) -> (decimal integer string=w1570:string)  [unwired: 1 in]
            n896 = call "Applied Send Command.vi"("error in (no error)"=w1566, "Extra"=w1570, "Command"=T3."Distance or Position", "VISA resource name"=w1565) -> ("error out"=w1569:errorcluster, "VISA resource name out"=w1564:refnum<visa-resource-name>)  [unwired: 3 in, 1 out]
            n897 = call "Time Delay31"("error in (no error)"=w1569, "Delay Time (s)"=w1563) -> ("error out"=w1567:errorcluster)  [unwired: 9 in]
          }
          frame #4 {
            # "Feed to Position"
            n898 = call "Applied Send Command.vi"("error in (no error)"=w1576, "Command"=T3."Feed to Position", "VISA resource name"=w1577) -> ("error out"=w1573:errorcluster, "VISA resource name out"=w1575:refnum<visa-resource-name>)  [unwired: 4 in, 1 out]
            n899 = call "Time Delay15"("error in (no error)"=w1573, "Delay Time (s)"=w1572) -> ("error out"=w1574:errorcluster)  [unwired: 9 in]
          }
        }
      }
      event #16 {
        n900 = event-data() -> ()  [unwired: 1 in, 7 out]
        n901 = flat-sequence {
          tunnel: [w1591] -> w1586
          tunnel: [w1603] -> w1585
          tunnel: w1584 -> [w1600]
          tunnel: w1583 -> [w1599]
          tunnel: w1586 -> [w1611]
          tunnel: w1585 -> [w1610]
          tunnel: [w1611] -> w1580
          tunnel: [w1610] -> w1579
          tunnel: [w1613] -> w1581
          tunnel: [w1614] -> w1582
          tunnel: w1580 -> [w1614]
          tunnel: w1579 -> [w1613]
          frame #0 {
            # "VELOCITY"
            n902 = property on="X Scan Velocity SP steps/sec" class="DigNum (strict)"() -> ("Value"=w1604:i32)  [unwired: 2 in, 2 out]
            n903 = Number To Decimal String(number=w1604) -> (decimal integer string=w1601:string)  [unwired: 1 in]
            n904 = call "Applied Send Command.vi"("error in (no error)"=w1599, "Extra"=w1601, "Command"=T3."Velocity Setting", "VISA resource name"=w1600) -> ("error out"=w1587:errorcluster, "VISA resource name out"=w1588:refnum<visa-resource-name>)  [unwired: 3 in, 1 out]
            n905 = call "Time Delay9"("error in (no error)"=w1587) -> ("error out"=w1589:errorcluster)  [unwired: 10 in]
            n906 = call "Applied Send Command.vi"("error in (no error)"=w1589, "Extra"="", "Command"=T3."Velocity Setting", "VISA resource name"=w1588) -> ("error out"=w1590:errorcluster, "read buffer"=w1596:string, "VISA resource name out"=w1591:refnum<visa-resource-name>)  [unwired: 3 in]
            n907 = Fract/Exp String To Number(string=w1596, offset=3) -> (number=w1594:dbl)  [unwired: 2 in, 1 out]
            n908 = property on="X steps/rev" class="DigNum (strict)"() -> ("Value"=w1593:u32)  [unwired: 2 in, 2 out]
            n909 = Multiply(x=w1594, y=w1593) -> (x*y=w1592:dbl)
            n910 = call "Time Delay10"("error in (no error)"=w1590) -> ("error out"=w1603:errorcluster)  [unwired: 10 in]
            n911 = property on="X velocity PV step/sec" class="DigNum (strict)"("Val(Sgnl)"=w1592) -> ()  [unwired: 2 in, 2 out]
          }
          frame #1 {
            n912 = property on="X Scan" class="Bool (strict)"("Val(Sgnl)"=TRUE ("Slew Ready 2")) -> ()  [unwired: 2 in, 2 out]
            n913 = property on="Scan Cancel" class="Bool"("DisabledEnum"=T2."Enabled" ("Disabled")) -> ()  [unwired: 2 in, 2 out]
            n914 = property on="Scan Go" class="Bool"("DisabledEnum"=T2."Enabled" ("Disabled")) -> ()  [unwired: 2 in, 2 out]
            n915 = property on="X Scan Length SP steps" class="DigNum (strict)"("DisabledEnum"=T2."Disabled and Grayed Out" ("Disabled")) -> ()  [unwired: 2 in, 2 out]
            n916 = property on="X Scan Velocity SP steps/sec" class="DigNum (strict)"("DisabledEnum"=T2."Disabled and Grayed Out" ("Disabled")) -> ()  [unwired: 2 in, 2 out]
          }
          frame #2 {
            n917 = property on="X Go" class="Bool"("DisabledEnum"=T2."Disabled and Grayed Out" ("Disabled")) -> ()  [unwired: 2 in, 2 out]
          }
        }
      }
      event #17 {
        n918 = event-data() -> ()  [unwired: 1 in, 7 out]
        n919 = flat-sequence {
          tunnel: w1622 -> [w1632]
          tunnel: w1621 -> [w1631]
          tunnel: [w1628] -> w1619
          tunnel: [w1626] -> w1618
          tunnel: w1619 -> [w1645]
          tunnel: w1618 -> [w1644]
          tunnel: [w1645] -> w1616
          tunnel: [w1644] -> w1615
          tunnel: [w1647] -> w1620
          tunnel: [w1648] -> w1617
          tunnel: w1616 -> [w1648]
          tunnel: w1615 -> [w1647]
          frame #0 {
            # "VELOCITY"
            n920 = property on="Y Scan Velocity SP steps/sec" class="DigNum (strict)"() -> ("Value"=w1629:i32)  [unwired: 2 in, 2 out]
            n921 = Number To Decimal String(number=w1629) -> (decimal integer string=w1630:string)  [unwired: 1 in]
            n922 = call "mDrive Send Command.vi"("error in (no error)"=w1632, "Extra"=w1630, "Command"=T1."Max Velocity", "VISA resource name"=w1631) -> ("error out"=w1633:errorcluster, "VISA resource name out"=w1638:refnum<visa-resource-name>)  [unwired: 3 in, 1 out]
            n923 = call "Time Delay5"("error in (no error)"=w1633) -> ("error out"=w1636:errorcluster)  [unwired: 10 in]
            n924 = call "mDrive Send Command.vi"("error in (no error)"=w1636, "Extra"="VM", "Command"=T1."Print Parameter", "VISA resource name"=w1638) -> ("error out"=w1627:errorcluster, "read buffer"=w1634:string, "VISA resource name out"=w1628:refnum<visa-resource-name>)  [unwired: 3 in]
            n925 = Decimal String To Number(string=w1634, offset=0) -> (number=w1637:i32)  [unwired: 1 in, 1 out]
            n926 = property on="Y velocity PV step/sec" class="DigNum (strict)"("Val(Sgnl)"=w1637) -> ()  [unwired: 2 in, 2 out]
            n927 = call "Time Delay6"("error in (no error)"=w1627) -> ("error out"=w1626:errorcluster)  [unwired: 10 in]
          }
          frame #1 {
            n928 = property on="Y Scan" class="Bool (strict)"("Val(Sgnl)"=TRUE ("Slew Ready 2")) -> ()  [unwired: 2 in, 2 out]
            n929 = property on="Scan Cancel" class="Bool"("DisabledEnum"=T2."Enabled" ("Disabled")) -> ()  [unwired: 2 in, 2 out]
            n930 = property on="Scan Go" class="Bool"("DisabledEnum"=T2."Enabled" ("Disabled")) -> ()  [unwired: 2 in, 2 out]
            n931 = property on="Y Scan Length SP steps" class="DigNum (strict)"("DisabledEnum"=T2."Disabled and Grayed Out" ("Disabled")) -> ()  [unwired: 2 in, 2 out]
            n932 = property on="Y Scan Velocity SP steps/sec" class="DigNum (strict)"("DisabledEnum"=T2."Disabled and Grayed Out" ("Disabled")) -> ()  [unwired: 2 in, 2 out]
          }
          frame #2 {
            n933 = property on="Y Go" class="Bool"("DisabledEnum"=T2."Disabled and Grayed Out" ("Disabled")) -> ()  [unwired: 2 in, 2 out]
          }
        }
      }
      event #18 {
        n934 = event-data() -> ()  [unwired: 1 in, 7 out]
        n935 = flat-sequence {
          tunnel: [w1664] -> w1656
          tunnel: [w1662] -> w1655
          tunnel: w1652 -> [w1658]
          tunnel: w1651 -> [w1657]
          tunnel: w1656 -> [w1679]
          tunnel: w1655 -> [w1678]
          tunnel: [w1679] -> w1654
          tunnel: [w1678] -> w1653
          tunnel: [w1681] -> w1650
          tunnel: [w1682] -> w1649
          tunnel: w1654 -> [w1682]
          tunnel: w1653 -> [w1681]
          frame #0 {
            # "VELOCITY"
            n936 = property on="Z Scan Velocity SP steps/sec" class="DigNum (strict)"() -> ("Value"=w1665:i32)  [unwired: 2 in, 2 out]
            n937 = Number To Decimal String(number=w1665) -> (decimal integer string=w1666:string)  [unwired: 1 in]
            n938 = call "mDrive Send Command.vi"("error in (no error)"=w1657, "Extra"=w1666, "Command"=T1."Max Velocity", "VISA resource name"=w1658) -> ("error out"=w1667:errorcluster, "VISA resource name out"=w1672:refnum<visa-resource-name>)  [unwired: 3 in, 1 out]
            n939 = call "Time Delay24"("error in (no error)"=w1667) -> ("error out"=w1670:errorcluster)  [unwired: 10 in]
            n940 = call "mDrive Send Command.vi"("error in (no error)"=w1670, "Extra"="VM", "Command"=T1."Print Parameter", "VISA resource name"=w1672) -> ("error out"=w1663:errorcluster, "read buffer"=w1668:string, "VISA resource name out"=w1664:refnum<visa-resource-name>)  [unwired: 3 in]
            n941 = Decimal String To Number(string=w1668, offset=0) -> (number=w1671:i32)  [unwired: 1 in, 1 out]
            n942 = property on="Z  velocity PV step/sec" class="DigNum (strict)"("Val(Sgnl)"=w1671) -> ()  [unwired: 2 in, 2 out]
            n943 = call "Time Delay25"("error in (no error)"=w1663) -> ("error out"=w1662:errorcluster)  [unwired: 10 in]
          }
          frame #1 {
            n944 = property on="Z Scan" class="Bool (strict)"("Val(Sgnl)"=TRUE ("Slew Ready 2")) -> ()  [unwired: 2 in, 2 out]
            n945 = property on="Scan Cancel" class="Bool"("DisabledEnum"=T2."Enabled" ("Disabled")) -> ()  [unwired: 2 in, 2 out]
            n946 = property on="Scan Go" class="Bool"("DisabledEnum"=T2."Enabled" ("Disabled")) -> ()  [unwired: 2 in, 2 out]
            n947 = property on="Z Scan Length SP steps" class="DigNum (strict)"("DisabledEnum"=T2."Disabled and Grayed Out" ("Disabled")) -> ()  [unwired: 2 in, 2 out]
            n948 = property on="Z Scan Velocity SP steps/sec" class="DigNum (strict)"("DisabledEnum"=T2."Disabled and Grayed Out" ("Disabled")) -> ()  [unwired: 2 in, 2 out]
          }
          frame #2 {
            n949 = property on="Z Go" class="Bool"("DisabledEnum"=T2."Disabled and Grayed Out" ("Disabled")) -> ()  [unwired: 2 in, 2 out]
          }
        }
      }
      event #19 {
        n950 = event-data() -> ()  [unwired: 1 in, 7 out]
        n951 = flat-sequence {
          tunnel: [w1698] -> w1690
          tunnel: [w1696] -> w1689
          tunnel: w1686 -> [w1692]
          tunnel: w1685 -> [w1691]
          tunnel: w1690 -> [w1713]
          tunnel: w1689 -> [w1712]
          tunnel: [w1713] -> w1688
          tunnel: [w1712] -> w1687
          tunnel: [w1715] -> w1683
          tunnel: [w1716] -> w1684
          tunnel: w1688 -> [w1716]
          tunnel: w1687 -> [w1715]
          frame #0 {
            # "VELOCITY"
            n952 = property on="R Scan Velocity SP steps/sec" class="DigNum (strict)"() -> ("Value"=w1699:i32)  [unwired: 2 in, 2 out]
            n953 = Number To Decimal String(number=w1699) -> (decimal integer string=w1700:string)  [unwired: 1 in]
            n954 = call "mDrive Send Command.vi"("error in (no error)"=w1691, "Extra"=w1700, "Command"=T1."Max Velocity", "VISA resource name"=w1692) -> ("error out"=w1701:errorcluster, "VISA resource name out"=w1706:refnum<visa-resource-name>)  [unwired: 3 in, 1 out]
            n955 = call "Time Delay26"("error in (no error)"=w1701) -> ("error out"=w1704:errorcluster)  [unwired: 10 in]
            n956 = call "mDrive Send Command.vi"("error in (no error)"=w1704, "Extra"="VM", "Command"=T1."Print Parameter", "VISA resource name"=w1706) -> ("error out"=w1697:errorcluster, "read buffer"=w1702:string, "VISA resource name out"=w1698:refnum<visa-resource-name>)  [unwired: 3 in]
            n957 = Decimal String To Number(string=w1702, offset=0) -> (number=w1705:i32)  [unwired: 1 in, 1 out]
            n958 = property on="R velocity PV step/sec" class="DigNum (strict)"("Val(Sgnl)"=w1705) -> ()  [unwired: 2 in, 2 out]
            n959 = call "Time Delay27"("error in (no error)"=w1697) -> ("error out"=w1696:errorcluster)  [unwired: 10 in]
          }
          frame #1 {
            n960 = property on="R Scan" class="Bool (strict)"("Val(Sgnl)"=TRUE ("Slew Ready 2")) -> ()  [unwired: 2 in, 2 out]
            n961 = property on="Scan Cancel" class="Bool"("DisabledEnum"=T2."Enabled" ("Disabled")) -> ()  [unwired: 2 in, 2 out]
            n962 = property on="Scan Go" class="Bool"("DisabledEnum"=T2."Enabled" ("Disabled")) -> ()  [unwired: 2 in, 2 out]
            n963 = property on="R Scan Length SP steps" class="DigNum (strict)"("DisabledEnum"=T2."Disabled and Grayed Out" ("Disabled")) -> ()  [unwired: 2 in, 2 out]
            n964 = property on="R Scan Velocity SP steps/sec" class="DigNum (strict)"("DisabledEnum"=T2."Disabled and Grayed Out" ("Disabled")) -> ()  [unwired: 2 in, 2 out]
          }
          frame #2 {
            n965 = property on="R Go" class="Bool"("DisabledEnum"=T2."Disabled and Grayed Out" ("Disabled")) -> ()  [unwired: 2 in, 2 out]
          }
        }
      }
      event #20 {
        n966 = event-data() -> ()  [unwired: 1 in, 4 out]
        n967 = event-data() -> ()  [unwired: 3 in, 1 out]
      }
      event #21 {
        n968 = event-data() -> ()  [unwired: 1 in, 7 out]
        n969 = flat-sequence {
          tunnel: [w1747] -> w1730
          tunnel: [w1746] -> w1729
          tunnel: w1728 -> [w1748]
          tunnel: w1727 -> [w1745]
          frame #0 {
            n970 = call "Applied Send Command.vi"("error in (no error)"=w1745, "Command"=T3."Stop", "VISA resource name"=w1748) -> ("error out"=w1746:errorcluster, "VISA resource name out"=w1747:refnum<visa-resource-name>)  [unwired: 4 in, 1 out]
          }
        }
        n971 = flat-sequence {
          tunnel: w1734 -> [w1754]
          tunnel: w1733 -> [w1753]
          tunnel: [w1752] -> w1732
          tunnel: [w1751] -> w1731
          frame #0 {
            n972 = call "mDrive Send Command.vi"("error in (no error)"=w1753, "Command"=T1."Stop", "VISA resource name"=w1754) -> ("error out"=w1751:errorcluster, "VISA resource name out"=w1752:refnum<visa-resource-name>)  [unwired: 4 in, 1 out]
          }
        }
        n973 = flat-sequence {
          tunnel: [w1743] -> w1724
          tunnel: [w1742] -> w1723
          tunnel: w1726 -> [w1741]
          tunnel: w1725 -> [w1740]
          frame #0 {
            n974 = call "mDrive Send Command.vi"("error in (no error)"=w1740, "Command"=T1."Stop", "VISA resource name"=w1741) -> ("error out"=w1742:errorcluster, "VISA resource name out"=w1743:refnum<visa-resource-name>)  [unwired: 4 in, 1 out]
          }
        }
        n975 = flat-sequence {
          tunnel: w1722 -> [w1739]
          tunnel: w1721 -> [w1738]
          tunnel: [w1737] -> w1720
          tunnel: [w1735] -> _
          tunnel: [w1735] -> w1719
          frame #0 {
            n976 = call "mDrive Send Command.vi"("error in (no error)"=w1738, "Command"=T1."Stop", "VISA resource name"=w1739) -> ("error out"=w1735:errorcluster, "VISA resource name out"=w1737:refnum<visa-resource-name>)  [unwired: 4 in, 1 out]
          }
        }
      }
      event #22 {
        n977 = event-data() -> ()  [unwired: 1 in, 7 out]
        n978 = flat-sequence {
          tunnel: w1770 -> [w1809]
          tunnel: w1769 -> [w1808]
          tunnel: [w1811] -> w1772
          tunnel: [w1810] -> w1771
          tunnel: [w1818] -> w1767
          tunnel: [w1819] -> w1768
          tunnel: w1772 -> [w1819]
          tunnel: w1771 -> [w1818]
          frame #0 {
            n979 = call "mDrive Send Command.vi"("error in (no error)"=w1808, "Command"=T1."Stop", "VISA resource name"=w1809) -> ("error out"=w1810:errorcluster, "VISA resource name out"=w1811:refnum<visa-resource-name>)  [unwired: 4 in, 1 out]
          }
          frame #1 {
            n980 = property on="X Scan" class="Bool (strict)"("Value"=FALSE ("Slew Ready")) -> ()  [unwired: 2 in, 2 out]
            n981 = property on="X Scan set" class="Bool"("DisabledEnum"=T2."Enabled" ("Disabled")) -> ()  [unwired: 2 in, 2 out]
            n982 = property on="X Scan Velocity SP steps/sec" class="DigNum (strict)"("DisabledEnum"=T2."Enabled" ("Disabled")) -> ()  [unwired: 2 in, 2 out]
            n983 = property on="X Scan Length SP steps" class="DigNum (strict)"("DisabledEnum"=T2."Enabled" ("Disabled")) -> ()  [unwired: 2 in, 2 out]
            n984 = property on="X Go" class="Bool"("DisabledEnum"=T2."Enabled" ("Disabled")) -> ()  [unwired: 2 in, 2 out]
            n985 = property on="X Scan OK" class="Bool"("DisabledEnum"=T2."Enabled" ("Disabled")) -> ()  [unwired: 2 in, 2 out]
          }
        }
        n986 = flat-sequence {
          tunnel: w1778 -> [w1822]
          tunnel: w1777 -> [w1821]
          tunnel: [w1824] -> w1774
          tunnel: [w1823] -> w1773
          tunnel: [w1831] -> w1779
          tunnel: [w1832] -> w1780
          tunnel: w1774 -> [w1832]
          tunnel: w1773 -> [w1831]
          frame #0 {
            n987 = call "mDrive Send Command.vi"("error in (no error)"=w1821, "Command"=T1."Stop", "VISA resource name"=w1822) -> ("error out"=w1823:errorcluster, "VISA resource name out"=w1824:refnum<visa-resource-name>)  [unwired: 4 in, 1 out]
          }
          frame #1 {
            n988 = property on="Y Scan" class="Bool (strict)"("Value"=FALSE ("Slew Ready")) -> ()  [unwired: 2 in, 2 out]
            n989 = property on="Y Go" class="Bool"("DisabledEnum"=T2."Enabled" ("Disabled")) -> ()  [unwired: 2 in, 2 out]
            n990 = property on="Y Scan Velocity SP steps/sec" class="DigNum (strict)"("DisabledEnum"=T2."Enabled" ("Disabled")) -> ()  [unwired: 2 in, 2 out]
            n991 = property on="Y Scan set" class="Bool"("DisabledEnum"=T2."Enabled" ("Disabled")) -> ()  [unwired: 2 in, 2 out]
            n992 = property on="Y Scan OK" class="Bool"("DisabledEnum"=T2."Enabled" ("Disabled")) -> ()  [unwired: 2 in, 2 out]
            n993 = property on="Y Scan Length SP steps" class="DigNum (strict)"("DisabledEnum"=T2."Enabled" ("Disabled")) -> ()  [unwired: 2 in, 2 out]
          }
        }
        n994 = flat-sequence {
          tunnel: [w1798] -> w1766
          tunnel: [w1797] -> w1765
          tunnel: w1764 -> [w1795]
          tunnel: w1763 -> [w1794]
          tunnel: [w1805] -> w1761
          tunnel: [w1806] -> w1762
          tunnel: w1766 -> [w1806]
          tunnel: w1765 -> [w1805]
          frame #0 {
            n995 = call "mDrive Send Command.vi"("error in (no error)"=w1794, "Command"=T1."Stop", "VISA resource name"=w1795) -> ("error out"=w1797:errorcluster, "VISA resource name out"=w1798:refnum<visa-resource-name>)  [unwired: 4 in, 1 out]
          }
          frame #1 {
            n996 = property on="Z Scan" class="Bool (strict)"("Value"=FALSE ("Slew Ready")) -> ()  [unwired: 2 in, 2 out]
            n997 = property on="Z Scan set" class="Bool"("DisabledEnum"=T2."Enabled" ("Disabled")) -> ()  [unwired: 2 in, 2 out]
            n998 = property on="Z Scan Velocity SP steps/sec" class="DigNum (strict)"("DisabledEnum"=T2."Enabled" ("Disabled")) -> ()  [unwired: 2 in, 2 out]
            n999 = property on="Z Scan Length SP steps" class="DigNum (strict)"("DisabledEnum"=T2."Enabled" ("Disabled")) -> ()  [unwired: 2 in, 2 out]
            n1000 = property on="Z Go" class="Bool"("DisabledEnum"=T2."Enabled" ("Disabled")) -> ()  [unwired: 2 in, 2 out]
            n1001 = property on="Z Scan OK" class="Bool"("DisabledEnum"=T2."Enabled" ("Disabled")) -> ()  [unwired: 2 in, 2 out]
          }
        }
        n1002 = flat-sequence {
          tunnel: [w1785] -> w1760
          tunnel: [w1784] -> w1759
          tunnel: w1758 -> [w1782]
          tunnel: w1757 -> [w1781]
          tunnel: [w1792] -> w1755
          tunnel: [w1793] -> w1756
          tunnel: w1760 -> [w1793]
          tunnel: w1759 -> [w1792]
          frame #0 {
            n1003 = call "mDrive Send Command.vi"("error in (no error)"=w1781, "Command"=T1."Stop", "VISA resource name"=w1782) -> ("error out"=w1784:errorcluster, "VISA resource name out"=w1785:refnum<visa-resource-name>)  [unwired: 4 in, 1 out]
          }
          frame #1 {
            n1004 = property on="R Scan" class="Bool (strict)"("Value"=FALSE ("Slew Ready")) -> ()  [unwired: 2 in, 2 out]
            n1005 = property on="R Scan Velocity SP steps/sec" class="DigNum (strict)"("DisabledEnum"=T2."Enabled" ("Disabled")) -> ()  [unwired: 2 in, 2 out]
            n1006 = property on="R Go" class="Bool"("DisabledEnum"=T2."Enabled" ("Disabled")) -> ()  [unwired: 2 in, 2 out]
            n1007 = property on="R Scan OK" class="Bool"("DisabledEnum"=T2."Enabled" ("Disabled")) -> ()  [unwired: 2 in, 2 out]
            n1008 = property on="R Scan Length SP steps" class="DigNum (strict)"("DisabledEnum"=T2."Enabled" ("Disabled")) -> ()  [unwired: 2 in, 2 out]
            n1009 = property on="R Scan set" class="Bool"("DisabledEnum"=T2."Enabled" ("Disabled")) -> ()  [unwired: 2 in, 2 out]
          }
        }
        n1010 = property on="Scan Go" class="Bool"("DisabledEnum"=T2."Disabled and Grayed Out" ("Disabled")) -> ()  [unwired: 2 in, 2 out]
        n1011 = property on="Scan Cancel" class="Bool"("DisabledEnum"=T2."Disabled and Grayed Out" ("Disabled")) -> ()  [unwired: 2 in, 2 out]
      }
      event #23 {
        n1012 = event-data() -> ()  [unwired: 1 in, 7 out]
        n1013 = flat-sequence {
          tunnel: [w1912] -> w1895
          tunnel: [w1911] -> w1888
          tunnel: [w1906] -> w1885
          tunnel: [w1910] -> w1884
          tunnel: [w1909] -> w1883
          tunnel: [w1908] -> w1882
          tunnel: [w1907] -> w1881
          tunnel: w1860 -> [w1896]
          tunnel: [w1897] -> w1859
          tunnel: w1858 -> [w1898]
          tunnel: [w1899] -> w1857
          tunnel: w1856 -> [w1905]
          tunnel: [w1905] -> w1855
          tunnel: w1854 -> [w1904]
          tunnel: [w1904] -> w1853
          tunnel: w1852 -> [w1903]
          tunnel: [w1903] -> w1851
          tunnel: w1850 -> [w1902]
          tunnel: [w1902] -> w1849
          tunnel: [w1901] -> w1848
          tunnel: w1847 -> [w1901]
          tunnel: [w1900] -> w1846
          tunnel: w1845 -> [w1900]
          tunnel: [w1965] -> w1892
          tunnel: [w1964] -> w1890
          tunnel: w1895 -> [w1963]
          tunnel: w1888 -> [w1962]
          tunnel: [w1962] -> w1886
          tunnel: w1885 -> [w1951]
          tunnel: w1884 -> [w1961]
          tunnel: w1883 -> [w1957]
          tunnel: w1882 -> [w1954]
          tunnel: w1881 -> [w1960]
          tunnel: [w1959] -> w1879
          tunnel: [w1958] -> w1877
          tunnel: [w1957] -> w1874
          tunnel: [w1956] -> w1872
          tunnel: [w1955] -> w1870
          tunnel: [w1954] -> w1868
          tunnel: [w1953] -> w1866
          tunnel: [w1952] -> w1864
          tunnel: [w1951] -> w1863
          tunnel: w1859 -> [w1950]
          tunnel: w1857 -> [w1949]
          tunnel: w1855 -> [w1948]
          tunnel: w1853 -> [w1947]
          tunnel: w1851 -> [w1946]
          tunnel: w1849 -> [w1945]
          tunnel: w1848 -> [w1944]
          tunnel: w1846 -> [w1943]
          tunnel: w1892 -> [w2003]
          tunnel: [w2003] -> w1891
          tunnel: w1890 -> [w2002]
          tunnel: [w2002] -> w1889
          tunnel: [w2000] -> w1887
          tunnel: w1886 -> [w2000]
          tunnel: [w1999] -> w1880
          tunnel: w1879 -> [w1999]
          tunnel: [w1998] -> w1878
          tunnel: w1877 -> [w1998]
          tunnel: [w1997] -> w1876
          tunnel: [w1996] -> w1875
          tunnel: w1874 -> [w1996]
          tunnel: [w1995] -> w1873
          tunnel: w1872 -> [w1995]
          tunnel: [w1994] -> w1871
          tunnel: w1870 -> [w1994]
          tunnel: [w1993] -> w1869
          tunnel: w1868 -> [w1993]
          tunnel: [w1992] -> w1867
          tunnel: w1866 -> [w1992]
          tunnel: [w1991] -> w1865
          tunnel: w1864 -> [w1991]
          tunnel: w1863 -> [w1997]
          tunnel: w1891 -> [w2023]
          tunnel: [w2021] -> w1894
          tunnel: w1889 -> [w2022]
          tunnel: [w2020] -> w1893
          tunnel: w1887 -> [w2019]
          tunnel: w1880 -> [w2018]
          tunnel: w1878 -> [w2017]
          tunnel: w1876 -> [w2016]
          tunnel: w1875 -> [w2015]
          tunnel: w1873 -> [w2014]
          tunnel: w1871 -> [w2013]
          tunnel: w1869 -> [w2012]
          tunnel: w1867 -> [w2011]
          tunnel: w1865 -> [w2010]
          tunnel: [w2009] -> w1862
          tunnel: [w2008] -> w1861
          tunnel: [w2007] -> w1840
          tunnel: [w2006] -> w1837
          tunnel: [w2005] -> w1835
          tunnel: [w2004] -> w1833
          tunnel: w1894 -> [w2081]
          tunnel: w1893 -> [w2080]
          tunnel: [w2081] -> w1844
          tunnel: [w2080] -> w1843
          tunnel: [w2074] -> w1842
          tunnel: w1862 -> [w2074]
          tunnel: [w2073] -> w1841
          tunnel: w1861 -> [w2073]
          tunnel: w1840 -> [w2063]
          tunnel: [w2063] -> w1839
          tunnel: [w2062] -> w1838
          tunnel: w1837 -> [w2062]
          tunnel: [w2061] -> w1836
          tunnel: w1835 -> [w2061]
          tunnel: [w2060] -> w1834
          tunnel: w1833 -> [w2060]
          frame #0 {
            n1014 = property on="X Scan" class="Bool (strict)"() -> ("Value"=w1906:bool)  [unwired: 2 in, 2 out]
            n1015 = property on="Y Scan" class="Bool (strict)"() -> ("Value"=w1911:bool)  [unwired: 2 in, 2 out]
            n1016 = property on="Z Scan" class="Bool (strict)"() -> ("Value"=w1908:bool)  [unwired: 2 in, 2 out]
            n1017 = property on="R Scan" class="Bool (strict)"() -> ("Value"=w1909:bool)  [unwired: 2 in, 2 out]
            n1018 = case shown="True" w1906 {
              tunnel: w1898 -> [w1928 w1932]
              tunnel: [w1928 w1931] -> w1899
              tunnel: w1896 -> [w1927 w1930]
              tunnel: [w1927 w1929] -> w1897
              frame #0 {
              }
              frame #1 {
                n1019 = property on="X Scan Length SP steps" class="DigNum (strict)"() -> ("Value"=w1933:i32)  [unwired: 2 in, 2 out]
                n1020 = Number To Decimal String(number=w1933) -> (decimal integer string=w1934:string)  [unwired: 1 in]
                n1021 = call "Applied Send Command.vi"("error in (no error)"=w1932, "Extra"=w1934, "Command"=T3."Distance or Position", "VISA resource name"=w1930) -> ("error out"=w1931:errorcluster, "VISA resource name out"=w1929:refnum<visa-resource-name>)  [unwired: 3 in, 1 out]
              }
            }
            n1022 = case shown="True" w1911 {
              tunnel: ["" w1937] -> w1912
              frame #0 {
              }
              frame #1 {
                n1023 = property on="Y Scan Length SP steps" class="DigNum (strict)"() -> ("Value"=w1942:i32)  [unwired: 2 in, 2 out]
                n1024 = Number To Decimal String(number=w1942) -> (decimal integer string=w1939:string)  [unwired: 1 in]
                n1025 = call <vilib>:"Space Constant.vi"() -> ("String"=w1940:string)
                n1026 = Concatenate Strings("MR", w1940, w1939, "\r") -> (w1937:string)
              }
            }
            n1027 = case shown="True" w1908 {
              tunnel: ["" w1921] -> w1910
              frame #0 {
              }
              frame #1 {
                n1028 = property on="Z Scan Length SP steps" class="DigNum (strict)"() -> ("Value"=w1926:i32)  [unwired: 2 in, 2 out]
                n1029 = Number To Decimal String(number=w1926) -> (decimal integer string=w1923:string)  [unwired: 1 in]
                n1030 = call <vilib>:"Space Constant.vi"() -> ("String"=w1924:string)
                n1031 = Concatenate Strings("MR", w1924, w1923, "\r") -> (w1921:string)
              }
            }
            n1032 = case shown="True" w1909 {
              tunnel: ["" w1914] -> w1907
              frame #0 {
              }
              frame #1 {
                n1033 = property on="R Scan Length SP steps" class="DigNum (strict)"() -> ("Value"=w1919:i32)  [unwired: 2 in, 2 out]
                n1034 = Number To Decimal String(number=w1919) -> (decimal integer string=w1916:string)  [unwired: 1 in]
                n1035 = call <vilib>:"Space Constant.vi"() -> ("String"=w1917:string)
                n1036 = Concatenate Strings("MR", w1917, w1916, "\r") -> (w1914:string)
              }
            }
          }
          frame #1 {
            n1037 = case shown="True" w1951 {
              tunnel: [w1981 w1983] -> w1959
              tunnel: [w1980 w1982] -> w1958
              tunnel: w1950 -> [w1981 w1983]
              tunnel: w1949 -> [w1980 w1982]
              frame #0 {
              }
              frame #1 {
              }
            }
            n1038 = case shown="False" w1962 {
              tunnel: [w1985 w1990] -> w1965
              tunnel: [w1984 w1989] -> w1964
              tunnel: w1963 -> [_ w1988]
              tunnel: w1948 -> [w1985 w1987]
              tunnel: w1947 -> [w1984 w1986]
              frame #0 {
              }
              frame #1 {
                n1039 = VISA Write(VISA resource name=w1987, write buffer=w1988, error in (no error)=w1986) -> (VISA resource name out=w1990:refnum<visa-resource-name>, error out=w1989:errorcluster)  [unwired: 1 out]
              }
            }
            n1040 = case shown="False" w1954 {
              tunnel: [w1974 w1979] -> w1953
              tunnel: [w1973 w1978] -> w1952
              tunnel: w1961 -> [_ w1977]
              tunnel: w1946 -> [w1974 w1976]
              tunnel: w1945 -> [w1973 w1975]
              frame #0 {
              }
              frame #1 {
                n1041 = VISA Write(VISA resource name=w1976, write buffer=w1977, error in (no error)=w1975) -> (VISA resource name out=w1979:refnum<visa-resource-name>, error out=w1978:errorcluster)  [unwired: 1 out]
              }
            }
            n1042 = case shown="False" w1957 {
              tunnel: [w1967 w1972] -> w1956
              tunnel: [w1966 w1971] -> w1955
              tunnel: w1960 -> [_ w1970]
              tunnel: w1944 -> [w1967 w1969]
              tunnel: w1943 -> [w1966 w1968]
              frame #0 {
              }
              frame #1 {
                n1043 = VISA Write(VISA resource name=w1969, write buffer=w1970, error in (no error)=w1968) -> (VISA resource name out=w1972:refnum<visa-resource-name>, error out=w1971:errorcluster)  [unwired: 1 out]
              }
            }
          }
          frame #2 {
            n1044 = call "Time Delay7"("Delay Time (s)"=0.1) -> ()  [unwired: 10 in, 1 out]
          }
          frame #3 {
            n1045 = case shown="True" w2016 {
              tunnel: w2018 -> [w2043 w2047]
              tunnel: w2017 -> [w2042 w2046]
              tunnel: [w2043 w2045] -> w2005
              tunnel: [w2042 w2044] -> w2004
              frame #0 {
              }
              frame #1 {
                n1046 = property class="Instr"(reference=w2047, error in=w2046) -> (reference out=w2049:refnum<visa-resource-name>, error out=w2048:errorcluster, "Serial Settings:Number of Bytes at Serial Port"=w2050:u32)
                n1047 = VISA Read(VISA resource name=w2049, byte count=w2050, error in (no error)=w2048) -> (VISA resource name out=w2045:refnum<visa-resource-name>, error out=w2044:errorcluster)  [unwired: 2 out]
              }
            }
            n1048 = case shown="True" w2019 {
              tunnel: w2023 -> [w2052 w2056]
              tunnel: w2022 -> [w2051 w2055]
              tunnel: [w2052 w2054] -> w2021
              tunnel: [w2051 w2053] -> w2020
              frame #0 {
              }
              frame #1 {
                n1049 = property class="Instr"(reference=w2056, error in=w2055) -> (reference out=w2058:refnum<visa-resource-name>, error out=w2057:errorcluster, "Serial Settings:Number of Bytes at Serial Port"=w2059:u32)
                n1050 = VISA Read(VISA resource name=w2058, byte count=w2059, error in (no error)=w2057) -> (VISA resource name out=w2054:refnum<visa-resource-name>, error out=w2053:errorcluster)  [unwired: 2 out]
              }
            }
            n1051 = case shown="True" w2012 {
              tunnel: w2011 -> [w2025 w2029]
              tunnel: w2010 -> [w2024 w2028]
              tunnel: [w2025 w2027] -> w2009
              tunnel: [w2024 w2026] -> w2008
              frame #0 {
              }
              frame #1 {
                n1052 = property class="Instr"(reference=w2029, error in=w2028) -> (reference out=w2031:refnum<visa-resource-name>, error out=w2030:errorcluster, "Serial Settings:Number of Bytes at Serial Port"=w2032:u32)
                n1053 = VISA Read(VISA resource name=w2031, byte count=w2032, error in (no error)=w2030) -> (VISA resource name out=w2027:refnum<visa-resource-name>, error out=w2026:errorcluster)  [unwired: 2 out]
              }
            }
            n1054 = case shown="True" w2015 {
              tunnel: w2014 -> [w2034 w2038]
              tunnel: w2013 -> [w2033 w2037]
              tunnel: [w2034 w2036] -> w2007
              tunnel: [w2033 w2035] -> w2006
              frame #0 {
              }
              frame #1 {
                n1055 = property class="Instr"(reference=w2038, error in=w2037) -> (reference out=w2040:refnum<visa-resource-name>, error out=w2039:errorcluster, "Serial Settings:Number of Bytes at Serial Port"=w2041:u32)
                n1056 = VISA Read(VISA resource name=w2040, byte count=w2041, error in (no error)=w2039) -> (VISA resource name out=w2036:refnum<visa-resource-name>, error out=w2035:errorcluster)  [unwired: 2 out]
              }
            }
          }
          frame #4 {
            n1057 = property on="R Scan" class="Bool (strict)"("Val(Sgnl)"=FALSE ("Slew Ready 2")) -> ()  [unwired: 2 in, 2 out]
            n1058 = property on="Z Scan" class="Bool (strict)"("Val(Sgnl)"=FALSE ("Slew Ready 2")) -> ()  [unwired: 2 in, 2 out]
            n1059 = property on="X Scan" class="Bool (strict)"("Val(Sgnl)"=FALSE ("Slew Ready 2")) -> ()  [unwired: 2 in, 2 out]
            n1060 = property on="Y Scan" class="Bool (strict)"("Val(Sgnl)"=FALSE ("Slew Ready 2")) -> ()  [unwired: 2 in, 2 out]
            n1061 = property on="Z Scan Velocity SP steps/sec" class="DigNum (strict)"("DisabledEnum"=T2."Enabled" ("Disabled")) -> ()  [unwired: 2 in, 2 out]
            n1062 = property on="X Scan Length SP steps" class="DigNum (strict)"("DisabledEnum"=T2."Enabled" ("Disabled")) -> ()  [unwired: 2 in, 2 out]
            n1063 = property on="Y Scan Selocity SP steps/sec" class="DigNum (strict)"("DisabledEnum"=T2."Enabled" ("Disabled")) -> ()  [unwired: 2 in, 2 out]
            n1064 = property on="Z Scan Length SP steps" class="DigNum (strict)"("DisabledEnum"=T2."Enabled" ("Disabled")) -> ()  [unwired: 2 in, 2 out]
            n1065 = property on="Y Scan Length SP steps" class="DigNum (strict)"("DisabledEnum"=T2."Enabled" ("Disabled")) -> ()  [unwired: 2 in, 2 out]
            n1066 = property on="X Scan Velocity SP steps/sec" class="DigNum (strict)"("DisabledEnum"=T2."Enabled" ("Disabled")) -> ()  [unwired: 2 in, 2 out]
            n1067 = property on="R Scan Velocity SP steps/sec" class="DigNum (strict)"("DisabledEnum"=T2."Enabled" ("Disabled")) -> ()  [unwired: 2 in, 2 out]
            n1068 = property on="R Scan Length SP steps" class="DigNum (strict)"("DisabledEnum"=T2."Enabled" ("Disabled")) -> ()  [unwired: 2 in, 2 out]
            n1069 = property on="Scan Go" class="Bool"("DisabledEnum"=T2."Disabled and Grayed Out" ("Disabled")) -> ()  [unwired: 2 in, 2 out]
            n1070 = property on="Scan Cancel" class="Bool"("DisabledEnum"=T2."Disabled and Grayed Out" ("Disabled")) -> ()  [unwired: 2 in, 2 out]
          }
        }
      }
      event #24 {
        n1071 = event-data() -> ()  [unwired: 1 in, 7 out]
        n1072 = flat-sequence {
          tunnel: [w2112] -> w2091
          tunnel: w2092 -> [w2114]
          tunnel: [w2113] -> w2090
          tunnel: w2093 -> [w2115]
          frame #0 {
            n1073 = property on="Reset X Motor Steps" class="DigNum (strict)"() -> ("Value"=w2118:i32)  [unwired: 2 in, 2 out]
            n1074 = Number To Decimal String(number=w2118) -> (decimal integer string=w2116:string)  [unwired: 1 in]
            n1075 = call "Applied Send Command.vi"("error in (no error)"=w2114, "Extra"=w2116, "Command"=T3."Set ABS Position", "VISA resource name"=w2115) -> ("error out"=w2113:errorcluster, "VISA resource name out"=w2112:refnum<visa-resource-name>)  [unwired: 3 in, 1 out]
          }
        }
        n1076 = flat-sequence {
          tunnel: w2097 -> [w2122]
          tunnel: w2096 -> [w2121]
          tunnel: [w2120] -> w2095
          tunnel: [w2119] -> w2094
          frame #0 {
            n1077 = property on="Reset Y Motor Steps" class="DigNum (strict)"() -> ("Value"=w2123:i32)  [unwired: 2 in, 2 out]
            n1078 = Number To Decimal String(number=w2123) -> (decimal integer string=w2124:string)  [unwired: 1 in]
            n1079 = call "mDrive Send Command.vi"("error in (no error)"=w2121, "Extra"=w2124, "Command"=T1."Set Current Position", "VISA resource name"=w2122) -> ("error out"=w2119:errorcluster, "VISA resource name out"=w2120:refnum<visa-resource-name>)  [unwired: 3 in, 1 out]
          }
        }
        n1080 = flat-sequence {
          tunnel: [w2099] -> w2085
          tunnel: [w2101] -> w2084
          tunnel: w2087 -> [w2100]
          tunnel: w2086 -> [w2098]
          frame #0 {
            n1081 = property on="Reset R Motor Steps" class="DigNum (strict)"() -> ("Value"=w2102:i32)  [unwired: 2 in, 2 out]
            n1082 = Number To Decimal String(number=w2102) -> (decimal integer string=w2103:string)  [unwired: 1 in]
            n1083 = call "mDrive Send Command.vi"("error in (no error)"=w2098, "Extra"=w2103, "Command"=T1."Set Current Position", "VISA resource name"=w2100) -> ("error out"=w2101:errorcluster, "VISA resource name out"=w2099:refnum<visa-resource-name>)  [unwired: 3 in, 1 out]
          }
        }
        n1084 = flat-sequence {
          tunnel: [w2108] -> w2083
          tunnel: [w2107] -> w2082
          tunnel: w2089 -> [w2106]
          tunnel: w2088 -> [w2105]
          frame #0 {
            n1085 = property on="Reset Z Motor Steps" class="DigNum (strict)"() -> ("Value"=w2109:i32)  [unwired: 2 in, 2 out]
            n1086 = Number To Decimal String(number=w2109) -> (decimal integer string=w2110:string)  [unwired: 1 in]
            n1087 = call "mDrive Send Command.vi"("error in (no error)"=w2105, "Extra"=w2110, "Command"=T1."Set Current Position", "VISA resource name"=w2106) -> ("error out"=w2107:errorcluster, "VISA resource name out"=w2108:refnum<visa-resource-name>)  [unwired: 3 in, 1 out]
          }
        }
      }
    }
    n1088 = case shown="True" "Set Button" {
      tunnel: "Preset positions" -> [_ w470]
      frame #0 {
      }
      frame #1 {
        n1089 = property on="Presets" class="Arr (strict)"() -> ("Value"=w467:i32[][])  [unwired: 2 in, 2 out]
        n1090 = Index Array(array=w467, index (row)=w470) -> (element=w469:i32[])  [unwired: 1 in]
        n1091 = Array To Cluster(array=w469) -> (cluster=w468:T5)
        n1092 = Unbundle(w468) -> ("Value[0]"=w466:i32, "Value[1]"=w465:i32, "Value[2]"=w464:i32, "Value[3]"=w463:i32)  [unwired: 5 out]
        n1093 = property on="X Step SP" class="DigNum (strict)"("Val(Sgnl)"=w466) -> ()  [unwired: 2 in, 2 out]
        n1094 = property on="Y Step SP" class="DigNum (strict)"("Val(Sgnl)"=w465) -> ()  [unwired: 2 in, 2 out]
        n1095 = property on="Z Step SP" class="DigNum (strict)"("Val(Sgnl)"=w464) -> ()  [unwired: 2 in, 2 out]
        n1096 = property on="R Step SP" class="DigNum (strict)"("Val(Sgnl)"=w463) -> ()  [unwired: 2 in, 2 out]
      }
    }
    n1097 = case shown="True" "Add Button" {
      tunnel: w427 -> [_ w462]
      frame #0 {
      }
      frame #1 {
        n1098 = property on="X Step PV" class="DigNum (strict)"() -> ("Value"=w457:i32)  [unwired: 2 in, 2 out]
        n1099 = property on="Y Step PV" class="DigNum (strict)"() -> ("Value"=w456:i32)  [unwired: 2 in, 2 out]
        n1100 = property on="Z Step PV" class="DigNum (strict)"() -> ("Value"=w455:i32)  [unwired: 2 in, 2 out]
        n1101 = property on="R Step PV" class="DigNum (strict)"() -> ("Value"=w454:i32)  [unwired: 2 in, 2 out]
        n1102 = Build Array(w457, w456, w455, w454) -> (w460:i32[])
        n1103 = Build Array (concatenate)(w462, "String") -> (w461:string[])
        n1104 = property on="Preset positions" class="Ring (strict)"("Strings []"=w461) -> ()  [unwired: 2 in, 2 out]
        n1105 = property on="Presets" class="Arr (strict)"() -> ("Value"=w459:i32[][])  [unwired: 2 in, 2 out]
        n1106 = Build Array (concatenate)(w459, w460) -> (w453:i32[][])
        n1107 = property on="Presets" class="Arr (strict)"("Val(Sgnl)"=w453) -> ()  [unwired: 2 in, 2 out]
      }
    }
    n1108 = case shown="True" "Delete Button" {
      tunnel: w427 -> [_ w452]
      frame #0 {
      }
      frame #1 {
        n1109 = property on="Preset positions" class="Ring (strict)"() -> ("Value"=w450:i32)  [unwired: 2 in, 2 out]
        n1110 = property on="Presets" class="Arr (strict)"() -> ("Value"=w449:i32[][])  [unwired: 2 in, 2 out]
        n1111 = Delete From Array(array=w452, index=w450) -> (array with subset deleted=w451:string[])  [unwired: 1 in, 1 out]
        n1112 = property on="Preset positions" class="Ring (strict)"("Strings []"=w451) -> ()  [unwired: 2 in, 2 out]
        n1113 = Delete From Array(array=w449, index (row)=w450) -> (array with subset deleted=w448:i32[][])  [unwired: 2 in, 1 out]
        n1114 = property on="Presets" class="Arr (strict)"("Val(Sgnl)"=w448) -> ()  [unwired: 2 in, 2 out]
      }
    }
  }
  n1115 = flat-sequence {
    tunnel: w86 -> [w2127]
    tunnel: w85 -> [w2126]
    tunnel: [w2138] -> w28
    frame #0 {
      # "GET CURRENT POSITION"
      n1116 = call "Applied Send Command.vi"("error in (no error)"=w2126, "Extra"="", "Command"=T3."Immediate Position?", "VISA resource name"=w2127) -> ("error out"=w2128:errorcluster, "read buffer"=w2133:string, "VISA resource name out"=w2129:refnum<visa-resource-name>)  [unwired: 3 in]
      n1117 = call "Applied Send Command.vi"("error in (no error)"=w2128, "Command"=T3."Stop & Kill Buffer", "VISA resource name"=w2129) -> ("error out"=w2135:errorcluster, "VISA resource name out"=w2136:refnum<visa-resource-name>)  [unwired: 4 in, 1 out]
      n1118 = VISA Close(VISA resource name=w2136, error in (no error)=w2135) -> ()  [unwired: 1 out]
      n1119 = Hexadecimal String To Number(string=w2133, offset=3) -> (number=w2130:u32)  [unwired: 1 in, 1 out]
      n1120 = To Long Integer(number=w2130) -> (32bit integer=w2138:i32)
    }
  }
  n1121 = flat-sequence {
    tunnel: w32 -> [w2144]
    tunnel: w31 -> [w2142]
    tunnel: [w2139] -> w27
    frame #0 {
      n1122 = call "mDrive Send Command.vi"("error in (no error)"=w2142, "Extra"="P", "Command"=T1."Print Parameter", "VISA resource name"=w2144) -> ("error out"=w2141:errorcluster, "read buffer"=w2148:string, "VISA resource name out"=w2143:refnum<visa-resource-name>)  [unwired: 3 in]
      n1123 = call "mDrive Send Command.vi"("error in (no error)"=w2141, "Command"=T1."Stop", "VISA resource name"=w2143) -> ("error out"=w2150:errorcluster, "VISA resource name out"=w2151:refnum<visa-resource-name>)  [unwired: 4 in, 1 out]
      n1124 = Decimal String To Number(string=w2148, offset=0) -> (number=w2140:i32)  [unwired: 1 in, 1 out]
      n1125 = To Long Integer(number=w2140) -> (32bit integer=w2139:i32)
      n1126 = VISA Close(VISA resource name=w2151, error in (no error)=w2150) -> ()  [unwired: 1 out]
    }
  }
  n1127 = flat-sequence {
    tunnel: w34 -> [w2157]
    tunnel: w33 -> [w2155]
    tunnel: [w2152] -> w26
    frame #0 {
      n1128 = call "mDrive Send Command.vi"("error in (no error)"=w2155, "Extra"="P", "Command"=T1."Print Parameter", "VISA resource name"=w2157) -> ("error out"=w2154:errorcluster, "read buffer"=w2161:string, "VISA resource name out"=w2156:refnum<visa-resource-name>)  [unwired: 3 in]
      n1129 = call "mDrive Send Command.vi"("error in (no error)"=w2154, "Command"=T1."Stop", "VISA resource name"=w2156) -> ("error out"=w2163:errorcluster, "VISA resource name out"=w2164:refnum<visa-resource-name>)  [unwired: 4 in, 1 out]
      n1130 = Decimal String To Number(string=w2161, offset=0) -> (number=w2153:i32)  [unwired: 1 in, 1 out]
      n1131 = To Long Integer(number=w2153) -> (32bit integer=w2152:i32)
      n1132 = VISA Close(VISA resource name=w2164, error in (no error)=w2163) -> ()  [unwired: 1 out]
    }
  }
  n1133 = flat-sequence {
    tunnel: w30 -> [w2170]
    tunnel: w29 -> [w2168]
    tunnel: [w2165] -> w25
    frame #0 {
      n1134 = call "mDrive Send Command.vi"("error in (no error)"=w2168, "Extra"="P", "Command"=T1."Print Parameter", "VISA resource name"=w2170) -> ("error out"=w2167:errorcluster, "read buffer"=w2174:string, "VISA resource name out"=w2169:refnum<visa-resource-name>)  [unwired: 3 in]
      n1135 = call "mDrive Send Command.vi"("error in (no error)"=w2167, "Command"=T1."Stop", "VISA resource name"=w2169) -> ("error out"=w2176:errorcluster, "VISA resource name out"=w2177:refnum<visa-resource-name>)  [unwired: 4 in, 1 out]
      n1136 = Decimal String To Number(string=w2174, offset=0) -> (number=w2166:i32)  [unwired: 1 in, 1 out]
      n1137 = To Long Integer(number=w2166) -> (32bit integer=w2165:i32)
      n1138 = VISA Close(VISA resource name=w2177, error in (no error)=w2176) -> ()  [unwired: 1 out]
    }
  }
  n1139 = flat-sequence {
    tunnel: w28 -> [w2183]
    tunnel: w27 -> [w2182]
    tunnel: w26 -> [w2181]
    tunnel: w25 -> [w2180]
    frame #0 {
      n1140 = Build Array(w2183, w2182, w2181, w2180) -> (w2178:i32[])
      n1141 = call-poly <vilib>:"Write To Spreadsheet File.vi"("1D data"=w2178, "file path (dialog if empty)"=path "S:/LV codes/SCL2/POS.TXT") -> ()  [unwired: 6 in, 1 out]
    }
    frame #1 {
      n1142 = property on="Presets" class="Arr (strict)"() -> ("Value"=w2190:i32[][])  [unwired: 2 in, 2 out]
      n1143 = property on="Preset positions" class="Ring (strict)"() -> ("Strings []"=w2186:string[])  [unwired: 2 in, 2 out]
      n1144 = Number To Decimal String(number=w2190) -> (decimal integer string=w2184:string[][])  [unwired: 1 in]
      n1145 = Transpose 2D Array(2D array=w2184) -> (transposed array=w2185:string[][])
      n1146 = Build Array (concatenate)(w2186, w2185) -> (w2187:string[][])
      n1147 = Transpose 2D Array(2D array=w2187) -> (transposed array=w2188:string[][])
      n1148 = call-poly <vilib>:"Write To Spreadsheet File.vi"("2D data"=w2188, "file path (dialog if empty)"=path "S:/LV codes/SCL2/PRESET.TXT") -> ()  [unwired: 6 in, 1 out]
    }
  }
